vi "MASTER_-_Copy.vi"() -> ()   [LabVIEW 2019]
doc: "This is the interface, the one VI which loads all the others. Run this one first.\n\n(the line below ensures settings are saved)\n[Red Tweezers Save Settings]"
uses:
  subvis/line_trapping.ctl
  subvis/spot.ctl
  <vilib>/userdefined/High Color/IMAQdx.ctl
  subvis/selection_element.ctl
  <vilib>/Analysis/Matrix/Datatypes/RealMatrix.ctl
  subvis/mouse_info.ctl
  subvis/red_tweezers_globals_INTERNAL_VOLATILE.vi
  subvis/red_tweezers_globals.vi
  <vilib>/Analysis/Matrix/Numeric/Multiply/Multiply - RM,R.vi
  <vilib>/Analysis/baseanly.llb/Real A x B.vi
  <vilib>/Analysis/NI_AALBase.lvlib
  <vilib>/vision/driver/NI_Vision_Acquisition_Software.lvlib
  <vilib>/Analysis/Matrix/NI_Matrix.lvlib
  <vilib>/vision/NI_Vision_Development_Module.lvlib
panel:
  out "Objects":T1(array[cluster]) {"Aspect Ratio" format="%.2f"; "Orientation" format="%.2f"; "Area" format="%.2f"; "Object Center"."Y" format="%.2f"; "Object Center"."X" format="%.2f"}
  out "Specific Point 2":cluster{i32, i32}
  out "Specific Point":cluster{i32, i32}
  out "bottomrx 3":dbl
  out "toply 3":dbl
  out "bottomry 3":dbl
  out "toplx 3":dbl
  out "Circles 2":T2(array[cluster]) {"Position"."Y" format="%.2f"; "Position"."X" format="%.2f"}
  out "Spot Storage":T3[](array[typedef]) {"Amplitude Correction" step=0.1; "Line Trapping"."Phase Gradient" step=0.05; "Line Trapping"."Vector"."x" step=1e-06 format="%#_6p"; "Line Trapping"."Vector"."y" step=1e-06 format="%#_6p"; "Line Trapping"."Vector"."z" step=1e-06 format="%#_6p"; "NA Position"."r" step=1e-06; "NA Position"."y" step=1e-06; "NA Position"."x" step=1e-06; "Position"."z" step=1e-06; "Position"."y" step=1e-06; "Position"."x" step=1e-06; "Phase" step=0.7753; "Intensity" step=0.1}
  out "# selected":i16
  out "Last Pattern":T3[](array[typedef]) {"Amplitude Correction" step=0.1; "Line Trapping"."Phase Gradient" step=0.05; "Line Trapping"."Vector"."x" step=1e-06 format="%#_6p"; "Line Trapping"."Vector"."y" step=1e-06 format="%#_6p"; "Line Trapping"."Vector"."z" step=1e-06 format="%#_6p"; "NA Position"."r" step=1e-06; "NA Position"."y" step=1e-06; "NA Position"."x" step=1e-06; "Position"."z" step=1e-06; "Position"."y" step=1e-06; "Position"."x" step=1e-06; "Phase" step=0.7753; "Intensity" step=0.1}
  out "Plugins":T5(array[cluster])=[{"Name"="ASI Stage", "Folder"=path "C:/Users/Richard Bowman/Dropbox/red_tweezers_1_4_rc4/plugins/ASI Stage.llb", "vi reference"=refnum, "Needs to be run"=TRUE, "Error"={"status"=FALSE, "code"=0, "source"=""}}, {"Name"="iTweezers", "Folder"=path "C:/Users/Richard Bowman/Dropbox/red_tweezers_1_4_rc4/plugins/iTweezers.llb", "vi reference"=refnum, "Needs to be run"=TRUE, "Error"={"status"=FALSE, "code"=0, "source"=""}}, {"Name"="MightexLED", "Folder"=path "C:/Users/Richard Bowman/Dropbox/red_tweezers_1_4_rc4/plugins/MightexLED.llb", "vi reference"=refnum, "Needs to be run"=TRUE, "Error"={"status"=FALSE, "code"=0, "source"=""}}]
  in  "Tab":T6(tab)
  out "Possible Collision":bool
  out "Play Pressed":bool
  out "Y":dbl
  out "X":dbl
  in  "O Button":bool
  in  "OK Button":bool
  in  "Bubble Size":dbl=50.0002
  out "Hit Indicator":bool
  in  "On":bool
  out "Induce check":bool
  out "Area+ Buffer":dbl
  in  "Area to check":dbl=0.00025
  out "Prev Current Spot":dbl
  out "spots selected 2":i32=4
  out "Spot # Check":dbl
  out "Orig Y SC":dbl
  out "Orig X SC":dbl
  out "ID num check":dbl
  out "Value Check":dbl
  out "ID":dbl[](array[numeric])
  out "Null array":dbl[](array[numeric])
  out "Potential Collisions":dbl
  out "What to Check":dbl[](array[numeric])
  out "Num":dbl
  out "Old Y":dbl
  out "Old X":dbl
  out "init":dbl
  out "Looper":bool
  in  "Output to SLM":bool
  out "Maximum":dbl
  out "Projected Distance":dbl
  out "Previous Distance":dbl
  out "Group ID #":dbl
  in  "Buffer Zone":dbl=7e-05
  out "# of Spots":dbl
  out "Distance":dbl
  out "Hit":bool
  out "Y Displacement":dbl
  out "X Displacement":dbl
  out "Current Spot #":dbl
  out "spots selected":i32=4
  in  "lock aspect ratio":bool=TRUE
  in  "Size":cluster{"x":dbl, "y":dbl, "z":dbl} {"z" step=1e-06 format="%#_4p"; "y" step=1e-06 format="%#_4p"; "x" step=1e-06 format="%#_4p"}
  in  "Position":cluster{"x":dbl, "y":dbl, "z":dbl}={"x"=1e-06, "y"=-6.3e-06, "z"=0.0} {"z" step=1e-06 format="%#_4p"; "y" step=1e-06 format="%#_4p"; "x" step=1e-06 format="%#_4p"}
  in  "phase":dbl step=0.7753
  in  "Vortex Charge":i8
  in  "Intensity":dbl=1.0 step=0.1
  in  "add to selection":bool
  in  "random position":bool
  in  "new spot":bool
  in  "delete":bool
  in  "rotate":bool
  in  "Rotation Axis":u16(ring)=2 items=["Z", "X", "Y", "Custom"]
  in  "Angle (degrees)":dbl=2.0
  in  "Custom Axis":cluster{dbl, dbl, dbl}
  in  "Spot Shape":enum32{"Normal", "Line", "NA", "Mixed"}(tab)=enum."Mixed"
  in  "Line Trapping":T4 {"Phase Gradient" step=0.05; "Vector"."x" step=1e-06 format="%#_4p"; "Vector"."y" step=1e-06 format="%#_4p"; "Vector"."z" step=1e-06 format="%#_4p"}
  in  "Scale back aperture":dbl=1.1 step=0.1
  in  "Scale BA":bool
  in  "Position on back aperture":cluster{"x":dbl, "y":dbl}={"x"=-5.84327907697451e-18, "y"=0.0} {"y" step=0.1 format="%#_4p"; "x" step=0.1 format="%#_4p"}
  in  "Radius on back aperture":dbl=1.1 step=0.1
  in  "Generate":bool
  in  "Pattern":T7(tab)
  in  "Spots across centre":i32=5
  in  "Reference Array?":bool
  in  "Fraction of SLM":dbl=1.0
  in  "Spots across centre":i32=5
  in  "N":cluster{i32, i32}
  in  "spacing/m":dbl=2.0
  in  "Iterations":i32=10
  out "non-uniformity":dbl(slide)=0.031119223416512406 scale=0.0..0.2
  out "efficiency":dbl(slide)=0.8985936267644501 scale=0.0..1.0
  in  "Optimise":bool
  in  "Reset Phase/Amplitude":bool
  in  "Fall-off/m":dbl=0.00025 min=0.0 step=1e-06 format="%#_4p"
  in  "Abort Plugin":bool
  in  "Plugin:":u16(ring)=1
  in  "Save Video":bool
  in  "Global ROI (requires restart)":i32[](array[numeric])=[0, 0, 1280, 512]
  in  "Zoom":bool
  in  "Draw ROI":bool
  in  "Zoom to Fit":bool
  out "Image Information":string="640x480 1.93X 8-bit image 255    (0,0)"
  in  "Camera":T8
  in  "Time per Frame (ms)":dbl
  in  "Edit Sequence Mode":bool
  in  "Manual Edit":bool
  in  "Bubble ID to Empty":dbl
  in  "Clearance Button":bool
  in  "Manual Sequence":bool
  in  "Play Sequence":bool
  in  "Reset":bool
  out "Sequence Instances":dbl
  out "Counter":dbl
  in  "Save State":bool
  out "Sequence On?":bool
  in  "Sequence Order":dbl
  out "Selection/Group":T9[](array[typedef])
  in  "Sequence Storer":T3[][](array[typedef]) {"Amplitude Correction" step=0.1; "Line Trapping"."Phase Gradient" step=0.05; "Line Trapping"."Vector"."x" step=1e-06 format="%#_6p"; "Line Trapping"."Vector"."y" step=1e-06 format="%#_6p"; "Line Trapping"."Vector"."z" step=1e-06 format="%#_6p"; "NA Position"."r" step=1e-06; "NA Position"."y" step=1e-06; "NA Position"."x" step=1e-06; "Position"."z" step=1e-06; "Position"."y" step=1e-06; "Position"."x" step=1e-06; "Phase" step=0.7753; "Intensity" step=0.1}
  in  "New location\n ROI":bool
  out "Radius ROI x6":dbl
  out "Radius ROI y6":dbl
  out "Radius ROI y5":dbl
  out "Radius ROI x5":dbl
  out "Radius ROI y4":dbl
  out "Radius ROI x4":dbl
  out "Radius ROI y3":dbl
  out "Radius ROI x3":dbl
  out "Radius ROI x2":dbl
  out "Radius ROI y2":dbl
  out "Radius ROI y1":dbl
  out "Radius ROI x1":dbl
  out "Caging Radius \nToo Big":bool
  in  "Caging Radius":dbl
  out "ROI Point 1":T10
  out "ROI Point 0":T10
  out "ROI Point 2":T10
  in  "New Center Y":dbl
  in  "New Center X":dbl
  out "Delta x":dbl[](array[numeric])
  out "Delta y":dbl[](array[numeric])
  in  "Input New \nObject Location":bool
  out "Time Elapsed(ms)":i32
  out "Start":i32
  out "Stop":i32
  out "Insert End":bool
  out "NewXYRates":dbl[][](array[numeric])
  out "NewXYArraySize":dbl
  out "NewXYArray":dbl[][](array[numeric])
  in  "Rates":dbl
  out "LCS Y":dbl
  out "LCS X":dbl
  in  "LCS":dbl
  in  "Play":bool
  out "Initiate Creation":dbl
  in  "Max Number \nof Bubbles":dbl
  in  "Number of Planned\nSequence Frames":dbl
  in  "Add Additional Frames":bool
  in  "Frame Location":dbl
  in  "Additional Frames Wanted":dbl
  in  "Tab Control":enum32{"Line", "Arc"}(tab)
  out "X Rate":dbl
  out "Y Rate":dbl
  out "Original D-Y":dbl
  out "Original D-X":dbl
  out "Original Radius":dbl
  out "Center Location":dbl[][](array[numeric])
  out "Center X":dbl
  out "Center Y":dbl
  out "ROI Y":dbl
  out "ROI X":dbl
  out "Original Theta":dbl
  out "Degree Rate":dbl
  in  "Lock Current Spot":bool
  out "Locked Current Spot":dbl
  out "Numeric":dbl
  out "probe":dbl
  in  "Insert":bool
  in  "Start at Which Frame?":dbl
  out "Original Y":dbl
  out "Original X":dbl
  in  "Mark Original Position":bool
  in  "How Many Frames?":dbl
  out "New Y":dbl
  out "New X":dbl
  out "Spot Storage 2":T3[](array[typedef]) {"Amplitude Correction" step=0.1; "Line Trapping"."Phase Gradient" step=0.05; "Line Trapping"."Vector"."x" step=1e-06 format="%#_6p"; "Line Trapping"."Vector"."y" step=1e-06 format="%#_6p"; "Line Trapping"."Vector"."z" step=1e-06 format="%#_6p"; "NA Position"."r" step=1e-06; "NA Position"."y" step=1e-06; "NA Position"."x" step=1e-06; "Position"."z" step=1e-06; "Position"."y" step=1e-06; "Position"."x" step=1e-06; "Phase" step=0.7753; "Intensity" step=0.1}
  in  "Save":bool
  in  "Load":bool
  out "Current Y":dbl
  out "Current X":dbl
  out "Object MP Y":dbl
  out "Object MP X":dbl
  out "ROI Point 3":T10
  out "Numeric 3":dbl
  out "Numeric 2":dbl
  in  "ROI points":dbl
  out "ROI Y":dbl
  out "ROI X":dbl
  out "Center Y":dbl
  out "Center X":dbl
  in  "Camera Capture 2":bool
  out "Bubble y 2":dbl
  out "Bubble x 2":dbl
  out "Number of Matches Returned":dbl
  out "bottomry 2":dbl
  out "toply 2":dbl
  out "bottomrx 2":dbl
  out "toplx 2":dbl
  in  "Send Data":bool
  out "Camera 3":T11(plugin-control)
  in  "Circle Descriptor 2":cluster{"Min Radius":dbl, "Max Radius":dbl}={"Min Radius"=3.0, "Max Radius"=500.0}
  out "Radius":dbl
  in  "Settings":T12={"Objects"=0, "Threshold"=128, "Reject Border"=FALSE, "Fill Holes"=FALSE, "Min Object Size"=FALSE, "Min Size"=3, "Max Object Size"=FALSE, "Max Size"=100, "Show Search Area"=FALSE, "Show Center"=TRUE, "Show Bounding Box"=TRUE} {"Objects" items=["Bright Objects", "Dark Objects"]; "Threshold" min=1 max=999999999 step=1; "Max Size" min=1 max=999999999 step=1; "Min Size" min=1 max=999999999 step=1}
  out "Number of Objects":i32
  in  "ROI switch":bool
  out "# of pairs":dbl
  out "Video Frame Rate":dbl(knob)=50.00000000000003 scale=0.0..100.0 scale format="%.1f"
  out "Interface Frame Rate":dbl(knob)=97.23240312927678 scale=0.0..100.0 scale format="%.1f"
  in  "stop":bool=TRUE
  out "Step Calculation Y2":dbl
  out "Step Calculation Y1":dbl
  out "Step Calculation X2":dbl
  out "Step Calculation X1":dbl
  out "NewY2":dbl
  out "NewX2":dbl
  out "NewY1":dbl
  out "NewX1":dbl
  out "3spot Y":dbl
  out "3spot X":dbl
  out "2spot Y":dbl
  out "2spot X":dbl
  out "1spot Y":dbl
  out "1spot X":dbl
  in  "Spots":dbl
  out "ROI new Mpy":dbl
  out "ROI new MPx":dbl
  out "ROI y6":dbl
  out "ROI x6":dbl
  out "ROI y5":dbl
  out "ROI x5":dbl
  out "ROI y4":dbl
  out "ROI x4":dbl
  out "ROI y3":dbl
  out "ROI x3":dbl
  out "ROI y2":dbl
  out "ROI x2":dbl
  out "ROI y1":dbl
  out "ROI x1":dbl
  out "ROI Point 6":T10
  out "ROI point 5":T10
  out "ROI Point 4":T10
  out "MOP pressed":bool
  out "MOP pressed After":bool
  out "X Pos every 10 sec":dbl
  out "Elapsed Time":dbl
  out "Position Indicator":string
  out "Spot Checker":T3[](array[typedef]) {"Amplitude Correction" step=0.1; "Line Trapping"."Phase Gradient" step=0.05; "Line Trapping"."Vector"."x" step=1e-06 format="%#_6p"; "Line Trapping"."Vector"."y" step=1e-06 format="%#_6p"; "Line Trapping"."Vector"."z" step=1e-06 format="%#_6p"; "NA Position"."r" step=1e-06; "NA Position"."y" step=1e-06; "NA Position"."x" step=1e-06; "Position"."z" step=1e-06; "Position"."y" step=1e-06; "Position"."x" step=1e-06; "Phase" step=0.7753; "Intensity" step=0.1}
  out "Image":T11(plugin-control)
  # "Notes:\n\nIf you are doing non-sequence controls,\nthe delete function can be used as intended.\nHowever, do not use the delete function after\nrunning a sequence! Using it will prevent\nthe bubbles from appearing as the\nnumber of spots will change, which is\nessential for the sequence to work (it would\nbe displaying the maximum number of\nbubbles). \n\nIf you happen to delete a bubble, it can be \nrestored by inserting a new spot. Once enough\nspots have been restored, click on manual edit\nto correct the # of spots tracker. It should \nbe restored to where it originally was."
  # "The SLM can be used to shape spots; here you can restrict the NA of a spot (so it comes only from part of the back aperture), or create a line-trap"
  # "The traps do not have any spot-shaping applied (so they should just be diffraction-limited focal spots)."
  # "This shapes the amplitude (and phase) of the beam to create extended line traps.  The \"Phase Gradient\" control allows the Poynting vector to push things along the line.  Unfortunately, some work is needed on the scaling factors so the phase gradient control will need tweaking if the line trap has a nonzero z component."
  # "By default,each spot comes from the whole back aperture.  Here, you can limit a spot to come from a specific part of the back aperture."
  # "The control below allows you to scale the whole back aperture (i.e. the position and size of all the apertures).  It's a one-time operation, i.e. only changes things when you push \"ok\"."
  # "A Combination of line-trapping and NA restriction has been applied to these traps.  You can get at the line trap or NA parameters on the other tabs, switching to the NA tab does not delete the line-trap settings."
  # "This tab generates Shack-Hartmann type holograms, which are often useful when aligning the system, and arrays of spots."
  # "The controls above only work when using the \"IMAQdx with ROI Buttons\" case in the bottom loop.  You can save video regardless of camera code though."
  # "Manual Edit allows a user to\ngo to a specific sequence frame."
  # "To clear the sequence, you must\nclear the array. Right click on sequence\nstorer to do this."
  # "Use this to \"clear\" a \nspecific bubble. If\nworking on a sequence,\nuse this as your delete\nbutton! You can update\nthe view by using manual edit."
  # "Use the reset button\nto clear counter.\nIt becomes necessary\nwhen you clear the array,\nespecially in manual mode."
  # "Use the sequence creator tab to specify the\nnumber of bubbles you want along with\nthe number of frames.\n\nTo save at a specific interval, the sequence\norder can be used to place the state. If used\nto correct something, it will replace the\nentire sequence frame.\n\n\"Sequence On?\" is only used in auto mode."
  # "Multiple bubbles can  be done with the\nline function. One bubble at a time for the arc\nfunction."
  # "Using the Load/Save function:\n\nRed Tweezers itself is unable to save long \nsequences, but a separate program is able to\naccomplish this. To do this, follow these\nsteps:\n\n1. After creating your sequence, press the save\nbutton below.\n\n2. Then, go to the subvi folder and find\nSequenceSaver.vi.\n\n3. At the control \"Sequence Storer,\" right-click\nthe dimensions part of the array and go to\ndata operations.\n\n4. Press \"Make Current Values Default\" and save\nthe sequence.\n\n5. The next time you load the program, simply\npress load to re-acquire the sequence. You\nwill need to insert the bubbles again, but after\nthe first frame can be recovered by using\nSequenceControl.vi."
types:
  T1 = cluster{"Object Center":cluster{"X":sgl, "Y":sgl}, "Bounding Box":cluster{"X Left":i32, "Y Top":i32, "X Right":i32, "Y Bottom":i32}, "Area":sgl, "Orientation":sgl, "Aspect Ratio":sgl, "Nb Holes":i32}[]
  T2 = cluster{"Position":cluster{"X":sgl, "Y":sgl}, "Radius":dbl, "Score":dbl}[]
  T3 = typedef "spot.ctl" = cluster{"Position":cluster{"x":dbl, "y":dbl, "z":dbl}, "Intensity":dbl, "Vortex Charge":i8, "Phase":dbl, "NA Position":cluster{"x":dbl, "y":dbl, "r":dbl}, "Line Trapping":T4, "Amplitude Correction":dbl}
  T4 = typedef "line_trapping.ctl" = cluster{"Vector":cluster{"x":dbl, "y":dbl, "z":dbl}, "Phase Gradient":dbl}
  T5 = cluster{"Name":string, "Folder":path, "vi reference":refnum<vi>, "Needs to be run":bool, "Error":errorcluster}[]
  T6 = enum32{"Current Spot", "Rotate", "Spot Shape", "Patterns", "Plugins", "Video", "Sequence", "Sequence Creator", "Spot Control", "Load/Save", "Image Process"}
  T7 = enum32{"HCP Shack-Hartmann", "Square Shack-Hartmann", "Rectangular Grid"}
  T8 = typedef "IMAQdx.ctl" = refnum<k21>
  T9 = typedef "selection_element.ctl" = cluster{"Group ID":i32, "Selected":bool}
  T10 = typedef "NI_Matrix.lvlib/RealMatrix.ctl" = dbl[][]
  T11 = typedef "IMAQ Image.ctl" = refnum<image>
  T12 = cluster{"Objects":u16, "Threshold":i32, "Reject Border":bool, "Fill Holes":bool, "Min Object Size":bool, "Min Size":i32, "Max Object Size":bool, "Max Size":i32, "Show Search Area":bool, "Show Center":bool, "Show Bounding Box":bool}
  T13 = typedef "mouse_info.ctl" = cluster{"Button Down":bool, "Dragging":bool, "Position (Image Pixels)":cluster{"X":dbl, "Y":dbl}, "Previous Position (Image Pixels)":cluster{"X":dbl, "Y":dbl}, "Button":u16, "Mods":cluster{"Double Click":bool, "Menu Key":bool}, "PlatMods":cluster{"Shift":bool, "Ctrl":bool, "Alt":bool, "Cmd":bool, "Opt":bool}}
  T14 = cluster{"Desired Font (Application)":enum16{"User-specified Font", "Application Font", "System Font", "Dialog Font"}, "[User-specified Font]":cluster{"Font Name":string, "Size":i16, "Strikeout?":bool, "Italic?":bool, "Underline?":bool, "Outline?":bool, "Shadow?":bool, "Bold?":bool, "Rotation Angle":dbl}, "Horizontal Alignment":i16, "Vertical Alignment":i16}
  T15 = cluster{"Position":cluster{"x":dbl, "y":dbl, "z":dbl}, "Intensity":dbl, "Vortex Charge":i8, "Phase":dbl, "NA Position":cluster{"x":dbl, "y":dbl, "r":dbl}, "Line Trapping":T4, "Amplitude Correction":dbl}
  T16 = enum16{"Set guide visibility", "Set grid visibility", "Show front panel", "Render on image"}
  T17 = enum32{"Current Spot", "Rotate", "Spot Shape", "Patterns", "Plugins", "Video"}
  T18 = enum16{"Left Button", "Center Button", "Right Button", "Window Close"}
  T19 = typedef "Image Type" = u32
  T20 = cluster{"number: 0 to 1":dbl, "number: 0 to 1":dbl}
  T21 = typedef "overlay_element.ctl" = cluster{"Tool":enum16{"Lines", "Oval", "Rectangle", "Text"}, "Points":cluster{"X":dbl, "Y":dbl}[], "Drawing Mode":u32, "Color":u32, "String":string}
  T22 = enum32{"Current Spot", "Rotate", "Spot Shape", "Patterns", "Plugins", "Video", "Particle Tracking", "Clamping", "Blank"}[]
  T23 = typedef "LVMenuShortCut.ctl" = cluster{"include Shift key?":bool, "include Ctrl key?":bool, "shortcut key":string}
  T24 = typedef "LVPoint32TypeDef.ctl" = cluster{"Horizontal":i32, "Vertical":i32}
  T25 = cluster{"Shift":bool, "Ctrl":bool, "Alt":bool, "Cmd":bool, "Opt":bool}
  T26 = cluster{"Button Down":bool, "Dragging":bool, "Mouse Coords (image pixels)":cluster{dbl, dbl}, "Mouse Coords (image pixels)":cluster{dbl, dbl}, "Button":u16, "Mods":cluster{"Double Click":bool, "Menu Key":bool}, "PlatMods":cluster{"Shift":bool, "Ctrl":bool, "Alt":bool, "Cmd":bool, "Opt":bool}}
  T27 = cluster{"Position":cluster{"X":sgl, "Y":sgl}, "Radius":dbl, "Score":dbl}
  T28 = cluster{"Global Rectangle":i32[], "Contours":cluster{"Contour Type":u32, "ROI Type":u32, "Points":i32[]}[]}
  T29 = cluster{"Contour Type":u32, "ROI Type":u32, "Points":i32[]}[]
  T30 = cluster{"Contour Type":u32, "ROI Type":u32, "Points":i32[]}
  T31 = cluster{"[0]":dbl, "[1]":dbl, "[2]":dbl, "[3]":dbl}
  T32 = cluster{"Object Center":cluster{"X":sgl, "Y":sgl}, "Bounding Box":cluster{"X Left":i32, "Y Top":i32, "X Right":i32, "Y Bottom":i32}, "Area":sgl, "Orientation":sgl, "Aspect Ratio":sgl, "Nb Holes":i32}
  T33 = cluster{"Position":cluster{"x":dbl, "y":dbl, "z":dbl}, "Intensity":dbl, "Vortex Charge":i8, "Phase":dbl, "NA Position":cluster{"x":dbl, "y":dbl, "r":dbl}, "Line Trapping":T4, "Amplitude Correction":dbl}[]
  T34 = cluster{"NewXYArray[0]":dbl, "NewXYArray[1]":dbl, "NewXYArray[2]":dbl, "NewXYArray[3]":dbl, "NewXYArray[4]":dbl, "NewXYArray[5]":dbl, "NewXYArray[6]":dbl, "NewXYArray[7]":dbl, "NewXYArray[8]":dbl}
  T35 = cluster{"Average Frame Time":dbl, "millisecond timer value":u32}
  T36 = enum32{"Bad", "Idle", "Run top level", "Running"}
  T37 = typedef "AviRefnum.ctl" = refnum<k1>
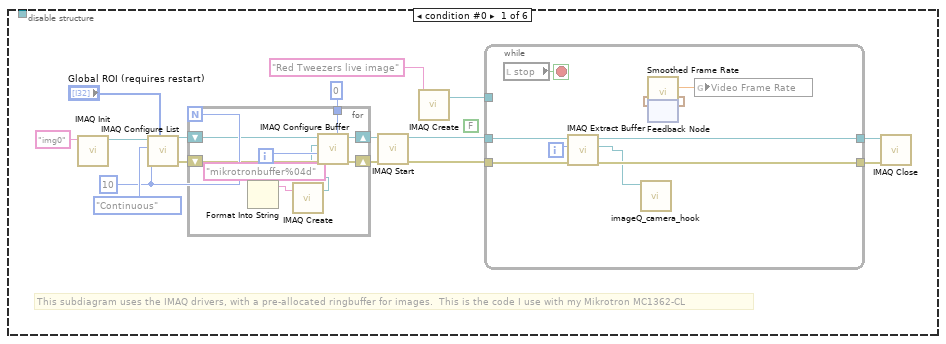
[diagram p3: hidden frame]
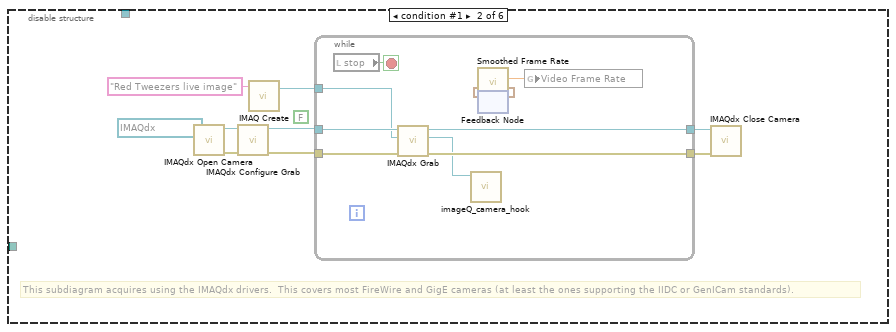
[diagram p4: hidden frame]
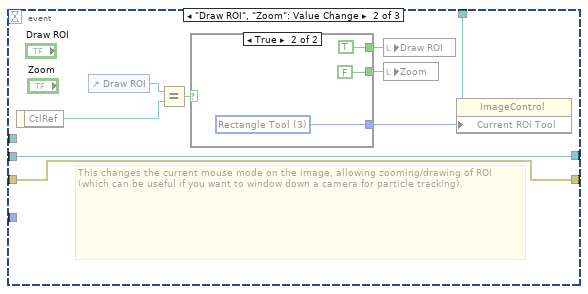
[diagram p5: hidden frame]
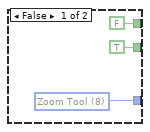
[diagram p6: hidden frame]
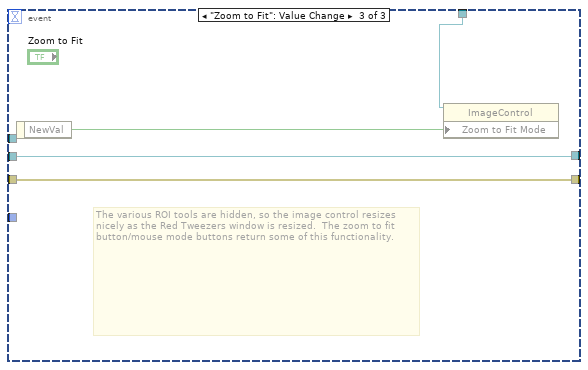
[diagram p7: hidden frame]
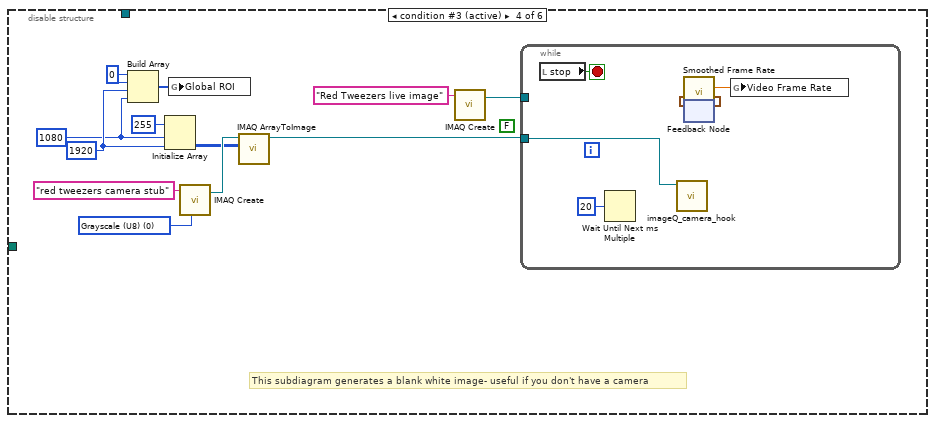
[diagram p8: hidden frame]
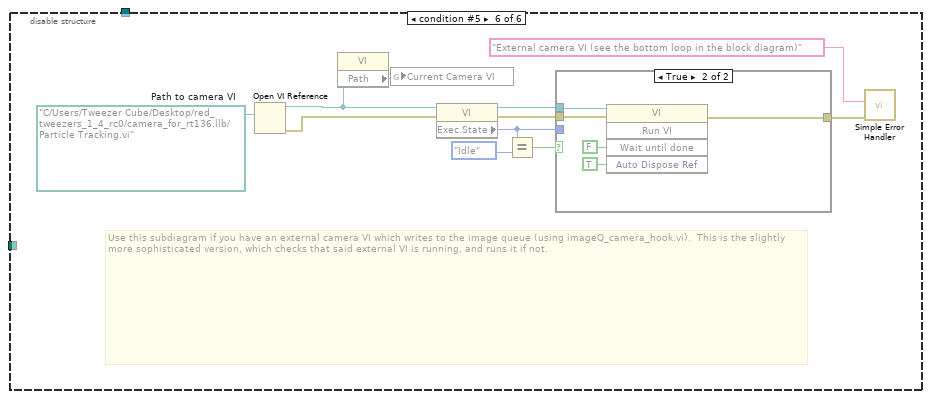
[diagram p10: hidden frame]
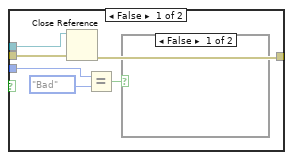
[diagram p11: hidden frame]
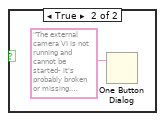
[diagram p12: hidden frame]
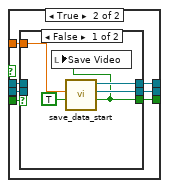
[diagram p14: hidden frame]
diagram:
  w11 = "red_tweezers_display_imageQ" ("Queue Name")
  w23 = T13 {"Button Down"=FALSE, "Dragging"=FALSE, "Position (Image Pixels)"={"X"=0.0, "Y"=0.0}, "Previous Position (Image Pixels)"={"X"=0.0, "Y"=0.0}, "Button"=0, "Mods"={"Double Click"=FALSE, "Menu Key"=FALSE}, "PlatMods"={"Shift"=FALSE, "Ctrl"=FALSE, "Alt"=FALSE, "Cmd"=FALSE, "Opt"=FALSE}}  # Mouse Information
  w24 = refnum<vi> refnum  # Image
  # "The funny looking feedback-node structure is deliberate (if odd).  We want to reload settings from the last used file (stored in the registry) only if this program has not been run since it was last loaded from file/recompiled.  That's why I use an uninitialised shift register: every time the program runs, it increments.  So, if it is zero, this is our first run (or we've been recently recompiled)."
  # "This loop handles the video that is displayed on-screen and saved to file."
  # "Initially, we only register to be told when the user clicks the image"
  # "This is the actual image control"
  # "This is a generic reference.\nIt is just a placeholder, so we can register for events later."
  # "This version of red tweezers uses two coordinate systems: \n1. Real Coordinates - corresponding to physical distances in 3D in microns\n2. Image Coordinates - position on the camera image, relative to the top left of the CURRENT ROI, measured in pixels. If the ROI changes, the relationship between \"real units\" and \"image pixels\" may change, so all values should be stored and presented to the user in REAL units unless there is a good reason to do otherwise."
  n1 = control-ref of="Plugin Pnl"() -> (w20:refnum<vi>)
  n2 = flat-sequence {
    tunnel: [w27] -> w6
    tunnel: w4 -> [_]
    frame #0 {
      n3 = vi-ref "red_tweezers_globals_INTERNAL.vi"() -> (w28:refnum<vi>)
      n4 = property class="VI"(reference=w28) -> ("Path"=w27:path)  [unwired: 1 in, 2 out]
      n5 = global write "red_tweezers_globals_INTERNAL_VOLATILE.vi" "Current Camera VI"(w27) -> ()
    }
  }
  n6 = control-ref of="Plugin:"() -> (w21:refnum<vi>)
  n7 = feedback #1() -> (w14:dbl)  [unwired: 1 in]
  n8 = Equal To 0?(x=w14) -> (x = 0?=w13:bool)
  n9 = Increment(x=w14) -> (x+1=w12:dbl)
  n10 = feedback-in #1(w12) -> ()
  n11 = call "plugins_load.vi"("Sub Panel"=w20, "Plugin Chooser"=w21) -> ("error out"=w15:errorcluster, "Plugins"=w17:T5)  [unwired: 2 in, 2 out]
  "Plugins" <- w17
  n12 = control-ref of="Image"() -> (w5:refnum<vi>)
  n13 = case shown="True" w13 {
    tunnel: w15 -> [_ w29]
    tunnel: [_ w29] -> w4
    frame False {
    }
    frame True {
      n14 = call "settings_load_default_file.vi"("error out"=w29) -> ()
    }
  }
  n15 = flat-sequence {
    tunnel: w4 -> [_]
    tunnel: w2 -> [w31]
    frame #0 {
      # "ensure we don't accidentally start saving video, and run UDP Sender to set up the hologram window."
      n16 = local write "Save Video"(FALSE ("background subtraction")) -> ()
      n17 = call "UDP Sender generic_2.vi"("Spots"=w31) -> ()  [unwired: 2 in, 1 out]
    }
  }
  n18 = global read "red_tweezers_globals.vi" "Selection/Group"() -> (w22:T9[])
  n19 = register-events(w5, w24, w24, w24) -> (reference out=w25:refnum<event-registration>)  [unwired: 2 in, 1 out]
  n20 = global read "red_tweezers_globals.vi" "Spots"() -> (w2:T3[])
  n21 = local write "stop"(FALSE ("STOP")) -> ()
  n22 = call "ensure_selection_matches_spots.vi"("Selection and Groups in"=w22, "Spots"=w2) -> ("Selection and Groups out"=w26:T9[], "Spots (duplicate)"=w1:T3[])  [unwired: 4 in]
  n23 = call "IMAQ Create"("Image Name"=w11) -> ("New Image"=w9:T11)  [unwired: 4 in, 1 out]
  n24 = call "imageQ_create_return_queue.vi"("Queue Name"=w11) -> ("queue out"=w10:refnum<queue>)
  n25 = while {
    shift-right: [w153] -> _
    shift-left: w1 -> [w173]
    shift-right: [w172] -> _
    shift-left: w26 -> [w171]
    shift-right: [w175] -> _
    shift-left: _ -> [w166]
    shift-right: [w174] -> _
    shift-left: _ -> [w165]
    tunnel: w5 -> [w170]
    shift-right: [w164] -> _
    shift-left: w23 -> [w163]
    shift-right: [w167] -> _
    shift-left: w25 -> [w168]
    border: errorcluster {"status"=FALSE, "code"=0, "source"=""} ("error out") -> [_]
    tunnel: [errorcluster {"status"=FALSE, "code"=0, "source"=""} ("error in (no error)")] -> w18
    border: w17 -> [_]
    tunnel: w1 -> [w154]
    stop <- w155 stop-if-true
    (unwired) 1 ("index")
    w72 = 7 items=["Red", "Green", "Blue", "Hue", "Saturation", "Luminance", "Value", "Intensity"] ("Color Plane")
    w74 = T19 0 items=["Grayscale (U8)", "Grayscale (I16)", "Grayscale (SGL)", "Complex (CSG)", "RGB (U32)", "HSL (U32)", "RGB (U64)", "Grayscale (U16)"] ("Image Type")
    # "Old play function that goes into case structure when\nInput New Object Location is False, using this case structure\nto prevent code from being actiivated for now"
    # "Pressing play is supposed to cause the program to\nsendcoordinates to Sequence Storer, which is\nused by SequenceControl to move the bubble, \nhowever this does not work at the moment"
    # "When done obtatining points\nKEEP it at 7!"
    # "Cycle through to obtain points"
    # "This is the calculation for the center of the detected circle, not sure where to put for now"
    # "This Play Function inserts bubbles from a given .mat file into the sequence storer"
    # "The function inserts the newly generated sequence for the automatic sequence generator. It also contains the code\nthe code necessary to check whether the bubbles will intersect with each other in the sequence."
    # "This calculates the size of the area including the buffer zone length.\nThe bubble diameter will also be included in the near future."
    # "The statement to the right controls the area that are being chcecked and checks\nwhich bubbles need to be checked.  There are two instances where this activates\nin this case:\n\nWhen a new bubble is selected\nWhen a bubble is deselected, reverting to the last current spot #\n\nThe other case, when the bubble moves out of the area specified, is located\ninside the while loop controlling the bubble movement with a mouse."
    # "Timer function example"
    # "These functions help with the calculations for the sequence generator."
    # "This loads the sequence from the \"saver\" VI. The save function below \"saves\" the sequence into the saver VI."
    # "The VI above is SequenceSaver.vi which contains the\ncode necessary to create a sequence."
    # "This case structure is the Save State structure. This stores\nthe current state of the bubbles (ie position)."
    # "Reset sets the counter back to zero. This is particularly useful \nwhen using the manual sequence."
    # "This case structure helps to continue the sequence.\nThis takes the true case of the Sequence On? function\nor the true case for the Manual Sequence function\nin order to go to the next sequence frame."
    # "This case structure allows for the playing of the sequence.\nThe amount of time it takes to go through the sequence\ncan be edited on the current spot menu."
    # "We only write to the image overlay when we are in one of the tabs, to prevent it disappearing when we are (for example) using the mouse."
    # "These wires control saving undo info. See the VI below's tip strips for details."
    # "Setting these wires to false means:\n(1) dragging moves the selection\n(2) clicking spots changes selection\nset them to true to stop the default mouse behaviour, don't wire them straight through!"
    n26 = event shown="[6] <Image>: Mouse Move" {
      selector: w168 -> [w901 w1582 w1587 w1809 w1837 w1854 w1951 _]
      dyn-events: [w901 w1581 w1587 w1807 w1834 w1855 w1951 _] -> w167
      timeout: 0 -> [_ _ _ _ _ _ _ _]
      tunnel: [w909 _ w1589 w1804 w1839 w1846 w1938 _] -> w175
      tunnel: [w908 _ w1588 w1803 w1838 w1845 w1942 _] -> w174
      tunnel: [w907 _ _ _ _ _ _ _] -> w126
      tunnel: w173 -> [w906 w1577 w1594 w1799 w1832 w1851 w1946 w2269]
      tunnel: [w905 w1577 w1592 w1799 w1832 w1842 w1944 w2269] -> w161
      tunnel: [w904 w1576 w1591 w1788 w1831 w1852 w1934 w2268] -> w160
      tunnel: w171 -> [w903 w1576 w1593 w1788 w1831 w1850 w1945 w2268]
      tunnel: w170 -> [w902 w1578 w1584 w1798 w1835 w1853 w1947 _]
      tunnel: [w900 _ w1586 w1808 T13 {"Button Down"=FALSE, "Dragging"=FALSE, "Position (Image Pixels)"={"X"=0.0, "Y"=0.0}, "Previous Position (Image Pixels)"={"X"=0.0, "Y"=0.0}, "Button"=0, "Mods"={"Double Click"=FALSE, "Menu Key"=FALSE}, "PlatMods"={"Shift"=FALSE, "Ctrl"=FALSE, "Alt"=FALSE, "Cmd"=FALSE, "Opt"=FALSE}} T13 {"Button Down"=FALSE, "Dragging"=FALSE, "Position (Image Pixels)"={"X"=0.0, "Y"=0.0}, "Previous Position (Image Pixels)"={"X"=0.0, "Y"=0.0}, "Button"=0, "Mods"={"Double Click"=FALSE, "Menu Key"=FALSE}, "PlatMods"={"Shift"=FALSE, "Ctrl"=FALSE, "Alt"=FALSE, "Cmd"=FALSE, "Opt"=FALSE}} w1950 _] -> w164
      tunnel: w163 -> [w900 _ w1586 _ _ w1849 w1941 _]
      tunnel: w166 -> [_ _ w1589 w1804 w1839 w1846 w1938 _]
      tunnel: w165 -> [_ _ w1588 w1803 w1838 w1845 w1942 _]
      tunnel: [w899 _ _ _ _ _ _ _] -> w162
      tunnel: [_ _ w1585 _ _ _ TRUE _] -> w159
      tunnel: [_ _ _ TRUE TRUE TRUE FALSE _] -> w158
      tunnel: [TRUE _ _ _ _ _ _ _] -> w156
      tunnel: [_ _ _ _ _ _ _ "stop"] -> w155
      tunnel: w154 -> [_ _ _ _ _ _ w1935 _]
      event Timeout {
        n27 = event-data() -> ()  [unwired: 1 in, 1 out]
        n28 = case shown="\"Image Process\"" "Tab" {
          tunnel: [w924 w1192 w1339 w1441 w1522 w1560 w1562 w1564 w1566 w1568 w1570] -> w905
          tunnel: w906 -> [w921 w1194 w1340 w1443 w1522 w1560 w1562 w1564 w1566 w1568 w1570]
          tunnel: w903 -> [w910 w1193 w1337 w1442 w1521 w1559 w1561 w1563 w1565 w1567 w1569]
          tunnel: [w923 w1191 w1338 w1440 w1521 w1559 w1561 w1563 w1565 w1567 w1569] -> w904
          tunnel: [w911 _ TRUE _ _ _ _ _ _ _ _] -> w909
          tunnel: [w911 _ _ _ _ _ _ _ _ _ _] -> w908
          tunnel: [_ _ _ FALSE _ _ _ _ _ _ _] -> w907
          tunnel: w902 -> [_ _ _ _ _ w1556 _ _ _ _ _]
          tunnel: w900 -> [_ _ w1319 _ _ _ _ _ _ _ _]
          tunnel: [_ _ w1321 _ _ _ _ _ _ _ _] -> w899
          frame "Current Spot", Default {
            w911 = FALSE
            # "The function below contains the code necessary to use the automatic sequence generator to create specific movements. It also helps translate cases where the point is entered in not dragged.\nThis prevents bubbles from intersecting if the bubble is told not to intersect."
            # "If it's out of date, update front panel"
            n29 = call "find_centroid.vi"("Selection and Groups"=w910, "Spots"=w921) -> ("Mean Values"=w919:T3, "size"=w913:cluster{"x":dbl, "y":dbl, "z":dbl}, "centroid"=w914:cluster{"x":dbl, "y":dbl, "z":dbl}, "# selected"=w912:i16)  [unwired: 2 in, 1 out]
            n30 = stacked-sequence {
              tunnel: w912 -> [_ w926]
              frame #0 {
                n31 = local read "spots selected"() -> (→"spots selected 2":i32)
              }
              frame #1 {
                "spots selected" <- w926
              }
            }
            n32 = feedback-in #2(w919) -> ()
            n33 = feedback #2() -> (w920:T3)  [unwired: 1 in]
            n34 = feedback #3() -> (w918:cluster{"x":dbl, "y":dbl, "z":dbl})  [unwired: 1 in]
            n35 = feedback-in #3(w913) -> ()
            n36 = Not Equal?(x=w920, y=w919) -> (x != y?=w917:bool)
            n37 = Not Equal?(x=w918, y=w913) -> (x != y?=w916:bool)
            n38 = Or(x=w917, y=w916) -> (x .or. y?=w915:bool)
            n39 = case shown="True" w915 {
              tunnel: w919 -> [_ w932]
              tunnel: w913 -> [_ w928]
              frame False {
              }
              frame True {
                n40 = Unbundle By Name(w932) -> ("Position"=w927:cluster{"x":dbl, "y":dbl, "z":dbl}, "Intensity"=w930:dbl, "Vortex Charge"=w929:i8, "Phase"=w931:dbl)
                n41 = local write "Size"(w928) -> ()
                n42 = local write "Vortex Charge"(w929) -> ()
                n43 = local write "Intensity"(w930) -> ()
                n44 = local write "Position"(w927) -> ()
                n45 = local write "phase"(w931) -> ()
                n46 = Unbundle By Name(w927) -> ()  [unwired: 2 out]
              }
            }
            n47 = local write "Selection/Group"(w910) -> ()
            n48 = event shown="[5] \"Intensity\": Value Change" {
              selector: _ -> [_ _ _ _ _ _ _ _]
              dyn-events: _ -> [_ _ _ _ _ _ _ _]
              timeout: 10 -> [_ _ _ _ _ _ _ _]
              tunnel: w921 -> [w934 w938 w952 w975 w1079 w1124 w1150 w1173]
              tunnel: w910 -> [w933 w937 w955 w982 w1066 w1121 w1147 w1171]
              tunnel: [w934 w936 w953 w974 w1067 w1122 w1148 w1172] -> w924
              tunnel: [w933 w935 w954 w982 w1066 w1121 w1147 w1171] -> w923
              tunnel: w914 -> [_ _ _ _ w1078 _ _ _]
              event Timeout {
                n49 = event-data() -> ()  [unwired: 3 out]
              }
              event "delete": Value Change {
                n50 = event-data() -> ()  [unwired: 7 out]
                n51 = call "delete_selected_spots.vi"("Selection/Group 3"=w937, "Spots 3"=w938) -> ("Selection/Group 2"=w935:T9[], "Spots 2"=w936:T3[])  [unwired: 4 in]
              }
              event "new spot": Value Change {
                # "If we're not adding it to the selection, de-select all the other spots"
                n52 = event-data() -> ()  [unwired: 7 out]
                n53 = call "coords_ROI_currentimage.vi"() -> ("Mono ROI"=w939:i32[])
                n54 = case shown="False" "add to selection" {
                  tunnel: w955 -> [w968 w973]
                  tunnel: [w967 w973] -> w950
                  frame False {
                    n55 = for {
                      tunnel: w968 -> [w971] mode=indexing
                      tunnel: [w972] -> w967 mode=indexing
                      n56 = Unbundle(w971) -> ("Group ID"=w970:i32)  [unwired: 1 out]
                      n57 = Bundle(cluster=w971, "Group ID"=w970, "Selected"=FALSE ("Label.Visible")) -> (w972:T9)
                    }
                  }
                  frame True {
                  }
                }
                n58 = Index Array(array=w939) -> (element #1=w945:i32, element #2=w946:i32, element #3=w944:i32, element #4=w943:i32)  [unwired: 4 in]
                n59 = Bundle("Numeric"=w945, "Numeric"=w946) -> (w940:cluster{"Numeric":i32, "Numeric":i32})  [unwired: 1 in]
                n60 = Bundle("Numeric"=w944, "Numeric"=w943) -> (w942:cluster{"Numeric":i32, "Numeric":i32})  [unwired: 1 in]
                n61 = Subtract(x=w942, y=w940) -> (x-y=w941:cluster{"Numeric":i32, "Numeric":i32})
                n62 = case shown="True" "random position" {
                  tunnel: [w957 w963] -> w948
                  tunnel: w941 -> [_ w959]
                  tunnel: w940 -> [_ w958]
                  frame False {
                    n63 = call "replace_position.vi"("Position"=cluster{"x":dbl, "y":dbl, "z":dbl} {"x"=0.0, "y"=0.0, "z"=0.0}) -> ("Spot"=w957:T3)  [unwired: 1 in, 2 out]
                  }
                  frame True {
                    n64 = Random Number (0-1)() -> (number: 0 to 1=w965:dbl)
                    n65 = Random Number (0-1)() -> (number: 0 to 1=w966:dbl)
                    n66 = Bundle("number: 0 to 1"=w966, "number: 0 to 1"=w965) -> (w964:T20)  [unwired: 1 out]
                    n67 = Multiply(x=w964, y=w959) -> (x*y=w961:cluster{dbl, dbl})
                    n68 = Add(x=w961, y=w958) -> (x+y=w960:cluster{dbl, dbl})
                    n69 = call "coords_image_to_real_currentimage.vi"("Position (pixels on image)"=w960) -> ("Position (real coords)"=w962:cluster{dbl, dbl, "Z":dbl})  [unwired: 9 in]
                    n70 = call "replace_position.vi"("Position"=w962) -> ("Spot"=w963:T3)  [unwired: 1 in, 2 out]
                  }
                }
                n71 = Build Array (concatenate)(w952, w948) -> (w953:T3[])
                n72 = Build Array (concatenate)(w950, cluster{i32, "Label.Visible":bool} {0, "Label.Visible"=TRUE}) -> (w954:T9[])
              }
              event "Position": Value Change {
                # "If the position has changed, translate the spots"
                n73 = event-data() -> ("OldVal"=w980:cluster{"x":dbl, "y":dbl, "z":dbl}, "NewVal"=w981:cluster{"x":dbl, "y":dbl, "z":dbl})  [unwired: 5 out]
                n74 = flat-sequence {
                  tunnel: w982 -> [w986]
                  tunnel: w979 -> [w985]
                  tunnel: w975 -> [w984]
                  tunnel: [w983] -> w976
                  frame #0 {
                    n75 = for {
                      tunnel: w984 -> [w991] mode=indexing
                      tunnel: w986 -> [w988] mode=indexing
                      tunnel: [w990] -> w983 mode=indexing
                      tunnel: w985 -> [w989]
                      n76 = Unbundle(w988) -> ("Selected"=w987:bool)  [unwired: 1 out]
                      n77 = case shown="True" w987 {
                        tunnel: w991 -> [w992 w997]
                        tunnel: [w992 w996] -> w990
                        tunnel: w989 -> [_ w993]
                        frame False {
                        }
                        frame True {
                          n78 = call "extract_position.vi"("Spot"=w997) -> ("Position"=w994:cluster{"x":dbl, "y":dbl, "z":dbl})
                          n79 = Add(x=w994, y=w993) -> (x+y=w995:cluster{"x":dbl, "y":dbl, "z":dbl})
                          n80 = call "replace_position.vi"("Position"=w995, "Spot in"=w997) -> ("Spot"=w996:T3)  [unwired: 2 out]
                        }
                      }
                    }
                  }
                }
                n81 = Subtract(x=w981, y=w980) -> (x-y=w979:cluster{"x":dbl, "y":dbl, "z":dbl})
                n82 = local read "# of Spots"() -> (w978:dbl)
                n83 = stacked-sequence {
                  tunnel: w975 -> [_ w1002 _]
                  tunnel: w976 -> [_ w1001 _]
                  tunnel: w978 -> [_ w1000 _]
                  tunnel: [_ _ w1049] -> w977
                  tunnel: w976 -> [_ _ w1048]
                  tunnel: w975 -> [_ _ w1047]
                  tunnel: [_ _ w1046] -> w974
                  frame #0 {
                    n84 = local write "Looper"(FALSE) -> ()
                    "init" <- 0
                  }
                  frame #1 {
                    n85 = for {
                      N: w1000 -> [_]
                      tunnel: w1002 -> [w1007]
                      tunnel: w1001 -> [w1012]
                      stop <- w1013 stop-if-true
                      n86 = local read "init"() -> (w1006:dbl)
                      n87 = Index Array(array=w1012, index=w1006) -> (element=w1011:T3)
                      n88 = Index Array(array=w1007, index=w1006) -> (element=w1005:T3)
                      n89 = Unbundle By Name(w1011) -> ("Position.x"=w1010:dbl, "Position.y"=w1009:dbl)
                      n90 = local read "# of Spots"() -> (w1008:dbl)
                      n91 = Unbundle By Name(w1005) -> ("Position.x"=→"Old X":dbl, "Position.y"=→"Old Y":dbl)
                      n92 = local write "New X"(w1010) -> ()
                      n93 = local write "New Y"(w1009) -> ()
                      n94 = stacked-sequence {
                        tunnel: w1007 -> [w1018 _]
                        tunnel: w1010 -> [w1017 _]
                        tunnel: w1009 -> [w1016 _]
                        tunnel: w1008 -> [w1015 _]
                        tunnel: w1006 -> [w1014 _]
                        frame #0 {
                          n95 = for {
                            N: w1015 -> [_]
                            tunnel: w1018 -> [w1040]
                            tunnel: w1017 -> [w1039]
                            tunnel: w1016 -> [w1037]
                            tunnel: w1014 -> [w1022]
                            i -> [w1024]
                            stop <- w1023 stop-if-true
                            n96 = Index Array(array=w1040, index=w1024) -> (element=w1041:T3)
                            n97 = Unbundle By Name(w1041) -> ("Position.x"=w1038:dbl, "Position.y"=w1036:dbl)
                            n98 = Subtract(x=w1039, y=w1038) -> (x-y=w1035:dbl)
                            n99 = Subtract(x=w1037, y=w1036) -> (x-y=w1034:dbl)
                            n100 = Square(x=w1035) -> (x^2=w1033:dbl)
                            n101 = Square(x=w1034) -> (x^2=w1032:dbl)
                            n102 = local read "# of Spots"() -> (w1026:dbl)
                            n103 = Add(x=w1033, y=w1032) -> (x+y=w1031:dbl)
                            n104 = local read "Buffer Zone"() -> (w1021:dbl)
                            n105 = Square Root(x=w1031) -> (sqrt(x)=w1030:dbl)
                            n106 = Multiply(x=2, y=w1021) -> (x*y=w1019:dbl)
                            n107 = Less?(x=w1030, y=w1019) -> (x < y?=w1028:bool)
                            n108 = Not Equal?(x=w1022, y=w1024) -> (x != y?=w1027:bool)
                            n109 = Equal?(x=w1026, y=w1024) -> (x = y?=w1029:bool)
                            n110 = And(x=w1027, y=w1028) -> (x .and. y?=w1025:bool)
                            "Looper" <- w1025
                            n111 = Or(x=w1025, y=w1029) -> (x .or. y?=w1023:bool)
                          }
                        }
                        frame #1 {
                          n112 = local read "Looper"() -> (w1042:bool)
                          n113 = case shown="False" w1042 {
                            frame False {
                              n114 = local read "init"() -> (w1043:dbl)
                              n115 = Add(x=w1043, y=1) -> (x+y=w1045:dbl)
                              n116 = local write "init"(w1045) -> ()
                            }
                            frame True {
                            }
                          }
                        }
                      }
                      n117 = local read "Looper"() -> (w1013:bool)
                    }
                  }
                  frame #2 {
                    n118 = local read "Looper"() -> (w1050:bool)
                    n119 = case shown="True" w1050 {
                      tunnel: w1048 -> [w1054 _]
                      tunnel: w1047 -> [_ w1062]
                      tunnel: ["This is an acceptable entry." "ERROR: A bubble will intersect the buffer zone."] -> w1049
                      tunnel: [w1054 w1062] -> w1046
                      frame False {
                        n120 = local write "Looper"(FALSE) -> ()
                        n121 = local read "Current Spot #"() -> (w1055:dbl)
                        n122 = Index Array(array=w1054, index=w1055) -> (element=w1053:T3)
                        n123 = Unbundle By Name(w1053) -> ("Position.x"=w1052:dbl, "Position.y"=w1051:dbl)
                        n124 = local write "New Y"(w1051) -> ()
                        n125 = local write "New X"(w1052) -> ()
                      }
                      frame True {
                        # "Restore original position"
                        n126 = local write "Looper"(FALSE) -> ()
                        n127 = local read "Old Y"() -> (w1059:dbl)
                        n128 = local read "Old X"() -> (w1060:dbl)
                        n129 = local read "Position"() -> (w1058:cluster{"x":dbl, "y":dbl, "z":dbl})
                        n130 = Bundle By Name(cluster=w1058, "x"=w1060, "y"=w1059) -> (w1061:cluster{"x":dbl, "y":dbl, "z":dbl})
                        n131 = local write "Position"(w1061) -> ()
                      }
                    }
                  }
                }
                "Position Indicator" <- w977
              }
              event "Size": Value Change {
                # "If we were constraining the aspect ratio, or preventing a divide by zero, the size control on the FP may be incorrect.  We refresh it in here to stop it displaying a wrong value."
                # "If the size has changed, scale the spots"
                n132 = event-data() -> ("OldVal"=w1071:cluster{"x":dbl, "y":dbl, "z":dbl}, "NewVal"=w1077:cluster{"x":dbl, "y":dbl, "z":dbl})  [unwired: 5 out]
                n133 = Not Equal?(x=w1071, y=w1077) -> (x != y?=w1070:cluster{"x":bool, "y":bool, "z":bool})
                n134 = Divide(x=w1077, y=w1071) -> (x/y=w1076:cluster{"x":dbl, "y":dbl, "z":dbl})
                n135 = Not Equal To 0?(x=w1071) -> (x != 0?=w1069:cluster{"x":bool, "y":bool, "z":bool})
                n136 = And(x=w1070, y=w1069) -> (x .and. y?=w1068:cluster{"x":bool, "y":bool, "z":bool})
                n137 = Cluster To Array(cluster=w1068) -> (array=w1075:bool[])
                n138 = Cluster To Array(cluster=w1076) -> (array=w1074:dbl[])
                n139 = case shown="True" "lock aspect ratio" {
                  tunnel: w1075 -> [w1083 w1100]
                  tunnel: w1074 -> [w1082 w1098]
                  tunnel: [w1080 w1090] -> w1073
                  frame False {
                    # "We are not constraining the aspect ratio here, so just check we're not introducing NAs"
                    n140 = for {
                      tunnel: w1083 -> [w1089] mode=indexing
                      tunnel: w1082 -> [w1085] mode=indexing
                      tunnel: [w1087] -> w1081 mode=indexing
                      n141 = Not A Number/Path/Refnum?(number/path/refnum=w1085) -> (NaN/Path/Refnum?=w1086:bool)
                      n142 = Compound Arithmetic op=AND(w1089, invert w1086) -> (w1088:bool)
                      n143 = Select(t=w1085, s=w1088, f=1.0) -> (s? t:f=w1087:dbl)
                    }
                    n144 = Array To Cluster(array=w1081) -> (cluster=w1080:cluster{"[0]":dbl, "[1]":dbl, "[2]":dbl})
                  }
                  frame True {
                    # "Pick the first element that changed and use it.  Also need to make sure (1) an element did change and (2) everything's valid (no divide by zeros)"
                    n145 = Search 1D Array(1D array=w1100, element=TRUE) -> (index of element=w1097:i32)  [unwired: 1 in]
                    n146 = Index Array(array=w1098, index=w1097) -> (element=w1093:dbl)
                    n147 = Not A Number/Path/Refnum?(number/path/refnum=w1093) -> (NaN/Path/Refnum?=w1096:bool)
                    n148 = Less Than 0?(x=w1097) -> (x < 0?=w1095:bool)
                    n149 = Or(x=w1096, y=w1095) -> (x .or. y?=w1094:bool)
                    n150 = Select(t=1.0, s=w1094, f=w1093) -> (s? t:f=w1091:dbl)
                    n151 = Bundle("x"=w1091, "x"=w1091, "x"=w1091) -> (w1090:cluster{"x":dbl, "x":dbl, "x":dbl})  [unwired: 1 in]
                  }
                }
                n152 = for {
                  tunnel: w1079 -> [w1106] mode=indexing
                  tunnel: w1066 -> [w1103] mode=indexing
                  tunnel: [w1105] -> w1067 mode=indexing
                  tunnel: w1073 -> [w1104]
                  tunnel: w1078 -> [w1101]
                  n153 = Unbundle(w1103) -> ("Selected"=w1102:bool)  [unwired: 1 out]
                  n154 = case shown="True" w1102 {
                    tunnel: w1106 -> [w1107 w1115]
                    tunnel: [w1107 w1114] -> w1105
                    tunnel: w1104 -> [_ w1113]
                    tunnel: w1101 -> [_ w1109]
                    frame False {
                    }
                    frame True {
                      n155 = call "extract_position.vi"("Spot"=w1115) -> ("Position"=w1111:cluster{"x":dbl, "y":dbl, "z":dbl})
                      n156 = Subtract(x=w1111, y=w1109) -> (x-y=w1112:cluster{"x":dbl, "y":dbl, "z":dbl})
                      n157 = Multiply(x=w1112, y=w1113) -> (x*y=w1110:cluster{"x":dbl, dbl, dbl})
                      n158 = Add(x=w1109, y=w1110) -> (x+y=w1108:cluster{"x":dbl, dbl, dbl})
                      n159 = call "replace_position.vi"("Position"=w1108, "Spot in"=w1115) -> ("Spot"=w1114:T3)  [unwired: 2 out]
                    }
                  }
                }
                n160 = call "find_centroid.vi"("Selection and Groups"=w1066, "Spots"=w1067) -> ("size"=w1065:cluster{"x":dbl, "y":dbl, "z":dbl})  [unwired: 2 in, 4 out]
                n161 = local write "Size"(w1065) -> ()
              }
              event "Intensity": Value Change {
                # "When  the user changes intensity, scale all the spots selected so the new mean is correct but keep the ratio between the selected spots.\n\nThe exception to this is when the mean intensity is zero, in which case multiplying makes no sense- in that case we just replace with the new value."
                n162 = event-data() -> ("NewVal"=w1116:dbl, "OldVal"=w1123:dbl)  [unwired: 5 out]
                n163 = Equal To 0?(x=w1123) -> (x = 0?=w1119:bool)
                n164 = Not A Number/Path/Refnum?(number/path/refnum=w1123) -> (NaN/Path/Refnum?=w1118:bool)
                n165 = Or(x=w1119, y=w1118) -> (x .or. y?=w1117:bool)
                n166 = Divide(x=w1116, y=w1123) -> (x/y=w1120:dbl)
                n167 = for {
                  tunnel: w1124 -> [w1129] mode=indexing
                  tunnel: w1121 -> [w1131] mode=indexing
                  tunnel: [w1128] -> w1122 mode=indexing
                  tunnel: w1120 -> [w1127]
                  tunnel: w1117 -> [w1126]
                  tunnel: w1116 -> [w1125]
                  n168 = Unbundle(w1131) -> ("Selected"=w1130:bool)  [unwired: 1 out]
                  n169 = case shown="True" w1130 {
                    tunnel: w1129 -> [w1132 w1139]
                    tunnel: [w1132 w1136] -> w1128
                    tunnel: w1127 -> [_ w1135]
                    tunnel: w1126 -> [_ w1134]
                    tunnel: w1125 -> [_ w1133]
                    frame False {
                    }
                    frame True {
                      n170 = Unbundle By Name(w1139) -> ("Intensity"=w1137:dbl)
                      n171 = case shown="True" w1134 {
                        tunnel: [w1142 w1143] -> w1138
                        tunnel: w1137 -> [w1141 _]
                        tunnel: w1135 -> [w1140 _]
                        tunnel: w1133 -> [_ w1143]
                        frame False {
                          n172 = Multiply(x=w1141, y=w1140) -> (x*y=w1142:dbl)
                        }
                        frame True {
                        }
                      }
                      n173 = Bundle By Name(cluster=w1139, "Intensity"=w1138) -> (w1136:T3)
                    }
                  }
                }
              }
              event "phase": Value Change {
                # "When  the user changes phase, translate the phase of all spots selectedd"
                n174 = event-data() -> ("NewVal"=w1145:dbl, "OldVal"=w1149:dbl)  [unwired: 5 out]
                n175 = Not A Number/Path/Refnum?(number/path/refnum=w1149) -> (NaN/Path/Refnum?=w1144:bool)
                n176 = Subtract(x=w1145, y=w1149) -> (x-y=w1146:dbl)
                n177 = for {
                  tunnel: w1150 -> [w1155] mode=indexing
                  tunnel: w1147 -> [w1157] mode=indexing
                  tunnel: [w1154] -> w1148 mode=indexing
                  tunnel: w1146 -> [w1153]
                  tunnel: w1144 -> [w1152]
                  tunnel: w1145 -> [w1151]
                  n178 = Unbundle(w1157) -> ("Selected"=w1156:bool)  [unwired: 1 out]
                  n179 = case shown="False" w1156 {
                    tunnel: w1155 -> [w1158 w1165]
                    tunnel: [w1158 w1162] -> w1154
                    tunnel: w1153 -> [_ w1161]
                    tunnel: w1152 -> [_ w1160]
                    tunnel: w1151 -> [_ w1159]
                    frame False {
                    }
                    frame True {
                      n180 = Unbundle By Name(w1165) -> ("Phase"=w1163:dbl)
                      n181 = case shown="False" w1160 {
                        tunnel: [w1168 w1169] -> w1164
                        tunnel: w1163 -> [w1167 _]
                        tunnel: w1161 -> [w1166 _]
                        tunnel: w1159 -> [_ w1169]
                        frame False {
                          n182 = Add(x=w1167, y=w1166) -> (x+y=w1168:dbl)
                        }
                        frame True {
                        }
                      }
                      n183 = Bundle By Name(cluster=w1165, "Phase"=w1164) -> (w1162:T3)
                    }
                  }
                }
              }
              event "Vortex Charge": Value Change {
                # "When  the user changes l, just set all selected spots to have that value of l."
                n184 = event-data() -> ("NewVal"=w1170:i8)  [unwired: 6 out]
                n185 = for {
                  tunnel: w1173 -> [w1176] mode=indexing
                  tunnel: w1171 -> [w1178] mode=indexing
                  tunnel: [w1175] -> w1172 mode=indexing
                  tunnel: w1170 -> [w1174]
                  n186 = Unbundle(w1178) -> ("Selected"=w1177:bool)  [unwired: 1 out]
                  n187 = case shown="True" w1177 {
                    tunnel: w1176 -> [w1179 w1182]
                    tunnel: [w1179 w1181] -> w1175
                    tunnel: w1174 -> [_ w1180]
                    frame False {
                    }
                    frame True {
                      n188 = Bundle By Name(cluster=w1182, "Vortex Charge"=w1180) -> (w1181:T3)
                    }
                  }
                }
              }
            }
          }
          frame "Spot Shape" {
            # "We update the spot shape tab only when spots have changed OUTSIDE this tab.  This avoids unnecessary jumping about of the tab control."
            n189 = call "find_centroid.vi"("Selection and Groups"=w1193, "Spots"=w1194) -> ("Mean Values"=w1189:T3)  [unwired: 2 in, 4 out]
            n190 = Wait (ms)(milliseconds to wait=u32 10) -> ()  [unwired: 1 out]
            n191 = call "spots_shape.vi"("Selection and Groups"=w1193, "Spots"=w1194) -> ("Spot Shape"=w1196:enum32{"Normal", "Line", "NA", "Mixed"})  [unwired: 7 in]
            n192 = feedback-in #4(w1189) -> ()
            n193 = feedback #4() -> (w1190:T3)  [unwired: 1 in]
            n194 = Not Equal?(x=w1190, y=w1189) -> (x != y?=w1195:bool)
            n195 = feedback #5() -> (w1185:enum32{"Normal", "Line", "NA", "Mixed"})  [unwired: 1 in]
            n196 = feedback #6() -> (w1187:T3)  [unwired: 1 in]
            n197 = Not Equal?(x=w1187, y=w1189) -> (x != y?=w1186:bool)
            n198 = case shown="False" w1186 {
              tunnel: w1196 -> [_ w1315]
              tunnel: ["Spot Shape" w1315] -> w1184
              frame False {
              }
              frame True {
                n199 = local write "Spot Shape"(w1315) -> ()
              }
            }
            n200 = feedback-in #5(w1184) -> ()
            n201 = Not Equal?(x=w1184, y=w1185) -> (x != y?=w1183:bool)
            n202 = case shown="\"Normal\", Default" w1184 {
              tunnel: w1194 -> [w1200 w1217 w1243 w1313]
              tunnel: w1193 -> [w1199 w1216 w1242 w1312]
              tunnel: [w1199 w1215 w1240 w1312] -> w1191
              tunnel: [w1198 w1214 w1241 w1313] -> w1192
              tunnel: w1189 -> [_ w1213 w1239 _]
              tunnel: w1195 -> [_ w1212 w1238 _]
              tunnel: w1183 -> [_ w1210 w1236 _]
              frame "Normal", Default {
                # "If \"normal\" is selected, don't allow any NA or line-trapping stuff"
                n203 = for {
                  tunnel: w1200 -> [w1203] mode=indexing
                  tunnel: w1199 -> [w1202] mode=indexing
                  tunnel: [w1204] -> w1198 mode=indexing
                  n204 = Unbundle(w1202) -> ("Selected"=w1201:bool)  [unwired: 1 out]
                  n205 = case shown="True" w1201 {
                    tunnel: [w1205 w1209] -> w1204
                    tunnel: w1203 -> [w1205 w1208]
                    frame False {
                    }
                    frame True {
                      n206 = Bundle By Name(cluster=w1208, "NA Position"=cluster{"x":dbl, "y":dbl, "r":dbl} {"x"=0.0, "y"=0.0, "r"=1.0} ("x"), "Line Trapping"=T4 {"Vector"={"x"=0.0, "y"=0.0, "z"=0.0}, "Phase Gradient"=0.0}) -> (w1209:T3)
                    }
                  }
                }
              }
              frame "Line" {
                # "If it's out of date, update front panel"
                n207 = Or(x=w1212, y=w1210) -> (x .or. y?=w1211:bool)
                n208 = case shown="True" w1211 {
                  tunnel: w1213 -> [_ w1220]
                  frame False {
                  }
                  frame True {
                    n209 = Unbundle By Name(w1220) -> ("Line Trapping"=w1219:T4)
                    n210 = local write "Line Trapping"(w1219) -> ()
                  }
                }
                n211 = event shown="[1] \"Line Trapping\": Value Change" {
                  selector: _ -> [_ _]
                  dyn-events: _ -> [_ _]
                  timeout: 10 -> [_ _]
                  tunnel: w1217 -> [w1222 w1226]
                  tunnel: w1216 -> [w1221 w1224]
                  tunnel: [w1222 w1225] -> w1214
                  tunnel: [w1221 w1224] -> w1215
                  event Timeout {
                    n212 = event-data() -> ()  [unwired: 3 out]
                  }
                  event Value Change {
                    # "If the line vector has changed, update it"
                    n213 = event-data() -> ("NewVal"=w1223:T4)  [unwired: 6 out]
                    n214 = for {
                      tunnel: w1226 -> [w1231] mode=indexing
                      tunnel: w1224 -> [w1228] mode=indexing
                      tunnel: [w1230] -> w1225 mode=indexing
                      tunnel: w1223 -> [w1229]
                      n215 = Unbundle(w1228) -> ("Selected"=w1227:bool)  [unwired: 1 out]
                      n216 = case shown="True" w1227 {
                        tunnel: w1231 -> [w1232 w1234]
                        tunnel: [w1232 w1235] -> w1230
                        tunnel: w1229 -> [_ w1233]
                        frame False {
                        }
                        frame True {
                          n217 = Bundle By Name(cluster=w1234, "Line Trapping"=w1233) -> (w1235:T3)
                        }
                      }
                    }
                  }
                }
              }
              frame "NA" {
                n218 = Or(x=w1236, y=w1238) -> (x .or. y?=w1237:bool)
                n219 = case shown="True" w1237 {
                  tunnel: w1239 -> [_ w1248]
                  frame False {
                  }
                  frame True {
                    n220 = Unbundle By Name(w1248) -> ("NA Position"=w1247:cluster{"x":dbl, "y":dbl, "r":dbl})
                    n221 = call "xyz_to_xy.vi"("Position"=w1247) -> ("Position (2D)"=w1246:cluster{"x":dbl, "y":dbl}, "z"=w1245:dbl)  [unwired: 6 out]
                    n222 = local write "Position on back aperture"(w1246) -> ()
                    n223 = local write "Radius on back aperture"(w1245) -> ()
                  }
                }
                n224 = event shown="[3] \"Scale BA\": Value Change" {
                  selector: _ -> [_ _ _ _]
                  dyn-events: _ -> [_ _ _ _]
                  timeout: 10 -> [_ _ _ _]
                  tunnel: w1243 -> [w1250 w1256 w1277 w1299]
                  tunnel: w1242 -> [w1249 w1254 w1274 w1300]
                  tunnel: [w1250 w1255 w1275 w1297] -> w1241
                  tunnel: [w1249 w1254 w1274 w1300] -> w1240
                  event Timeout {
                    n225 = event-data() -> ()  [unwired: 3 out]
                  }
                  event "Position on back aperture": Value Change {
                    # "If the position has changed, translate the spots"
                    n226 = event-data() -> ("OldVal"=w1252:cluster{"x":dbl, "y":dbl}, "NewVal"=w1253:cluster{"x":dbl, "y":dbl})  [unwired: 5 out]
                    n227 = Subtract(x=w1253, y=w1252) -> (x-y=w1251:cluster{"x":dbl, "y":dbl})
                    n228 = for {
                      tunnel: w1256 -> [w1261] mode=indexing
                      tunnel: w1254 -> [w1258] mode=indexing
                      tunnel: [w1260] -> w1255 mode=indexing
                      tunnel: w1251 -> [w1259]
                      n229 = Unbundle(w1258) -> ("Selected"=w1257:bool)  [unwired: 1 out]
                      n230 = case shown="True" w1257 {
                        tunnel: w1261 -> [w1262 w1264]
                        tunnel: [w1262 w1265] -> w1260
                        tunnel: w1259 -> [_ w1266]
                        frame False {
                        }
                        frame True {
                          n231 = Unbundle By Name(w1264) -> ("NA Position"=w1268:cluster{"x":dbl, "y":dbl, "r":dbl})
                          n232 = call "xy_to_xyz.vi"("Position (2D)"=w1266) -> ("Position (3D)"=w1267:cluster{dbl, dbl, dbl})  [unwired: 1 in, 2 out]
                          n233 = Add(x=w1268, y=w1267) -> (x+y=w1263:cluster{dbl, dbl, dbl})
                          n234 = Bundle By Name(cluster=w1264, "NA Position"=w1263) -> (w1265:T3)
                        }
                      }
                    }
                  }
                  event "Radius on back aperture": Value Change {
                    # "When  the user changes intensity, scale all the spots selected so the new mean is correct but keep the ratio between the selected spots.\n\nThe exception to this is when the mean intensity is zero, in which case multiplying makes no sense- in that case we just replace with the new value."
                    n235 = event-data() -> ("NewVal"=w1269:dbl, "OldVal"=w1276:dbl)  [unwired: 5 out]
                    n236 = Equal To 0?(x=w1276) -> (x = 0?=w1272:bool)
                    n237 = Not A Number/Path/Refnum?(number/path/refnum=w1276) -> (NaN/Path/Refnum?=w1271:bool)
                    n238 = Or(x=w1272, y=w1271) -> (x .or. y?=w1270:bool)
                    n239 = Divide(x=w1269, y=w1276) -> (x/y=w1273:dbl)
                    n240 = for {
                      tunnel: w1277 -> [w1282] mode=indexing
                      tunnel: w1274 -> [w1284] mode=indexing
                      tunnel: [w1281] -> w1275 mode=indexing
                      tunnel: w1273 -> [w1280]
                      tunnel: w1270 -> [w1279]
                      tunnel: w1269 -> [w1278]
                      n241 = Unbundle(w1284) -> ("Selected"=w1283:bool)  [unwired: 1 out]
                      n242 = case shown="True" w1283 {
                        tunnel: w1282 -> [w1285 w1292]
                        tunnel: [w1285 w1289] -> w1281
                        tunnel: w1280 -> [_ w1288]
                        tunnel: w1279 -> [_ w1287]
                        tunnel: w1278 -> [_ w1286]
                        frame False {
                        }
                        frame True {
                          n243 = Unbundle By Name(w1292) -> ("NA Position.r"=w1290:dbl)
                          n244 = case shown="False" w1287 {
                            tunnel: [w1295 w1296] -> w1291
                            tunnel: w1290 -> [w1294 _]
                            tunnel: w1288 -> [w1293 _]
                            tunnel: w1286 -> [_ w1296]
                            frame False {
                              n245 = Multiply(x=w1294, y=w1293) -> (x*y=w1295:dbl)
                            }
                            frame True {
                            }
                          }
                          n246 = Bundle By Name(cluster=w1292, "NA Position.r"=w1291) -> (w1289:T3)
                        }
                      }
                    }
                  }
                  event "Scale BA": Value Change {
                    n247 = event-data() -> ()  [unwired: 7 out]
                    n248 = for {
                      tunnel: w1300 -> [w1305] mode=indexing
                      tunnel: w1299 -> [w1303] mode=indexing
                      tunnel: "Scale back aperture" -> [w1302]
                      tunnel: [w1301] -> w1297 mode=indexing
                      n249 = Unbundle(w1305) -> ("Selected"=w1304:bool)  [unwired: 1 out]
                      n250 = case shown="True" w1304 {
                        tunnel: w1303 -> [w1306 w1307]
                        tunnel: w1302 -> [_ w1310]
                        tunnel: [w1306 w1308] -> w1301
                        frame False {
                        }
                        frame True {
                          n251 = Unbundle By Name(w1307) -> ("NA Position"=w1311:cluster{"x":dbl, "y":dbl, "r":dbl})
                          n252 = Multiply(x=w1310, y=w1311) -> (x*y=w1309:cluster{"x":dbl, "y":dbl, "r":dbl})
                          n253 = Bundle By Name(cluster=w1307, "NA Position"=w1309) -> (w1308:T3)
                        }
                      }
                    }
                  }
                }
              }
              frame "Mixed" {
              }
            }
            n254 = call "find_centroid.vi"("Selection and Groups"=w1191, "Spots"=w1192) -> ("Mean Values"=w1188:T3)  [unwired: 2 in, 4 out]
            n255 = feedback-in #6(w1188) -> ()
          }
          frame "Rotate" {
            w1326 = u32 0 items=["Frame", "Fill", "Highlight"] ("Drawing Mode")
            w1325 = u32 0 ("Color")
            w1322 = i16 100 ("radius")
            # "It's necessary to check this has changed to stop us unintentionally \"spinning\" the spots..."
            # "Draw the centroid as a spot, then a large circle+cross"
            # "It's important that this loop doesn't go too fast- it hogs the CPU.  However, each tab can have a different loop speed."
            n256 = Unbundle By Name(w1319) -> ("Position (Image Pixels)"=w1335:cluster{"X":dbl, "Y":dbl}, "Previous Position (Image Pixels)"=w1334:cluster{"X":dbl, "Y":dbl}, "Dragging"=w1336:bool)
            n257 = feedback-in #7(w1319) -> ()
            n258 = feedback #7() -> (w1320:T13)  [unwired: 1 in]
            n259 = call "find_centroid.vi"("Selection and Groups"=w1337, "Spots"=w1340) -> ("centroid"=w1333:cluster{"x":dbl, "y":dbl, "z":dbl})  [unwired: 2 in, 4 out]
            n260 = Not Equal?(x=w1319, y=w1320) -> (x != y?=w1317:bool)
            n261 = Wait (ms)(milliseconds to wait=u32 10) -> ()  [unwired: 1 out]
            n262 = And(x=w1317, y=w1336) -> (x .and. y?=w1318:bool)
            n263 = call "coords_real_to_image_currentview.vi"("Position (real coords)"=w1333) -> ("Position (pixels, relative to the top left of the image)"=w1316:cluster{dbl, dbl})  [unwired: 7 in, 1 out]
            n264 = case shown="True" w1318 {
              tunnel: w1340 -> [w1349 w1393]
              tunnel: [w1351 w1392] -> w1339
              tunnel: w1337 -> [w1350 w1394]
              tunnel: [w1350 w1394] -> w1338
              tunnel: w1333 -> [w1348 w1385]
              tunnel: w1335 -> [_ w1384]
              tunnel: w1334 -> [_ w1383]
              tunnel: w1316 -> [_ w1382]
              frame False {
                n265 = event shown="[1] Timeout" {
                  selector: _ -> [_ _]
                  dyn-events: _ -> [_ _]
                  timeout: 10 -> [_ _]
                  tunnel: [w1364 w1381] -> w1351
                  tunnel: w1350 -> [w1363 _]
                  tunnel: w1349 -> [w1362 w1381]
                  tunnel: w1348 -> [w1358 _]
                  event "rotate": Value Change {
                    n266 = event-data() -> ()  [unwired: 6 out]
                    n267 = case shown="3" "Rotation Axis" {
                      tunnel: [cluster{dbl, dbl, dbl} {0.0, 0.0, 1.0} ("Custom Axis") cluster{dbl, dbl, dbl} {1.0, 0.0, 0.0} ("Custom Axis") cluster{dbl, dbl, dbl} {0.0, 1.0, 0.0} ("Custom Axis") "Custom Axis"] -> w1359
                      frame 0, Default {
                        # "Z"
                      }
                      frame 1 {
                        # "X"
                      }
                      frame 2 {
                        # "Y"
                      }
                      frame 3 {
                      }
                    }
                    n268 = call "normalise_3d_vector.vi"("Vector"=w1359) -> ("Unit Vector"=w1361:cluster{dbl, dbl, dbl})  [unwired: 3 out]
                    n269 = Divide(x=6.283185307179586, y=360.0) -> (x/y=w1356:dbl)
                    n270 = Multiply(x="Angle (degrees)", y=w1356) -> (x*y=w1353:dbl)
                    n271 = call "arb_rotation_matrix.vi"("Unit Vector"=w1361, "theta"=w1353) -> ("Real Matrix"=w1365:T10)
                    n272 = for {
                      tunnel: w1363 -> [w1375] mode=indexing
                      tunnel: w1362 -> [w1370] mode=indexing
                      tunnel: [w1371] -> w1364 mode=indexing
                      tunnel: w1358 -> [w1373]
                      tunnel: w1365 -> [w1372]
                      n273 = Unbundle(w1375) -> ("Selected"=w1374:bool)  [unwired: 1 out]
                      n274 = case shown="True" w1374 {
                        tunnel: w1373 -> [_ w1380]
                        tunnel: [w1376 w1379] -> w1371
                        tunnel: w1370 -> [w1376 w1378]
                        tunnel: w1372 -> [_ w1377]
                        frame False {
                        }
                        frame True {
                          n275 = call "apply_matrix_transformation_to_spots.vi"("Transform centre (i.e. transform about this point)"=w1380, "Transformation Matrix (3x3)"=w1377, "Spot In"=w1378) -> ("Spot Out"=w1379:T3)  [unwired: 5 out]
                        }
                      }
                    }
                  }
                  event Timeout {
                    n276 = event-data() -> ()  [unwired: 4 out]
                  }
                }
              }
              frame True {
                # "if the mouse has not moved, stuff will be NaN, so let's make like a leopard and not change our spots"
                # "the magnitude of the change in our direction vector gives the rotation angle in radians"
                # "If it's within 100px of the centroid, pretend the mouse is on the surface of a sphere, and synthesize Z accordingly (z^2=100^2-x^2-y^2).  This allows rotation in 3d :)  The output should always be a unit vector."
                n277 = Build Array(w1384, w1383) -> (w1399:cluster{"X":dbl, "Y":dbl}[])
                n278 = for {
                  tunnel: w1382 -> [w1432]
                  tunnel: w1399 -> [w1428] mode=indexing
                  tunnel: [w1418] -> w1398 mode=indexing
                  n279 = Subtract(x=w1428, y=w1432) -> (x-y=w1423:cluster{dbl, dbl})
                  n280 = Divide(x=w1423, y=100.0 ("x")) -> (x/y=w1424:cluster{dbl, dbl})
                  n281 = Square(x=w1424) -> (x^2=w1431:cluster{dbl, dbl})
                  n282 = Unbundle(w1431) -> (w1429:dbl, w1430:dbl)
                  n283 = Add(x=w1429, y=w1430) -> (x+y=w1420:dbl)
                  n284 = Subtract(x=1.0, y=w1420) -> (x-y=w1426:dbl)
                  n285 = Square Root(x=w1420) -> (sqrt(x)=w1421:dbl)
                  n286 = Greater Than 0?(x=w1426) -> (x > 0?=w1427:bool)
                  n287 = case shown="False" w1427 {
                    tunnel: w1426 -> [_ w1439]
                    tunnel: [0.0 w1438] -> w1417
                    tunnel: w1424 -> [w1436 w1437]
                    tunnel: w1421 -> [w1435 _]
                    tunnel: [w1434 w1437] -> w1419
                    frame False {
                      n288 = Divide(x=w1436, y=w1435) -> (x/y=w1434:cluster{dbl, dbl})
                    }
                    frame True {
                      n289 = Square Root(x=w1439) -> (sqrt(x)=w1438:dbl)
                    }
                  }
                  n290 = call "xy_to_xyz.vi"("z"=w1417, "Position (2D)"=w1419) -> ("Position (3D)"=w1418:cluster{dbl, dbl, dbl})  [unwired: 2 out]
                }
                n291 = Index Array(array=w1398) -> (element #1=w1397:cluster{dbl, dbl, dbl}, element #2=w1388:cluster{dbl, dbl, dbl})  [unwired: 2 in]
                n292 = Add(x=w1397, y=w1388) -> (x+y=w1387:cluster{dbl, dbl, dbl})
                n293 = Subtract(x=w1397, y=w1388) -> (x-y=w1386:cluster{dbl, dbl, dbl})
                n294 = call "cross_product.vi"("b"=w1387, "a"=w1386) -> ("a cross b"=w1396:cluster{dbl, dbl, dbl})
                n295 = call "normalise_3d_vector.vi"("Vector"=w1396) -> ("Unit Vector"=w1395:cluster{dbl, dbl, dbl})  [unwired: 3 out]
                n296 = call "normalise_3d_vector.vi"("Vector"=w1386) -> ("magnitude"=w1390:dbl)  [unwired: 3 out]
                n297 = Not Equal To 0?(x=w1390) -> (x != 0?=w1389:bool)
                n298 = call "arb_rotation_matrix.vi"("Unit Vector"=w1395, "theta"=w1390) -> ("Real Matrix"=w1391:T10)
                n299 = case shown="True" w1389 {
                  tunnel: w1394 -> [_ w1405]
                  tunnel: w1393 -> [w1400 w1404]
                  tunnel: [w1400 w1403] -> w1392
                  tunnel: w1391 -> [_ w1402]
                  tunnel: w1385 -> [_ w1401]
                  frame False {
                  }
                  frame True {
                    n300 = for {
                      tunnel: w1405 -> [w1411] mode=indexing
                      tunnel: w1404 -> [w1408] mode=indexing
                      tunnel: [w1407] -> w1403 mode=indexing
                      tunnel: w1402 -> [w1409]
                      tunnel: w1401 -> [w1406]
                      n301 = Unbundle(w1411) -> ("Selected"=w1410:bool)  [unwired: 1 out]
                      n302 = case shown="True" w1410 {
                        tunnel: [w1412 w1415] -> w1407
                        tunnel: w1408 -> [w1412 w1416]
                        tunnel: w1409 -> [_ w1413]
                        tunnel: w1406 -> [_ w1414]
                        frame False {
                        }
                        frame True {
                          n303 = call "apply_matrix_transformation_to_spots.vi"("Transform centre (i.e. transform about this point)"=w1414, "Transformation Matrix (3x3)"=w1413, "Spot In"=w1416) -> ("Spot Out"=w1415:T3)  [unwired: 5 out]
                        }
                      }
                    }
                  }
                }
              }
            }
            n304 = call "coords_real_to_image_currentview.vi"("Position (real coords)"=w1333) -> ("Position (pixels, relative to the top left of the image)"=w1328:cluster{dbl, dbl}, "z (real coords)"=w1332:dbl)  [unwired: 7 in]
            n305 = expression code="z*1e7+20"(w1332) -> (w1344:dbl)
            n306 = In Range and Coerce(upper limit=100.0, x=w1344, lower limit=2.0) -> (coerced(x)=w1331:dbl)  [unwired: 1 out]
            n307 = Bundle("upper limit"=w1331, "upper limit"=w1331) -> (w1324:cluster{"upper limit":dbl, "upper limit":dbl})  [unwired: 1 in]
            n308 = call "myoverlay_oval.vi"("Color"=w1325, "Drawing Mode"=w1326, "Size"=w1324, "Centre Position (pixels on image)"=w1328) -> ("Overlay Elements Out"=w1330:T21[])  [unwired: 5 in]
            n309 = Bundle("radius"=w1322, "radius"=w1322) -> (w1323:cluster{"radius":i16, "radius":i16})  [unwired: 1 in]
            n310 = call "myoverlay_oval.vi"("Color"=w1325, "Drawing Mode"=w1326, "Size"=w1323, "Centre Position (pixels on image)"=w1328, "Overlay Elements In"=w1330) -> ("Overlay Elements Out"=w1329:T21[])  [unwired: 4 in]
            n311 = Multiply(x=w1322, y=cluster{dbl, dbl}[] [{0.0, 0.0}, {1.0, 0.0}, {0.0, 0.0}, {0.0, 1.0}, {0.0, 0.0}, {-1.0, 0.0}, {0.0, 0.0}, {0.0, -1.0}, {0.0, 0.0}]) -> (x*y=w1341:cluster{dbl, dbl}[])
            n312 = Add(x=w1328, y=w1341) -> (x+y=w1327:cluster{dbl, dbl}[])
            n313 = call "myoverlay_lines.vi"("Color"=w1325, "Drawing Mode"=w1326, "Line Endpoints"=w1327, "Overlay Elements In"=w1329) -> ("Overlay Elements Out"=w1321:T21[])  [unwired: 5 in]
          }
          frame "Patterns" {
            n314 = event shown="[3] \"Optimise\": Value Change" {
              selector: _ -> [_ _ _ _ _]
              dyn-events: _ -> [_ _ _ _ _]
              timeout: u32 10 ("milliseconds to wait") -> [_ _ _ _ _]
              tunnel: [w1458 w1488 w1492 w1495 w1506] -> w1441
              tunnel: [w1457 w1489 w1491 w1498 w1507] -> w1440
              tunnel: w1443 -> [w1456 w1488 w1492 w1496 w1505]
              tunnel: w1442 -> [w1455 w1489 w1491 w1498 w1507]
              event "Generate": Value Change {
                # "If there were previous spots, centre the pattern on the spots"
                n315 = event-data() -> ()  [unwired: 1 in, 1 out]
                n316 = call "find_centroid.vi"("Selection and Groups"=w1455, "Spots"=w1456) -> ("size"=w1451:cluster{"x":dbl, "y":dbl, "z":dbl}, "centroid"=w1447:cluster{"x":dbl, "y":dbl, "z":dbl}, "# selected"=w1453:i16)  [unwired: 2 in, 2 out]
                n317 = Greater?(x=w1453, y=i16 1) -> (0:w1448:bool)
                n318 = case shown="False" w1448 {
                  tunnel: w1451 -> [_ w1474]
                  tunnel: [cluster{"x":dbl, "y":dbl, "z":dbl} {"x"=2e-05, "y"=2e-05, "z"=2e-05} ("size") w1474] -> w1450
                  frame False {
                  }
                  frame True {
                  }
                }
                n319 = case shown="\"HCP Shack-Hartmann\"" "Pattern" {
                  tunnel: [w1476 w1479 w1485] -> w1449
                  tunnel: w1450 -> [_ w1478 _]
                  frame "Square Shack-Hartmann" {
                    n320 = call "patterns_square_shack_hartmann.vi"("N"="Spots across centre") -> ("Spots"=w1476:T3[])
                  }
                  frame "HCP Shack-Hartmann" {
                    n321 = Unbundle By Name(w1478) -> ("x"=w1477:dbl)
                    n322 = call "pattern_hcp_shack_hartmann.vi"("Width"=w1477, "Reference Array?"="Reference Array?", "Fraction of SLM"="Fraction of SLM", "N"="Spots across centre") -> ("Shack-Hartmann Spots"=w1479:T3[])  [unwired: 7 in]
                  }
                  frame "Rectangular Grid" {
                    n323 = call "patterns_rectangular_grid.vi"("spacing/m"="spacing/m", "N"="N") -> ("Spots"=w1485:T3[])
                  }
                }
                n324 = local write "Generate"(FALSE ("Generate")) -> ()
                n325 = case shown="True" w1448 {
                  tunnel: w1449 -> [w1461 w1465]
                  tunnel: w1447 -> [_ w1467]
                  tunnel: [w1461 w1463] -> w1459
                  frame False {
                  }
                  frame True {
                    n326 = call "find_centroid.vi"("Spots"=w1465) -> ("centroid"=w1466:cluster{"x":dbl, "y":dbl, "z":dbl}, "# selected"=→"# selected":i16)  [unwired: 3 in, 3 out]
                    n327 = Subtract(x=w1467, y=w1466) -> (x-y=w1464:cluster{"x":dbl, "y":dbl, "z":dbl})
                    n328 = for {
                      tunnel: w1465 -> [w1470] mode=indexing
                      tunnel: w1464 -> [w1469]
                      tunnel: [w1468] -> w1463 mode=indexing
                      n329 = call "extract_position.vi"("Spot"=w1470) -> ("Position"=w1471:cluster{"x":dbl, "y":dbl, "z":dbl})
                      n330 = Add(x=w1471, y=w1469) -> (x+y=w1472:cluster{"x":dbl, "y":dbl, "z":dbl})
                      n331 = call "replace_position.vi"("Position"=w1472, "Spot in"=w1470) -> ("Spot"=w1468:T3)  [unwired: 2 out]
                    }
                  }
                }
                "Last Pattern" <- w1459
                n332 = call "ensure_selection_matches_spots.vi"("Select All (default: no)"=TRUE ("Select All (default: true)"), "Spots"=w1459) -> ("Selection and Groups out"=w1457:T9[], "Spots (duplicate)"=w1458:T3[])  [unwired: 4 in]
              }
              event "Spots across centre", "Fraction of SLM", "Reference Array?", "N", "spacing/m", "Spots across centre": Value Change {
                n333 = event-data() -> ()  [unwired: 1 in, 1 out]
                n334 = local read "Last Pattern"() -> (w1487:T3[])
                n335 = Equal?(x=w1488, y=w1487) -> (x = y?=w1486:bool)
                n336 = case shown="True" w1486 {
                  selector: w1486 -> [_ w1490]
                  frame False {
                  }
                  frame True {
                    n337 = property on="Generate" class="Bool (strict)"("Val(Sgnl)"=w1490) -> ()  [unwired: 2 in, 2 out]
                  }
                }
              }
              event Timeout {
                n338 = event-data() -> ()  [unwired: 1 in, 1 out]
              }
              event "Optimise": Value Change {
                n339 = event-data() -> ()  [unwired: 1 in, 1 out]
                n340 = for {
                  N: "Iterations" -> [_]
                  tunnel: 203 ("Optimisation Resolution") -> [w1502]
                  shift-right: [w1503] -> w1495
                  shift-left: w1496 -> [w1504]
                  tunnel: "Fall-off/m" -> [w1499]
                  n341 = call "do_gsw_step.vi"("Optimisation Resolution"=w1502, "Sinc Zero"=w1499, "Spots In"=w1504) -> ("non-uniformity"=→"non-uniformity":dbl, "efficiency"=→"efficiency":dbl, "Spots Out"=w1503:T3[])  [unwired: 6 in]
                }
              }
              event "Reset Phase/Amplitude": Value Change {
                n342 = event-data() -> ()  [unwired: 1 in, 1 out]
                n343 = for {
                  tunnel: [w1510] -> w1506 mode=indexing
                  tunnel: w1505 -> [w1511] mode=indexing
                  n344 = Bundle By Name(cluster=w1511, "Phase"=0.0, "Amplitude Correction"=0.0) -> (w1510:T3)
                }
              }
            }
          }
          frame "Plugins" {
            # "The local variable ensures the references are  correct when they make it through to the \"close plugins\" block."
            # "This is the error from loading/unloading VIs on the front panel"
            n345 = control-ref of="Plugin Pnl"() -> (w1515:refnum<vi>)
            n346 = Wait (ms)(milliseconds to wait=u32 10) -> ()  [unwired: 1 out]
            n347 = feedback #8() -> (w1514:T5)
            n348 = feedback #9() -> (w1516:errorcluster)
            n349 = event shown="[1] \"Plugin:\": Value Change" {
              selector: _ -> [_ _ _]
              dyn-events: _ -> [_ _ _]
              timeout: 10 -> [_ _ _]
              tunnel: "Abort Plugin" -> [w1523 _ _]
              tunnel: "Plugin:" -> [w1528 _ w1544]
              tunnel: w1516 -> [w1527 w1542 w1546]
              tunnel: [w1526 w1537 w1545] -> w1517
              tunnel: [w1525 w1538 w1548] -> w1513
              tunnel: w1514 -> [w1529 w1539 w1547]
              tunnel: w1515 -> [_ w1540 _]
              event Timeout {
                n350 = event-data() -> ()  [unwired: 1 in, 2 out]
                n351 = Not(x=w1523) -> (.not. x?=w1524:bool)
                n352 = case shown="True" w1524 {
                  tunnel: w1529 -> [w1531 w1536]
                  tunnel: w1528 -> [_ w1535]
                  tunnel: w1527 -> [w1530 w1534]
                  tunnel: [w1530 w1533] -> w1526
                  tunnel: [w1531 w1532] -> w1525
                  frame False {
                  }
                  frame True {
                    n353 = call "plugins_run.vi"("Error In"=w1534, "Plugin Index"=w1535, "Plugins In"=w1536) -> ("Error Out"=w1533:errorcluster, "Plugins"=w1532:T5)  [unwired: 7 in]
                  }
                }
              }
              event "Plugin:": Value Change {
                n354 = event-data() -> ("NewVal"=w1541:u16)  [unwired: 1 in]
                n355 = call "plugins_switch.vi"("error in"=w1542, "Plugin Pnl"=w1540, "Plugin Index"=w1541, "Plugins In"=w1539) -> ("error out"=w1537:errorcluster, "Plugins Out"=w1538:T5)  [unwired: 4 in]
              }
              event "Abort Plugin": Value Change {
                n356 = event-data() -> ("NewVal"=w1543:bool)  [unwired: 1 in]
                n357 = case shown="True" w1543 {
                  tunnel: [w1550 w1555] -> w1548
                  tunnel: w1547 -> [w1550 w1554]
                  tunnel: w1546 -> [w1549 w1553]
                  tunnel: [w1549 w1552] -> w1545
                  tunnel: w1544 -> [_ w1551]
                  frame False {
                  }
                  frame True {
                    n358 = call "plugins_abort.vi"("Error In"=w1553, "Plugin Index"=w1551, "Plugins In"=w1554) -> ("Error Out"=w1552:errorcluster, "Plugins Out"=w1555:T5)  [unwired: 7 in]
                  }
                }
              }
            }
            n359 = feedback-in #8(w1513) -> ()
            n360 = feedback-in #9(w1517) -> ()
            n361 = local write "Plugins"(w1513) -> ()
          }
          frame "Video" {
            # "All the controls on this tab are in the bottom (camera) loop."
            n362 = Wait (ms)(milliseconds to wait=u32 10) -> ()  [unwired: 1 out]
            n363 = property on="Property Node" class="ImageControl"(reference=w1556) -> ("Image Information String"=→"Image Information":string)  [unwired: 1 in, 2 out]
          }
          frame "Sequence" {
          }
          frame "Sequence Creator" {
          }
          frame "Spot Control" {
          }
          frame "Load/Save" {
          }
          frame "Image Process" {
          }
        }
      }
      event "Tab": Value Change {
        w1574 = T22 [enum."Video", enum."Particle Tracking"] items=["Current Spot", "Rotate", "Spot Shape", "Patterns", "Plugins", "Video", "Particle Tracking", "Clamping", "Blank"]
        w1579 = refnum<vi> refnum  # Image
        # "This allows us to disable custom mouse-handling for certain tabs.  It can also be done from within the \"mouse down\" event case."
        n364 = event-data() -> ("NewVal"=w1575:T6)  [unwired: 1 in, 3 out]
        n365 = Equal?(x=w1574, y=w1575) -> (x = y?=w1573:bool[])
        n366 = Or Array Elements(Boolean array=w1573) -> (logical OR=w1572:bool)
        n367 = Not(x=w1572) -> (.not. x?=w1571:bool)
        n368 = Select(t=w1578, s=w1571, f=w1579) -> (s? t:f=w1580:refnum<vi>)
        n369 = register-events(reference=w1582, w1580, w1579, w1579, w1579) -> (reference out=w1581:refnum<event-registration>)  [unwired: 1 in, 1 out]
      }
      event Menu Selection (User) {
        n370 = event-data() -> ("ItemTag"=w1590:string, "MenuRef"=w1583:refnum<k9>)  [unwired: 1 in]
        n371 = case shown="\"ToggleSavingData\"" w1590 {
          tunnel: w1594 -> [w1598 w1608 w1617 w1631 w1650 w1654 w1657 w1664 w1671 w1673 w1676 w1705 w1731 w1752 w1763 w1774 w1777 w1779 w1784 w1787]
          tunnel: w1593 -> [w1597 w1607 w1616 w1640 w1649 w1653 w1655 w1662 w1670 w1672 w1675 w1704 w1730 w1751 w1762 w1773 w1776 w1780 w1785 w1786]
          tunnel: [w1598 w1608 w1617 w1631 w1648 w1651 w1657 w1664 w1671 w1673 w1676 w1705 w1731 w1752 w1763 w1774 w1777 w1779 w1784 w1787] -> w1592
          tunnel: [w1597 w1607 w1616 w1640 w1647 w1652 w1656 w1663 w1669 w1674 w1677 w1704 w1730 w1751 w1762 w1773 w1776 w1780 w1785 w1786] -> w1591
          tunnel: [_ _ _ _ TRUE _ _ _ _ _ _ _ _ _ _ _ _ _ _ _] -> w1585
          tunnel: w1584 -> [_ _ _ _ _ _ _ _ _ _ _ w1703 w1729 w1743 _ _ _ _ _ _]
          tunnel: w1583 -> [_ _ _ _ _ _ _ _ _ _ _ w1694 w1723 w1746 w1757 w1768 _ _ _ _]
          frame "ToggleSavingData" {
            # "Data is saved from the middle loop: look there for an explanation."
            n372 = local read "Save Video"() -> (w1596:bool)
            n373 = Not(x=w1596) -> (.not. x?=w1595:bool)
            n374 = local write "Save Video"(w1595) -> ()
          }
          frame "SaveStateToFile" {
            # "Save the current settings (i.e. the values of all the controls in VIs that have [Red Tweezers Save Settings] in their documentation string) to a file."
            n375 = call "File Dialog"("prompt"="Please select a location to save the settings", "button label"="Save", "default name"="red_tweezers_settings.xml", "pattern (all files)"="*.xml" ("pattern label"), "pattern label"="XML Settings Files") -> ("selected path"=w1606:path, "cancelled"=w1599:bool)  [unwired: 7 in, 2 out]
            n376 = Not(x=w1599) -> (.not. x?=w1600:bool)
            n377 = case shown="True" w1600 {
              tunnel: w1606 -> [_ w1610]
              frame False {
              }
              frame True {
                n378 = Path To String(path=w1610) -> (string=w1609:string)
                n379 = call "settings_save_to_file.vi"("XML File Path"=w1610) -> ()  [unwired: 11 in]
                n380 = call "settings_filename_to_registry.vi"("Last Used Settings File"=w1609) -> ()  [unwired: 11 in]
              }
            }
          }
          frame "SaveStateToCurrentFile" {
            # "As SaveStateToFile, but using the current file (i.e. Save not Save As...)."
            n381 = global read "red_tweezers_globals_INTERNAL_VOLATILE.vi" "Current Settings File"() -> (w1615:path)
            n382 = call <vilib>:"Check if File or Folder Exists.vi"("path"=w1615) -> ("file or folder exists?"=w1614:bool, "dup path"=w1613:path)  [unwired: 8 in, 1 out]
            n383 = case shown="True" w1614 {
              selector: w1614 -> [_ w1628]
              tunnel: w1613 -> [_ w1629]
              tunnel: [w1620 w1629] -> w1612
              tunnel: [w1621 w1628] -> w1611
              frame False {
                n384 = call "File Dialog3"("prompt"="Please select a location to save the settings", "button label"="Save", "default name"="red_tweezers_settings.xml", "pattern (all files)"="*.xml" ("pattern label"), "pattern label"="XML Settings Files") -> ("selected path"=w1620:path, "cancelled"=w1627:bool)  [unwired: 7 in, 2 out]
                n385 = Not(x=w1627) -> (.not. x?=w1621:bool)
              }
              frame True {
              }
            }
            n386 = case shown="True" w1611 {
              tunnel: w1612 -> [_ w1619]
              frame False {
              }
              frame True {
                n387 = Path To String(path=w1619) -> (string=w1618:string)
                n388 = call "settings_save_to_file.vi"("XML File Path"=w1619) -> ()  [unwired: 11 in]
                n389 = call "settings_filename_to_registry.vi"("Last Used Settings File"=w1618) -> ()  [unwired: 11 in]
              }
            }
          }
          frame "LoadStateFromFile" {
            # "Load a file, and use it to reset the values of all the front panel controls."
            # "We need to re-run the initialisation stuff in UDP sender after changing settings\n(for example, this synchronises the settings like camera pixel size with the\nrelevant global variable)"
            n390 = call "File Dialog2"("prompt"="Please select a settings file", "button label"="Open", "default name"="red_tweezers_settings.xml", "pattern (all files)"="*.xml" ("pattern label"), "pattern label"="XML Settings Files") -> ("selected path"=w1632:path, "cancelled"=w1639:bool)  [unwired: 7 in, 2 out]
            n391 = Not(x=w1639) -> (.not. x?=w1638:bool)
            n392 = case shown="False" w1638 {
              selector: w1638 -> [w1641 w1642]
              tunnel: w1632 -> [_ w1643]
              tunnel: [w1641 w1642] -> w1630
              frame False {
              }
              frame True {
                n393 = call "settings_load_from_file.vi"("XML File Path"=w1643) -> ()  [unwired: 9 in, 2 out]
                n394 = Path To String(path=w1643) -> (string=w1644:string)
                n395 = call "settings_filename_to_registry.vi"("Last Used Settings File"=w1644) -> ()  [unwired: 11 in]
              }
            }
            n396 = call "UDP Sender generic_2.vi"("re-initialise"=w1630, "Spots"=w1631) -> ()  [unwired: 1 in, 1 out]
          }
          frame "Undo" {
            # "This should get the last undo vector and replace the spots with it :)"
            n397 = call "red_tweezers_UNDO.vi"("Selection/Group"=w1649, "Undo/Store (store, False)"=TRUE, "Spots"=w1650) -> ("Selection/Group Out (Undo only)"=w1647:T9[], "Spots Out (Undo only)"=w1648:T3[])  [unwired: 7 in]
          }
          frame "Delete" {
            n398 = call "delete_selected_spots.vi"("Selection/Group 3"=w1653, "Spots 3"=w1654) -> ("Selection/Group 2"=w1652:T9[], "Spots 2"=w1651:T3[])  [unwired: 4 in]
          }
          frame "SelectAllSpots" {
            n399 = for {
              tunnel: w1655 -> [w1660] mode=indexing
              tunnel: [w1661] -> w1656 mode=indexing
              n400 = Unbundle(w1660) -> ("Group ID"=w1659:i32)  [unwired: 1 out]
              n401 = Bundle(cluster=w1660, "Group ID"=w1659, "Selected"=TRUE ("Label.Visible")) -> (w1661:T9)
            }
          }
          frame "SelectNoSpots" {
            n402 = for {
              tunnel: w1662 -> [w1667] mode=indexing
              tunnel: [w1668] -> w1663 mode=indexing
              n403 = Unbundle(w1667) -> ("Group ID"=w1666:i32)  [unwired: 1 out]
              n404 = Bundle(cluster=w1667, "Group ID"=w1666, "Selected"=FALSE ("Label.Visible")) -> (w1668:T9)
            }
          }
          frame "SelectSpecificSpots" {
            n405 = call "select_by_id.vi"("Selection/Group"=w1670, "Spots"=w1671) -> ("Selection/Group Out"=w1669:T9[])  [unwired: 9 in]
          }
          frame "Group" {
            # "Group the currently selected spots"
            n406 = call "group_selected_spots.vi"("Selection/Group 2"=w1672) -> ("Array"=w1674:T9[])
          }
          frame "Ungroup" {
            # "Ungroup the currently selected spots"
            n407 = for {
              tunnel: [w1681] -> w1677 mode=indexing
              tunnel: w1675 -> [w1680] mode=indexing
              tunnel: 0 -> [w1679]
              n408 = Unbundle(w1680) -> ("Selected"=w1682:bool)  [unwired: 1 out]
              n409 = case shown="False" w1682 {
                tunnel: [w1683 w1686] -> w1681
                tunnel: w1680 -> [w1683 w1685]
                tunnel: w1679 -> [_ w1684]
                frame False {
                }
                frame True {
                  n410 = Unbundle(w1685) -> ("Selected"=w1687:bool)  [unwired: 1 out]
                  n411 = Bundle(cluster=w1685, "Group ID"=w1684, "Selected"=w1687) -> (w1686:T9)
                }
              }
            }
          }
          frame "ZoomIn" {
            w1688 = "ZoomToFit" ("item tag")
            # "turn off \"zoom to fit\""
            n412 = property class="ImageControl"(reference=w1703) -> (reference out=w1697:refnum<vi>, "ZoomSingle"=w1702:cluster{"X":sgl, "Y":sgl}, "Image Center Position"=w1695:cluster{"X":u32, "Y":u32})  [unwired: 1 in, 1 out]
            n413 = Unbundle(w1702) -> ("X"=w1700:sgl)  [unwired: 1 out]
            n414 = Round To Nearest(number=w1700) -> (nearest integer value=w1696:sgl)
            n415 = Greater Than 0?(x=w1696) -> (x > 0?=w1701:bool)
            n416 = case shown="True" w1701 {
              tunnel: w1700 -> [w1710 w1713]
              tunnel: [w1709 w1711] -> w1699
              frame False {
                n417 = Reciprocal(x=w1710) -> (1/x=w1707:sgl)
                n418 = Round Toward +Infinity(x=w1707) -> (ceil(x): smallest int >= x=w1708:sgl)
                n419 = Decrement(x=w1708) -> (x-1=w1706:sgl)
                n420 = Reciprocal(x=w1706) -> (1/x=w1709:sgl)
              }
              frame True {
                n421 = Round Toward -Infinity(1:w1713) -> (0:w1712:sgl)
                n422 = Increment(x=w1712) -> (x+1=w1711:sgl)
              }
            }
            n423 = Bundle(w1699, w1699) -> (w1698:cluster{sgl, sgl})  [unwired: 1 in]
            n424 = property class="ImageControl"(reference=w1697, "ZoomSingle"=w1698, "Image Center Position"=w1695) -> ()  [unwired: 1 in, 2 out]
            n425 = Get Menu Item Info(7:w1688, 11:w1694) -> (1:w1691:bool, 2:w1692:string, 3:w1693:refnum<k9>, 6:w1690:T23)  [unwired: 1 in, 3 out]
            n426 = Set Menu Item Info(4:w1690, 6:FALSE ("checked"), 7:w1688, 9:w1691, 10:w1692, 11:w1693) -> ()  [unwired: 1 in, 2 out]
          }
          frame "ZoomOut" {
            w1717 = "ZoomToFit" ("item tag")
            # "turn off \"zoom to fit\""
            n427 = property class="ImageControl"(reference=w1729) -> (reference out=w1725:refnum<vi>, "ZoomSingle"=w1728:cluster{"X":sgl, "Y":sgl}, "Image Center Position"=w1724:cluster{"X":u32, "Y":u32})  [unwired: 1 in, 1 out]
            n428 = Unbundle(w1728) -> ("X"=w1714:sgl)  [unwired: 1 out]
            n429 = Greater?(x=w1714, y=1.0) -> (0:w1716:bool)
            n430 = case shown="False" w1716 {
              tunnel: w1714 -> [w1738 w1741]
              tunnel: [w1737 w1739] -> w1727
              frame False {
                n431 = Reciprocal(x=w1738) -> (1/x=w1735:sgl)
                n432 = Add(x=w1735, y=sgl 0.01 ("x")) -> (x+y=w1733:sgl)
                n433 = Round Toward -Infinity(1:w1733) -> (0:w1736:sgl)
                n434 = Increment(x=w1736) -> (x+1=w1734:sgl)
                n435 = Reciprocal(x=w1734) -> (1/x=w1737:sgl)
              }
              frame True {
                n436 = Round Toward +Infinity(x=w1741) -> (ceil(x): smallest int >= x=w1740:sgl)
                n437 = Decrement(x=w1740) -> (x-1=w1739:sgl)
              }
            }
            n438 = Bundle(w1727, w1727) -> (w1726:cluster{sgl, sgl})  [unwired: 1 in]
            n439 = property class="ImageControl"(reference=w1725, "ZoomSingle"=w1726, "Image Center Position"=w1724) -> ()  [unwired: 1 in, 2 out]
            n440 = Get Menu Item Info(7:w1717, 11:w1723) -> (1:w1720:bool, 2:w1721:string, 3:w1722:refnum<k9>, 6:w1719:T23)  [unwired: 1 in, 3 out]
            n441 = Set Menu Item Info(4:w1719, 6:FALSE ("checked"), 7:w1717, 9:w1720, 10:w1721, 11:w1722) -> ()  [unwired: 1 in, 2 out]
          }
          frame "ZoomToFit" {
            w1747 = "ZoomToFit" ("item tag")
            # "and make sure the image obeys the result"
            # "Toggle menu checkmark"
            n442 = Get Menu Item Info(7:w1747, 11:w1746) -> (1:w1745:bool, 2:w1749:string, 3:w1750:refnum<k9>, 4:w1744:bool, 6:w1748:T23)  [unwired: 1 in, 2 out]
            n443 = Not(x=w1744) -> (.not. x?=w1742:bool)
            n444 = Set Menu Item Info(4:w1748, 6:w1742, 7:w1747, 9:w1745, 10:w1749, 11:w1750) -> ()  [unwired: 1 in, 2 out]
            n445 = property class="ImageControl"(reference=w1743, "Zoom to Fit Mode"=w1742) -> ()  [unwired: 1 in, 2 out]
          }
          frame "ShowGrid" {
            w1758 = "ShowGrid" ("item tag")
            # "Toggle menu checkmark"
            n446 = Get Menu Item Info(7:w1758, 11:w1757) -> (1:w1756:bool, 2:w1760:string, 3:w1761:refnum<k9>, 4:w1755:bool, 6:w1759:T23)  [unwired: 1 in, 2 out]
            n447 = Not(x=w1755) -> (.not. x?=w1754:bool)
            n448 = Set Menu Item Info(4:w1759, 6:w1754, 7:w1758, 9:w1756, 10:w1760, 11:w1761) -> ()  [unwired: 1 in, 2 out]
            n449 = call "grid_and_guides.vi"("Boolean"=w1754, "Operation"=T16."Set grid visibility") -> ()  [unwired: 9 in, 1 out]
          }
          frame "ShowGuides" {
            w1769 = "ShowGuides" ("item tag")
            # "Toggle menu checkmark"
            n450 = Get Menu Item Info(7:w1769, 11:w1768) -> (1:w1767:bool, 2:w1771:string, 3:w1772:refnum<k9>, 4:w1766:bool, 6:w1770:T23)  [unwired: 1 in, 2 out]
            n451 = Not(x=w1766) -> (.not. x?=w1765:bool)
            n452 = Set Menu Item Info(4:w1770, 6:w1765, 7:w1769, 9:w1767, 10:w1771, 11:w1772) -> ()  [unwired: 1 in, 2 out]
            n453 = call "grid_and_guides.vi"("Boolean"=w1765, "Operation"=T16."Set guide visibility") -> ()  [unwired: 9 in, 1 out]
          }
          frame "ConfigureGridAndGuides" {
            n454 = call "grid_and_guides.vi"("Operation"=T16."Show front panel") -> ()  [unwired: 10 in, 1 out]
          }
          frame "ShowSettings" {
            n455 = call "UDP Sender generic_2.vi"("Show panel"=TRUE, "Spots"=w1779) -> ()  [unwired: 1 in, 1 out]
          }
          frame "CameraSettings" {
            n456 = global read "red_tweezers_globals_INTERNAL_VOLATILE.vi" "Current Camera VI"() -> (w1782:path)
            n457 = Open VI Reference(vi path=w1782) -> (vi reference=w1781:refnum<vi>)  [unwired: 5 in, 1 out]
            n458 = property class="VI"(reference=w1781, "Front Panel.Open"=TRUE ("Front Panel Window:Open")) -> ()  [unwired: 1 in, 2 out]
          }
          frame Default {
          }
        }
      }
      event Mouse Down? {
        # "We don't process clicks when the user is on the video tab, so that we can set ROIs."
        # "When the mouse button goes down over the image, we save where it went down, etc. and wait to see what happens next.  We also register to be told when the mouse leaves the control, goes up, or moves.  \"click\" or \"drag\" are only detected once the mouse moves or goes up."
        n459 = event-data() -> ("Coords"=w1802:T24, "Button"=w1797:u16, "Mods"=w1806:cluster{"Double Click":bool, "Menu Key":bool}, "PlatMods"=w1805:T25)  [unwired: 1 in]
        n460 = call "mouse_to_image_coords.vi"("Mouse Coords (screen/pane units)"=w1802, "Image Control"=w1798) -> ("Cursor is on Display Area"=w1796:bool, "Mouse Coords (image pixels)"=w1801:cluster{dbl, dbl})  [unwired: 4 in]
        n461 = disable-structure shown="Enabled" {
          disable-tunnel: w1797 -> [w1814 _]
          disable-tunnel: w1796 -> [w1812 w1815]
          disable-tunnel: [w1811 w1815] -> w1792
          frame Enabled {
            n462 = Equal?(x=u16 1, y=w1814) -> (x = y?=w1813:bool)
            n463 = And(x=w1812, y=w1813) -> (x .and. y?=w1811:bool)
          }
          frame Disabled {
            # "use other pane to allow right-clicking on image"
          }
        }
        n464 = local read "Tab"() -> (w1793:T6)
        n465 = Not Equal?(x=w1793, y=T17."Video" ("Tab")) -> (x != y?=w1791:bool)
        n466 = And(x=w1792, y=w1791) -> (x .and. y?=w1790:bool)
        n467 = case shown="False" w1790 {
          tunnel: w1809 -> [w1818 w1829]
          tunnel: [T13 {"Button Down"=FALSE, "Dragging"=FALSE, "Position (Image Pixels)"={"X"=0.0, "Y"=0.0}, "Previous Position (Image Pixels)"={"X"=0.0, "Y"=0.0}, "Button"=0, "Mods"={"Double Click"=FALSE, "Menu Key"=FALSE}, "PlatMods"={"Shift"=FALSE, "Ctrl"=FALSE, "Alt"=FALSE, "Cmd"=FALSE, "Opt"=FALSE}} w1828] -> w1808
          tunnel: [w1818 w1825] -> w1807
          tunnel: w1797 -> [_ w1824]
          tunnel: w1806 -> [_ w1823]
          tunnel: w1805 -> [_ w1822]
          tunnel: w1801 -> [_ w1821]
          tunnel: [FALSE TRUE] -> w1800
          tunnel: w1798 -> [_ w1819]
          frame False {
            # "If the user clicked on a scrollbar, ignore it and let LabVIEW handle it. (this keeps the scrollbars working)"
          }
          frame True {
            w1827 = FALSE  # Dragging
            w1826 = TRUE  # Button Down
            n468 = register-events(reference=w1829, w1819, w1819, w1819, w1819) -> (reference out=w1825:refnum<event-registration>)  [unwired: 1 in, 1 out]
            n469 = Bundle("Button Down"=w1826, "Dragging"=w1827, "Mouse Coords (image pixels)"=w1821, "Mouse Coords (image pixels)"=w1821, "Button"=w1824, "Mods"=w1823, "PlatMods"=w1822) -> (w1828:T26)  [unwired: 1 in]
          }
        }
        n470 = Array Size(array=w1788) -> (size(s)=w1789:i32)
        n471 = local write "Selection/Group"(w1788) -> ()
        n472 = local write "# of Spots"(w1789) -> ()
        n473 = event-data("Discard?"=w1800) -> ()  [unwired: 4 in, 1 out]
      }
      event Mouse Leave {
        w1836 = refnum<vi> refnum  # Dummy
        # "When the mouse leaves, we reset things."
        n474 = event-data() -> ()  [unwired: 1 in, 2 out]
        n475 = register-events(reference=w1837, w1835, w1836, w1836, w1836) -> (reference out=w1834:refnum<event-registration>)  [unwired: 1 in, 1 out]
      }
      event Mouse Up {
        w1856 = refnum<vi> refnum  # Dummy
        # "Double clicking adds a spot at the mouse position."
        # "deregister"
        # "If we get here the mouse has gone down and up again.  If we've not moved in between, we have a Click.\nEither way we're no longer interested in mouse leave/move/up events."
        n476 = event-data() -> ("Mods"=w1843:cluster{"Double Click":bool, "Menu Key":bool})  [unwired: 1 in, 5 out]
        n477 = Unbundle By Name(w1849) -> ("Dragging"=w1858:bool)
        n478 = Unbundle By Name(w1843) -> ("Double Click"=w1840:bool)
        n479 = Not(x=w1858) -> (.not. x?=w1857:bool)
        n480 = Not(x=w1845) -> (.not. x?=w1847:bool)
        n481 = And(x=w1857, y=w1847) -> (x .and. y?=w1841:bool)
        n482 = case shown="True" w1841 {
          tunnel: w1849 -> [_ w1864]
          tunnel: w1851 -> [w1859 w1863]
          tunnel: w1850 -> [w1860 w1866]
          tunnel: [w1860 w1865] -> w1852
          tunnel: w1840 -> [_ w1861]
          tunnel: [w1859 w1862] -> w1842
          frame False {
          }
          frame True {
            n483 = case shown="True" w1861 {
              tunnel: w1866 -> [w1873 w1923]
              tunnel: [w1871 w1929] -> w1865
              tunnel: w1863 -> [w1867 w1930]
              tunnel: w1864 -> [w1870 w1925]
              tunnel: [w1867 w1921] -> w1862
              frame False {
                w1877 = 400.0  # 20^2 px
                # "If the user clicked, determine which spots should be selected: if we've clicked a spot/group then select it.  Shift-clicking toggles selection for that spot, and leaves the rest of the selection unchanged."
                # "check we're close enough"
                # "find closest"
                n484 = Unbundle By Name(w1870) -> ("Position (Image Pixels)"=w1869:cluster{"X":dbl, "Y":dbl}, "PlatMods.Shift"=w1868:bool)
                n485 = for {
                  tunnel: [w1913] -> w1875 mode=indexing
                  tunnel: w1869 -> [w1912]
                  tunnel: w1867 -> [w1911] mode=indexing
                  # "calculate distances between mouse position and spot positions"
                  n486 = call "extract_position.vi"("Spot"=w1911) -> ("Position"=w1910:cluster{"x":dbl, "y":dbl, "z":dbl})
                  n487 = call "coords_real_to_image_currentview.vi"("Position (real coords)"=w1910) -> ("Position (pixels, relative to the top left of the image)"=w1909:cluster{dbl, dbl})  [unwired: 7 in, 1 out]
                  n488 = Subtract(x=w1909, y=w1912) -> (x-y=w1916:cluster{dbl, dbl})
                  n489 = Multiply(x=w1916, y=w1916) -> (x*y=w1915:cluster{dbl, dbl})
                  n490 = Cluster To Array(cluster=w1915) -> (array=w1914:dbl[])
                  n491 = Add Array Elements(numeric array=w1914) -> (sum=w1913:dbl)
                }
                n492 = Array Max & Min(array=w1875) -> (min value=w1876:dbl, min index (indices)=w1872:i32)  [unwired: 2 out]
                n493 = Less Or Equal?(x=w1876, y=w1877) -> (x <= y?=w1874:bool)
                n494 = case shown="True" w1874 {
                  tunnel: w1873 -> [w1878 w1885]
                  tunnel: w1872 -> [_ w1879]
                  tunnel: w1868 -> [_ w1881]
                  tunnel: [w1878 w1880] -> w1871
                  frame False {
                    # "If we didn't click a spot, do nothing."
                  }
                  frame True {
                    # "If the spot is in a group, act on all spots in that group, not just the spot we clicked."
                    # "This case statement toggles the selection of the spot/group we clicked, and leaves other spots unchanged if we're holding shift.  Otherwise, we select the spot/group that was clicked and deselect everything else."
                    n495 = stacked-sequence {
                      tunnel: w1879 -> [_ w1887]
                      frame #0 {
                        n496 = local read "Current Spot #"() -> (→"Prev Current Spot":dbl)
                      }
                      frame #1 {
                        "Current Spot #" <- w1887
                      }
                    }
                    n497 = Index Array(array=w1885, index=w1879) -> (element=w1884:T9)
                    n498 = Unbundle(w1884) -> ("Group ID"=w1882:i32)  [unwired: 1 out]
                    n499 = Greater Than 0?(x=w1882) -> (x > 0?=w1883:bool)
                    n500 = for {
                      tunnel: w1885 -> [w1898] mode=indexing
                      tunnel: w1883 -> [w1895]
                      tunnel: w1882 -> [w1894]
                      tunnel: w1879 -> [w1893]
                      tunnel: w1881 -> [w1891]
                      tunnel: [w1889] -> w1880 mode=indexing
                      i -> [w1892]
                      n501 = Unbundle(w1898) -> ("Group ID"=w1888:i32, "Selected"=w1896:bool)
                      n502 = case shown="True" w1895 {
                        tunnel: w1888 -> [_ w1902]
                        tunnel: [w1900 w1904] -> w1890
                        tunnel: w1894 -> [_ w1903]
                        tunnel: w1893 -> [w1901 _]
                        tunnel: w1892 -> [w1899 _]
                        frame False {
                          n503 = Equal?(x=w1899, y=w1901) -> (x = y?=w1900:bool)
                        }
                        frame True {
                          n504 = Equal?(x=w1902, y=w1903) -> (x = y?=w1904:bool)
                        }
                      }
                      n505 = case shown="True" w1891 {
                        tunnel: [w1905 w1906] -> w1897
                        tunnel: w1896 -> [_ w1907]
                        tunnel: w1890 -> [w1905 w1908]
                        frame False {
                        }
                        frame True {
                          n506 = Exclusive Or(1:w1908, 2:w1907) -> (0:w1906:bool)
                        }
                      }
                      n507 = Bundle("Group ID"=w1888, w1897) -> (w1889:cluster{"Group ID":i32, bool})  [unwired: 1 out]
                    }
                  }
                }
              }
              frame True {
                # "convert mouse position to real coords, and add a spot there."
                # "Double-click detected"
                n508 = Unbundle By Name(w1925) -> ("Position (Image Pixels)"=w1924:cluster{"X":dbl, "Y":dbl})
                n509 = for {
                  tunnel: w1923 -> [w1933] mode=indexing
                  tunnel: [w1932] -> w1922 mode=indexing
                  n510 = Bundle(cluster=w1933, "Selected"=FALSE) -> (w1932:T9)  [unwired: 1 in]
                }
                n511 = call "coords_image_to_real_currentimage.vi"("Position (pixels on image)"=w1924) -> ("Position (real coords)"=w1926:cluster{dbl, dbl, "Z":dbl})  [unwired: 9 in]
                n512 = call "replace_position.vi"("Position"=w1926) -> ("Spot"=w1928:T3)  [unwired: 3 in]
                n513 = Build Array (concatenate)(w1930, w1928) -> (w1921:T3[])
                n514 = Build Array (concatenate)(w1922, T9 {"Group ID"=0, "Selected"=TRUE} ("selection_element")) -> (w1929:T9[])
                n515 = Array Size(array=w1921) -> (size(s)=w1920:i32)
                n516 = local write "Induce check"(TRUE) -> ()
                n517 = Subtract(x=w1920, y=1) -> (x-y=w1919:i32)
                n518 = local write "Current Spot #"(w1919) -> ()
              }
            }
          }
        }
        n519 = register-events(reference=w1854, w1853, w1856, w1856, w1856) -> (reference out=w1855:refnum<event-registration>)  [unwired: 1 in, 1 out]
      }
      event Mouse Move {
        n520 = event-data() -> ("Coords"=w1948:T24)  [unwired: 1 in, 2 out]
        n521 = call "mouse_to_image_coords.vi"("Mouse Coords (screen/pane units)"=w1948, "Image Control"=w1947) -> ("Mouse Coords (image pixels)"=w1939:cluster{dbl, dbl})  [unwired: 4 in, 1 out]
        n522 = Not(x=w1938) -> (.not. x?=w1943:bool)
        n523 = case shown="True" w1943 {
          tunnel: w1941 -> [_ w1961]
          tunnel: w1946 -> [w1953 w1963]
          tunnel: w1945 -> [w1952 w1962]
          tunnel: [w1952 w1962] -> w1934
          tunnel: [w1953 w1964] -> w1944
          tunnel: w1939 -> [_ w1955]
          tunnel: w1935 -> [_ w1954]
          frame False {
          }
          frame True {
            # "this is the displacement of the mouse, since the last iteration, in \"real\" coordinates (NB the conversions go before subtracting, as it may involve adding a constant as well as multiplying, which would confuse things as we're only interested in displacements here."
            # "The \"position\" local variable is there just in case we're on the \"current spot\" tab, so that the position updates nicely"
            # "If the user is dragging, translate the spots.\nHolding down shift causes the mouse's motion to be transformed into scaling about the centroid of the spots and rotation about the same point"
            n524 = Unbundle By Name(w1961) -> ("Position (Image Pixels)"=w1956:cluster{"X":dbl, "Y":dbl})
            n525 = call "find_centroid.vi"("Selection and Groups"=w1962, "Spots"=w1963) -> ("centroid"=w1957:cluster{"x":dbl, "y":dbl, "z":dbl})  [unwired: 2 in, 4 out]
            n526 = Unbundle By Name(w1961) -> ("PlatMods.Shift"=w1960:bool)
            n527 = disable-structure shown="Disabled" {
              disable-tunnel: w1957 -> [w1965 _]
              frame Disabled {
                n528 = local write "Position"(w1965) -> ()
              }
              frame Enabled {
              }
            }
            n529 = call "coords_image_to_real_currentimage.vi"("Position (pixels on image)"=w1955) -> ("Position (real coords)"=w1958:cluster{dbl, dbl, "Z":dbl})  [unwired: 9 in]
            n530 = call "coords_image_to_real_currentimage.vi"("Position (pixels on image)"=w1956) -> ("Position (real coords)"=w1959:cluster{dbl, dbl, "Z":dbl})  [unwired: 9 in]
            n531 = case shown="False" w1960 {
              tunnel: [w1970 w2244] -> w1964
              tunnel: w1963 -> [w1976 w2245]
              tunnel: w1962 -> [w1975 w2243]
              tunnel: w1959 -> [w1974 w2230]
              tunnel: w1957 -> [_ w2240]
              tunnel: w1958 -> [w1971 w2231]
              tunnel: w1954 -> [_ _]
              frame False {
                # "Spot Checker passes on information for the bubble collision,system so proper calculations can be made."
                n532 = while {
                  tunnel: w1974 -> [w2015]
                  tunnel: [w2005] -> w1972
                  tunnel: w1971 -> [w2004]
                  i -> [w1998]
                  stop <- w2000 stop-if-true
                  w1990 = 0
                  # "This while loop statement makes sure\nthat every spot gets checked before \nallowing any spot to move."
                  # "Buffer zone controls the amount of space between the\ncenter of a spot compared to the center of another spot.\nThis is used to prevent bubbles from colliding with each other."
                  # "Projected distance calculates the distance between two spots- this is used for when a \"hit\" occurs. If the projected distance becomes larger than the previous distance, the program will assume that the spot is being pulled from the buffer zone and as a result will allow the bubble to exit."
                  # "This subVI leads to the distance function, which outputs the distance between a spot being checked compared to the current spot number."
                  n533 = control-ref of="Value Check"() -> (w1995:refnum<vi>)
                  n534 = control-ref of="ID num check"() -> (w1994:refnum<vi>)
                  n535 = control-ref of="Spot Checker"() -> (w2011:refnum<vi>)
                  n536 = Subtract(x=w2004, y=w2015) -> (x-y=w2005:cluster{dbl, dbl, "Z":dbl})
                  n537 = call "DistanceFunction.vi"("Condition Driver"=FALSE, "Position (real coords)"=w2015, "Current Spot Number"=w1994, "Spot Checker"=w2011, "Spot Number Being Checked"=w1995) -> ("Distance"=w1977:dbl)  [unwired: 6 in]
                  n538 = stacked-sequence {
                    tunnel: w1977 -> [_ w2020]
                    frame #0 {
                      n539 = local read "Distance"() -> (→"Previous Distance":dbl)
                    }
                    frame #1 {
                      "Distance" <- w2020
                    }
                  }
                  n540 = Unbundle(w2005) -> (→"X Displacement":dbl, →"Y Displacement":dbl)  [unwired: 1 out]
                  n541 = control-ref of="ID num check"() -> (w1996:refnum<vi>)
                  n542 = control-ref of="Spot Checker"() -> (w2009:refnum<vi>)
                  n543 = control-ref of="Y Displacement"() -> (w2007:refnum<vi>)
                  n544 = control-ref of="Value Check"() -> (w1997:refnum<vi>)
                  n545 = control-ref of="X Displacement"() -> (w2008:refnum<vi>)
                  n546 = call "ProjectedDistance.vi"("X Displacement"=w2008, "Spot Number Check"=w1997, "Current Spot #"=w1996, "Spot Checker"=w2009, "Y Displacement"=w2007) -> ("Numeric"=→"Projected Distance":dbl)  [unwired: 6 in]
                  n547 = local read "Projected Distance"() -> (w1983:dbl)
                  n548 = Multiply(x="Buffer Zone", y=2) -> (x*y=w2014:dbl)
                  n549 = Less Or Equal?(x=w1977, y=w2014) -> (x <= y?=w1984:bool)
                  n550 = Not Equal?(x=w1983, y=0) -> (x != y?=w1981:bool)
                  n551 = And(x=w1984, y=w1981) -> (x .and. y?=w1978:bool)
                  "Hit" <- w1978
                  n552 = local read "ID num check"() -> (w1991:dbl)
                  n553 = local read "Value Check"() -> (w1992:dbl)
                  n554 = Equal?(x=w1977, y=0) -> (x = y?=w1980:bool)
                  n555 = case shown="False" w1980 {
                    frame False {
                      n556 = local read "Hit"() -> (w2017:bool)
                      n557 = local write "Hit Indicator"(w2017) -> ()
                    }
                    frame True {
                      "Hit Indicator" <- FALSE
                    }
                  }
                  n558 = Equal?(x=w1991, y=w1990) -> (x = y?=w1989:bool)
                  n559 = Equal?(x=w1990, y=w1992) -> (x = y?=w1988:bool)
                  n560 = Not(x=w1978) -> ()  [unwired: 1 out]
                  n561 = And(x=w1989, y=w1988) -> (x .and. y?=w1987:bool)
                  n562 = Or(x=w1978, y=w1987) -> (x .or. y?=w1993:bool)
                  n563 = case shown="True" w1993 {
                    frame False {
                      n564 = stacked-sequence {
                        frame #0 {
                          n565 = local read "Potential Collisions"() -> (w2023:dbl)
                          n566 = local read "Spot # Check"() -> (w2025:dbl)
                          n567 = Subtract(x=w2023, y=1) -> (x-y=w2021:dbl)
                          n568 = Less Or Equal?(x=w2025, y=w2021) -> (x <= y?=w2024:bool)
                          n569 = case shown="True" w2024 {
                            frame False {
                              # "Spot # Check resets if the the number of potential collisons is more than Spot # Check."
                              n570 = local write "Spot # Check"(0) -> ()
                            }
                            frame True {
                              n571 = stacked-sequence {
                                frame #0 {
                                # "Spot # Check increments by 1 every time it is greater than the # of potential collisions."
                                n572 = local read "Spot # Check"() -> (w2029:dbl)
                                n573 = Add(x=w2029, y=1) -> (x+y=→"Spot # Check":dbl)
                                }
                                frame #1 {
                                # "Spot # Check resets if the Spot # Check is eqaul to the # of potential collisions."
                                n574 = local read "Potential Collisions"() -> (w2030:dbl)
                                n575 = local read "Spot # Check"() -> (w2031:dbl)
                                n576 = Equal?(x=w2031, y=w2030) -> (x = y?=w2032:bool)
                                n577 = case shown="True" w2032 {
                                frame False {
                                }
                                frame True {
                                n578 = local write "Spot # Check"(0) -> ()
                                }
                                }
                                }
                                frame #2 {
                                n579 = local read "Spot Checker"() -> (w2047:T3[])
                                n580 = local read "Current Spot #"() -> (w2048:dbl)
                                n581 = local read "Area to check"() -> (w2034:dbl)
                                n582 = Index Array(array=w2047, index=w2048) -> (element=w2046:T3)
                                n583 = local read "Orig Y SC"() -> (w2043:dbl)
                                n584 = Unbundle By Name(w2046) -> ("Position.x"=w2044:dbl, "Position.y"=w2042:dbl)
                                n585 = local read "Orig X SC"() -> (w2045:dbl)
                                n586 = Subtract(x=w2042, y=w2043) -> (x-y=w2035:dbl)
                                n587 = Absolute Value(x=w2035) -> (abs(x)=w2036:dbl)
                                n588 = Subtract(x=w2044, y=w2045) -> (x-y=w2038:dbl)
                                n589 = Greater?(x=w2036, y=w2034) -> (0:w2040:bool)
                                n590 = Absolute Value(x=w2038) -> (abs(x)=w2037:dbl)
                                n591 = Greater?(x=w2037, y=w2034) -> (0:w2039:bool)
                                n592 = Or(x=w2039, y=w2040) -> (x .or. y?=w2041:bool)
                                n593 = case shown="True" w2041 {
                                frame False {
                                }
                                frame True {
                                n594 = stacked-sequence {
                                frame #0 {
                                n595 = local read "Null array"() -> (w2053:dbl[])
                                n596 = local write "What to Check"(w2053) -> ()
                                n597 = local write "ID"(w2053) -> ()
                                n598 = local read "Current Spot #"() -> (w2055:dbl)
                                n599 = local write "Potential Collisions"(0) -> ()
                                n600 = local read "Spot Checker"() -> (w2054:T3[])
                                n601 = Index Array(array=w2054, index=w2055) -> (element=w2056:T3)
                                n602 = Wait (ms)(milliseconds to wait=100) -> ()  [unwired: 1 out]
                                n603 = Unbundle By Name(w2056) -> ("Position.x"=w2050:dbl, "Position.y"=w2051:dbl)
                                n604 = local write "Orig Y SC"(w2051) -> ()
                                n605 = local write "Orig X SC"(w2050) -> ()
                                }
                                frame #1 {
                                # "All this is a  statement checking whether the microrobot is within the area being checked using absolute value statements. The number of potential collisions gets added by 1 every time a bubble is detected within the area."
                                n606 = local read "# of Spots"() -> (w2057:dbl)
                                n607 = for {
                                N: w2057 -> [_]
                                tunnel: w2057 -> [w2062]
                                i -> [w2058]
                                n608 = local read "Selection/Group"() -> (w2061:T9[])
                                n609 = Index Array(array=w2061, index=w2058) -> (element=w2060:T9)
                                n610 = Unbundle By Name(w2060) -> ("Selected"=w2059:bool)
                                n611 = case shown="True" w2059 {
                                tunnel: w2062 -> [_ w2064]
                                tunnel: w2058 -> [_ w2063]
                                frame False {
                                }
                                frame True {
                                n612 = for {
                                N: w2064 -> [_]
                                tunnel: w2063 -> [w2065]
                                i -> [w2066]
                                n613 = local read "Selection/Group"() -> (w2070:T9[])
                                n614 = Index Array(array=w2070, index=w2066) -> (element=w2069:T9)
                                n615 = Unbundle By Name(w2069) -> ("Selected"=w2067:bool)
                                n616 = Not(x=w2067) -> (.not. x?=w2068:bool)
                                n617 = case shown="True" w2068 {
                                tunnel: w2066 -> [_ w2074]
                                tunnel: w2065 -> [_ w2073]
                                tunnel: w2065 -> [_ w2072]
                                frame False {
                                }
                                frame True {
                                n618 = local read "Spot Checker"() -> (w2091:T3[])
                                n619 = Index Array(array=w2091, index=w2074) -> (element=w2092:T3)
                                n620 = Index Array(array=w2091, index=w2073) -> (element=w2090:T3)
                                n621 = Unbundle By Name(w2090) -> ("Position.x"=w2087:dbl, "Position.y"=w2083:dbl)
                                n622 = Unbundle By Name(w2092) -> ("Position.x"=w2084:dbl, "Position.y"=w2080:dbl)
                                n623 = local read "Area+ Buffer"() -> (w2071:dbl)
                                n624 = Subtract(x=w2087, y=w2071) -> (x-y=w2088:dbl)
                                n625 = Greater Or Equal?(x=w2084, y=w2088) -> (x >= y?=w2089:bool)
                                n626 = Add(x=w2083, y=w2071) -> (x+y=w2082:dbl)
                                n627 = Subtract(x=w2083, y=w2071) -> (x-y=w2081:dbl)
                                n628 = Add(x=w2087, y=w2071) -> (x+y=w2085:dbl)
                                n629 = Less Or Equal?(x=w2080, y=w2082) -> (x <= y?=w2079:bool)
                                n630 = Greater Or Equal?(x=w2080, y=w2081) -> (x >= y?=w2078:bool)
                                n631 = Less Or Equal?(x=w2084, y=w2085) -> (x <= y?=w2086:bool)
                                n632 = And(x=w2089, y=w2086) -> (x .and. y?=w2076:bool)
                                n633 = And(x=w2079, y=w2078) -> (x .and. y?=w2077:bool)
                                n634 = And(x=w2076, y=w2077) -> (x .and. y?=w2075:bool)
                                n635 = case shown="True" w2075 {
                                tunnel: w2074 -> [_ _]
                                tunnel: w2074 -> [_ w2094]
                                tunnel: w2072 -> [_ w2093]
                                frame False {
                                }
                                frame True {
                                n636 = stacked-sequence {
                                tunnel: w2094 -> [w2095 _]
                                tunnel: w2093 -> [w2096 _]
                                frame #0 {
                                n637 = local read "Potential Collisions"() -> (w2099:dbl)
                                n638 = local read "What to Check"() -> (w2100:dbl[])
                                n639 = Insert Into Array(array=w2100, index=w2099, new element=w2095) -> (w2101:dbl[])
                                n640 = local read "ID"() -> (w2098:dbl[])
                                n641 = local write "What to Check"(w2101) -> ()
                                n642 = Insert Into Array(array=w2098, index=w2099, new element=w2096) -> (w2097:dbl[])
                                n643 = local write "ID"(w2097) -> ()
                                }
                                frame #1 {
                                n644 = local read "Potential Collisions"() -> (w2104:dbl)
                                n645 = Add(x=w2104, y=1) -> (x+y=w2102:dbl)
                                n646 = local write "Potential Collisions"(w2102) -> ()
                                }
                                }
                                }
                                }
                                }
                                }
                                }
                                }
                                }
                                }
                                }
                                frame #2 {
                                n647 = local read "Current Spot #"() -> (w2105:dbl)
                                n648 = local write "Prev Current Spot"(w2105) -> ()
                                }
                                }
                                }
                                }
                                }
                              }
                            }
                          }
                        }
                        frame #1 {
                          # "This updates the ID and Value being checked at the beginning of IDs and values being checked."
                          n649 = local read "Spot # Check"() -> (w2108:dbl)
                          n650 = local read "What to Check"() -> (w2109:dbl[])
                          n651 = local read "ID"() -> (w2110:dbl[])
                          n652 = Index Array(array=w2110, index=w2108) -> (element=w2107:dbl)
                          n653 = Index Array(array=w2109, index=w2108) -> (element=w2106:dbl)
                          n654 = local write "Value Check"(w2106) -> ()
                          n655 = local write "ID num check"(w2107) -> ()
                        }
                      }
                    }
                    frame True {
                      n656 = stacked-sequence {
                        frame #0 {
                          # "This section activate a case statement which allows us to change the area being checked. Orig X/Y SC holds the position of the area to check and changes after the bubble exits the area beig checked."
                          # "This statement controls the areas selected and finds which bubbles needs to be checked. This activates when the bubble\nmoves out of the area specified."
                          n657 = local read "# of Spots"() -> (w2130:dbl)
                          n658 = local read "Current Spot #"() -> (w2129:dbl)
                          n659 = Subtract(x=w2130, y=1) -> (x-y=w2131:dbl)
                          n660 = Equal?(x=w2129, y=w2131) -> (x = y?=w2127:bool)
                          n661 = case shown="True" w2127 {
                            tunnel: [w2190 w2193] -> w2128
                            frame True {
                              n662 = local read "# of Spots"() -> (w2191:dbl)
                              n663 = Subtract(x=w2191, y=2) -> (x-y=w2190:dbl)
                            }
                            frame False {
                              n664 = local read "# of Spots"() -> (w2192:dbl)
                              n665 = Subtract(x=w2192, y=1) -> (x-y=w2193:dbl)
                            }
                          }
                          "Maximum" <- w2128
                          n666 = local read "Spot Checker"() -> (w2126:T3[])
                          n667 = local read "Current Spot #"() -> (w2125:dbl)
                          n668 = Index Array(array=w2126, index=w2125) -> (element=w2124:T3)
                          n669 = Unbundle By Name(w2124) -> ("Position.x"=w2123:dbl, "Position.y"=w2122:dbl)
                          n670 = local read "Orig Y SC"() -> (w2120:dbl)
                          n671 = local read "Orig X SC"() -> (w2121:dbl)
                          n672 = Subtract(x=w2122, y=w2120) -> (x-y=w2117:dbl)
                          n673 = Subtract(x=w2123, y=w2121) -> (x-y=w2119:dbl)
                          n674 = Absolute Value(x=w2117) -> (abs(x)=w2116:dbl)
                          n675 = Absolute Value(x=w2119) -> (abs(x)=w2118:dbl)
                          n676 = local read "Area to check"() -> (w2112:dbl)
                          n677 = local read "Area to check"() -> (w2111:dbl)
                          n678 = Greater?(x=w2118, y=w2112) -> (0:w2115:bool)
                          n679 = Greater?(x=w2116, y=w2111) -> (0:w2114:bool)
                          n680 = Or(x=w2115, y=w2114) -> (x .or. y?=w2113:bool)
                          n681 = case shown="True" w2113 {
                            frame False {
                            }
                            frame True {
                              n682 = stacked-sequence {
                                frame #0 {
                                # "A small time delay of 100 ms is provided to allow the data to pass throguh properly."
                                n683 = Wait (ms)(milliseconds to wait=100) -> ()  [unwired: 1 out]
                                n684 = local read "Null array"() -> (→"What to Check" →"ID":dbl[])
                                n685 = local read "Spot Checker"() -> (w2138:T3[])
                                n686 = local read "Current Spot #"() -> (w2137:dbl)
                                n687 = Index Array(array=w2138, index=w2137) -> (element=w2136:T3)
                                n688 = Unbundle By Name(w2136) -> ("Position.x"=→"Orig X SC":dbl, "Position.y"=→"Orig Y SC":dbl)
                                "Potential Collisions" <- 0
                                }
                                frame #1 {
                                n689 = local read "# of Spots"() -> (w2141:dbl)
                                n690 = for {
                                N: w2141 -> [_]
                                tunnel: w2141 -> [w2146]
                                i -> [w2142]
                                n691 = local read "Selection/Group"() -> (w2145:T9[])
                                n692 = Index Array(array=w2145, index=w2142) -> (element=w2144:T9)
                                n693 = Unbundle By Name(w2144) -> ("Selected"=w2143:bool)
                                n694 = case shown="True" w2143 {
                                tunnel: w2146 -> [_ w2148]
                                tunnel: w2142 -> [_ w2147]
                                frame False {
                                }
                                frame True {
                                n695 = for {
                                N: w2148 -> [_]
                                tunnel: w2147 -> [w2149]
                                i -> [w2150]
                                n696 = local read "Selection/Group"() -> (w2154:T9[])
                                n697 = Index Array(array=w2154, index=w2150) -> (element=w2153:T9)
                                n698 = Unbundle By Name(w2153) -> ("Selected"=w2151:bool)
                                n699 = Not(x=w2151) -> (.not. x?=w2152:bool)
                                n700 = case shown="True" w2152 {
                                tunnel: w2150 -> [_ w2158]
                                tunnel: w2149 -> [_ w2157]
                                tunnel: w2149 -> [_ w2156]
                                frame False {
                                }
                                frame True {
                                n701 = local read "Spot Checker"() -> (w2175:T3[])
                                n702 = Index Array(array=w2175, index=w2158) -> (element=w2176:T3)
                                n703 = Index Array(array=w2175, index=w2157) -> (element=w2174:T3)
                                n704 = Unbundle By Name(w2174) -> ("Position.x"=w2171:dbl, "Position.y"=w2167:dbl)
                                n705 = Unbundle By Name(w2176) -> ("Position.x"=w2168:dbl, "Position.y"=w2164:dbl)
                                n706 = local read "Area+ Buffer"() -> (w2155:dbl)
                                n707 = Subtract(x=w2171, y=w2155) -> (x-y=w2172:dbl)
                                n708 = Greater Or Equal?(x=w2168, y=w2172) -> (x >= y?=w2173:bool)
                                n709 = Add(x=w2167, y=w2155) -> (x+y=w2166:dbl)
                                n710 = Subtract(x=w2167, y=w2155) -> (x-y=w2165:dbl)
                                n711 = Add(x=w2171, y=w2155) -> (x+y=w2169:dbl)
                                n712 = Less Or Equal?(x=w2164, y=w2166) -> (x <= y?=w2163:bool)
                                n713 = Greater Or Equal?(x=w2164, y=w2165) -> (x >= y?=w2162:bool)
                                n714 = Less Or Equal?(x=w2168, y=w2169) -> (x <= y?=w2170:bool)
                                n715 = And(x=w2173, y=w2170) -> (x .and. y?=w2160:bool)
                                n716 = And(x=w2163, y=w2162) -> (x .and. y?=w2161:bool)
                                n717 = And(x=w2160, y=w2161) -> (x .and. y?=w2159:bool)
                                n718 = case shown="True" w2159 {
                                tunnel: w2158 -> [_ _]
                                tunnel: w2158 -> [_ w2178]
                                tunnel: w2156 -> [_ w2177]
                                frame False {
                                }
                                frame True {
                                n719 = stacked-sequence {
                                tunnel: w2178 -> [w2179 _]
                                tunnel: w2177 -> [w2180 _]
                                frame #0 {
                                n720 = local read "Potential Collisions"() -> (w2183:dbl)
                                n721 = local read "What to Check"() -> (w2184:dbl[])
                                n722 = Insert Into Array(array=w2184, index=w2183, new element=w2179) -> (w2185:dbl[])
                                n723 = local read "ID"() -> (w2182:dbl[])
                                n724 = Insert Into Array(array=w2182, index=w2183, new element=w2180) -> (w2181:dbl[])
                                n725 = local write "What to Check"(w2185) -> ()
                                n726 = local write "ID"(w2181) -> ()
                                }
                                frame #1 {
                                n727 = local read "Potential Collisions"() -> (w2188:dbl)
                                n728 = Add(x=w2188, y=1) -> (x+y=w2186:dbl)
                                n729 = local write "Potential Collisions"(w2186) -> ()
                                }
                                }
                                }
                                }
                                }
                                }
                                }
                                }
                                }
                                }
                                }
                              }
                            }
                          }
                        }
                        frame #1 {
                          n730 = local read "# of Spots"() -> (w2197:dbl)
                          n731 = Not Equal?(x=w2197, y=1) -> (x != y?=w2195:bool)
                          n732 = case shown="True" w2195 {
                            frame False {
                            }
                            frame True {
                              n733 = stacked-sequence {
                                frame #0 {
                                n734 = local read "Potential Collisions"() -> (w2200:dbl)
                                n735 = local read "Spot # Check"() -> (w2202:dbl)
                                n736 = Subtract(x=w2200, y=1) -> (x-y=w2198:dbl)
                                n737 = Less Or Equal?(x=w2202, y=w2198) -> (x <= y?=w2201:bool)
                                n738 = case shown="False" w2201 {
                                frame False {
                                n739 = local write "Spot # Check"(0) -> ()
                                }
                                frame True {
                                }
                                }
                                }
                                frame #1 {
                                n740 = local read "What to Check"() -> (w2208:dbl[])
                                n741 = local read "ID"() -> (w2206:dbl[])
                                n742 = local read "Spot # Check"() -> (w2204:dbl)
                                n743 = Index Array(array=w2208, index=w2204) -> (element=→"Value Check":dbl)
                                n744 = Index Array(array=w2206, index=w2204) -> (element=→"ID num check":dbl)
                                }
                              }
                            }
                          }
                        }
                      }
                    }
                  }
                  n745 = local read "Potential Collisions"() -> (w1985:dbl)
                  n746 = Subtract(x=w1985, y=1) -> (x-y=w1986:dbl)
                  n747 = local read "Hit"() -> (w2003:bool)
                  n748 = Equal?(x=w1998, y=w1986) -> (x = y?=w2002:bool)
                  n749 = Or(x=w2003, y=w2002) -> (x .or. y?=w2000:bool)
                }
                n750 = for {
                  tunnel: w1975 -> [w2222] mode=indexing
                  tunnel: w1976 -> [w2219] mode=indexing
                  tunnel: [w2221] -> w1970 mode=indexing
                  tunnel: w1972 -> [w2220]
                  # "If the projected distance is greater than the\nprevious distance, then the selected spots will move. \nThis situation only occurs if the bubble is about to/crossing \nthe buffer zone of another bubble. \n\nThe selected spots will also move if none of the bubbles\nare near/crossing the buffer zone of another bubble."
                  n751 = local read "Hit"() -> (w2212:bool)
                  n752 = Unbundle By Name(w2219) -> ()  [unwired: 1 out]
                  n753 = local read "Projected Distance"() -> (w2211:dbl)
                  n754 = Unbundle(w2222) -> ("Group ID"=→"Group ID #":i32, "Selected"=w2216:bool)
                  n755 = local read "Previous Distance"() -> (w2214:dbl)
                  n756 = Not(x=w2212) -> (.not. x?=w2210:bool)
                  n757 = Greater?(x=w2211, y=w2214) -> (0:w2213:bool)
                  n758 = And(x=w2212, y=w2213) -> (x .and. y?=w2209:bool)
                  n759 = Or(x=w2210, y=w2209) -> (x .or. y?=w2215:bool)
                  n760 = And(x=w2216, y=w2215) -> (x .and. y?=w2217:bool)
                  n761 = case shown="True" w2217 {
                    tunnel: w2219 -> [w2223 w2227]
                    tunnel: [w2223 w2226] -> w2221
                    tunnel: w2220 -> [_ w2228]
                    frame False {
                      # "otherwise, leave it alone!"
                    }
                    frame True {
                      # "If the spot is selected, move it by the same amount as the mouse"
                      n762 = call "extract_position.vi"("Spot"=w2227) -> ("Position"=w2225:cluster{"x":dbl, "y":dbl, "z":dbl})
                      n763 = Add(x=w2225, y=w2228) -> (x+y=w2224:cluster{dbl, dbl, dbl})
                      n764 = call "replace_position.vi"("Position"=w2224, "Spot in"=w2227) -> ("Spot"=w2226:T3)  [unwired: 2 out]
                    }
                  }
                }
                "Spot Checker" <- w1970
                n765 = local read "Locked Current Spot"() -> (w1966:dbl)
                n766 = Index Array(array=w1970, index=w1966) -> (element=w1969:T3)
                n767 = Unbundle By Name(w1969) -> ("Position.x"=→"New X":dbl, "Position.y"=→"New Y":dbl)  [unwired: 1 out]
                n768 = Array Size(array=w1970) -> (size(s)=→"# of Spots":i32)
              }
              frame True {
                # "coordinate conversion to find the rotation and scaling done by the mouse, about the centroid of the spots"
                n769 = Subtract(x=w2230, y=w2240) -> (x-y=w2249:cluster{dbl, dbl, dbl})
                n770 = Subtract(x=w2231, y=w2240) -> (x-y=w2248:cluster{dbl, dbl, dbl})
                n771 = Unbundle(w2248) -> (w2234:dbl, w2235:dbl)  [unwired: 1 out]
                n772 = Unbundle(w2249) -> (w2239:dbl, w2238:dbl)  [unwired: 1 out]
                n773 = Re/Im To Polar(2:w2235, 3:w2234) -> (0:w2232:dbl, 1:w2233:dbl)
                n774 = Re/Im To Polar(2:w2238, 3:w2239) -> (0:w2236:dbl, 1:w2237:dbl)
                n775 = Divide(x=w2233, y=w2237) -> (x/y=w2229:dbl)
                n776 = Subtract(x=w2232, y=w2236) -> (x-y=w2241:dbl)
                n777 = Bundle(w2229, w2229, w2229) -> (w2251:cluster{dbl, dbl, dbl})  [unwired: 1 out]
                n778 = call "scale_matrix.vi"("Scale Factors"=w2251) -> ("Scale Matrix"=w2247:T10)
                n779 = call "arb_rotation_matrix.vi"("Unit Vector"=cluster{dbl, dbl, dbl} {0.0, 0.0, 1.0}, "theta"=w2241) -> ("Real Matrix"=w2246:T10)
                n780 = call-poly <vilib>:"A x B.vi"("B"=w2246, "A"=w2247) -> ("A x B"=w2242:T10)  [unwired: 1 out]
                n781 = for {
                  tunnel: w2245 -> [w2257] mode=indexing
                  tunnel: [w2256] -> w2244 mode=indexing
                  tunnel: w2243 -> [w2255] mode=indexing
                  tunnel: w2240 -> [w2253]
                  tunnel: w2242 -> [w2252]
                  n782 = Unbundle(w2255) -> ("Selected"=w2254:bool)  [unwired: 1 out]
                  n783 = case shown="True" w2254 {
                    tunnel: w2257 -> [w2258 w2262]
                    tunnel: [w2258 w2261] -> w2256
                    tunnel: w2253 -> [_ w2260]
                    tunnel: w2252 -> [_ w2259]
                    frame False {
                    }
                    frame True {
                      n784 = call "apply_matrix_transformation_to_spots.vi"("Transform centre (i.e. transform about this point)"=w2260, "Transformation Matrix (3x3)"=w2259, "Spot In"=w2262) -> ("Spot Out"=w2261:T3)  [unwired: 5 out]
                    }
                  }
                }
              }
            }
          }
        }
        "Selection/Group" <- w1934
        n785 = Unbundle By Name(w1941) -> ("Position (Image Pixels)"=w1940:cluster{"X":dbl, "Y":dbl})
        n786 = Bundle By Name(cluster=w1941, "Dragging"=TRUE, "Previous Position (Image Pixels)"=w1940, "Position (Image Pixels)"=w1939) -> (w1950:T13)
      }
      event "stop": Value Change {
        n787 = event-data() -> ()  [unwired: 1 in, 4 out]
        n788 = global read "red_tweezers_globals_INTERNAL_VOLATILE.vi" "Current Settings File"() -> (w2266:path)
        n789 = call <vilib>:"Check if File or Folder Exists.vi"("path"=w2266) -> ("file or folder exists?"=w2265:bool)  [unwired: 8 in, 2 out]
        n790 = case shown="False" w2265 {
          tunnel: [w2273 w2277] -> w2267
          frame False {
            n791 = Two Button Dialog(message="Save current settings?", 1:"Don't Save" ("F button name (\"Cancel\")"), 2:"Save As..." ("T button name (\"OK\")")) -> (T button?=w2270:bool)
            n792 = Select(t=T18."Center Button" ("Which Button?"), s=w2270, f=T18."Right Button" ("Which Button?")) -> (s? t:f=w2273:T18)
          }
          frame True {
            n793 = call <vilib>:"Three Button Dialog.vi"("Allow user to close window? (TRUE)"=TRUE, "Window Title (\"\")"="Save Settings?" ("Window Title (\"\")"), "Right Button Text (\"Cancel\")"="No" ("Right Button Text (\"Cancel\")"), "Center Button Text (\"No\")"="Save As..." ("Center Button Text (\"No\")"), "Left Button Text (\"Yes\")"="Save" ("Left Button Text (\"Yes\")"), "message"="Would you like to save the current settings? You can choose to use the current settings file or save to a new location.") -> ("Which Button?"=w2277:T18)  [unwired: 5 in]
          }
        }
        n794 = case shown="\"Center Button\"" w2267 {
          tunnel: [TRUE TRUE FALSE FALSE] -> w2264
          frame "Left Button", Default {
          }
          frame "Center Button" {
            n795 = call "File Dialog5"("prompt"="Please select a location to save the settings", "button label"="Save", "default name"="red_tweezers_settings.xml", "pattern (all files)"="*.xml" ("pattern label"), "pattern label"="XML Settings Files") -> ("selected path"=w2285:path)  [unwired: 7 in, 3 out]
            n796 = global write "red_tweezers_globals_INTERNAL_VOLATILE.vi" "Current Settings File"(w2285) -> ()
          }
          frame "Right Button" {
          }
          frame "Window Close" {
          }
        }
        n797 = global write "red_tweezers_globals_INTERNAL_VOLATILE.vi" "Save Settings On Exit"(w2264) -> ()
      }
    }
    n798 = case shown="1" "ROI points" {
      frame 0, Default {
        # "ROI point 0 is not used"
        n799 = local read "ROI Y"() -> (w355:dbl)
        "ROI new Mpy" <- w355
        n800 = local read "ROI X"() -> (w356:dbl)
        "ROI new MPx" <- w356
        n801 = Build Array(w356, w355) -> (→"ROI Point 0":T10)
      }
      frame 1 {
        n802 = local read "Object MP Y"() -> (w362:dbl)
        n803 = local read "Object MP X"() -> (w363:dbl)
        n804 = local read "ROI Y"() -> (w359:dbl)
        "ROI y1" <- w359
        "NewY1" <- w359
        n805 = local read "ROI X"() -> (w358:dbl)
        "ROI x1" <- w358
        "NewX1" <- w358
        n806 = Subtract(x=w359, y=w362) -> (x-y=→"Radius ROI y1":dbl)
        n807 = Subtract(x=w358, y=w363) -> (x-y=→"Radius ROI x1":dbl)
        n808 = Build Array(w358, w359) -> (→"ROI Point 1":T10)
      }
      frame 2 {
        n809 = local read "Object MP Y"() -> (w369:dbl)
        n810 = local read "Object MP X"() -> (w370:dbl)
        n811 = local read "ROI Y"() -> (w366:dbl)
        "ROI y2" <- w366
        "NewY2" <- w366
        n812 = local read "ROI X"() -> (w365:dbl)
        "ROI x2" <- w365
        "NewX2" <- w365
        n813 = Subtract(x=w366, y=w369) -> (x-y=→"Radius ROI y2":dbl)
        n814 = Subtract(x=w365, y=w370) -> (x-y=→"Radius ROI x2":dbl)
        n815 = Build Array(w365, w366) -> (→"ROI Point 2":T10)
      }
      frame 3 {
        n816 = local read "Object MP Y"() -> (w376:dbl)
        n817 = local read "Object MP X"() -> (w377:dbl)
        n818 = local read "ROI Y"() -> (w372:dbl)
        "ROI y3" <- w372
        n819 = local read "ROI X"() -> (w373:dbl)
        "ROI x3" <- w373
        n820 = Subtract(x=w372, y=w376) -> (x-y=→"Radius ROI y3":dbl)
        n821 = Subtract(x=w373, y=w377) -> (x-y=→"Radius ROI x3":dbl)
        n822 = Build Array(w373, w372) -> (→"ROI Point 3":T10)
      }
      frame 4 {
        n823 = local read "Object MP Y"() -> (w384:dbl)
        n824 = local read "Object MP X"() -> (w383:dbl)
        n825 = local read "ROI Y"() -> (w379:dbl)
        "ROI y4" <- w379
        n826 = local read "ROI X"() -> (w380:dbl)
        "ROI x4" <- w380
        n827 = Subtract(x=w379, y=w384) -> (x-y=→"Radius ROI y4":dbl)
        n828 = Subtract(x=w380, y=w383) -> (x-y=→"Radius ROI x4":dbl)
        n829 = Build Array(w380, w379) -> (→"ROI Point 4":T10)
      }
      frame 5 {
        n830 = local read "Object MP Y"() -> (w391:dbl)
        n831 = local read "Object MP X"() -> (w390:dbl)
        n832 = local read "ROI Y"() -> (w387:dbl)
        "ROI y5" <- w387
        n833 = local read "ROI X"() -> (w386:dbl)
        "ROI x5" <- w386
        n834 = Subtract(x=w387, y=w391) -> (x-y=→"Radius ROI y5":dbl)
        n835 = Subtract(x=w386, y=w390) -> (x-y=→"Radius ROI x5":dbl)
        n836 = Build Array(w386, w387) -> (→"ROI point 5":T10)
      }
      frame 6 {
        n837 = local read "Object MP Y"() -> (w398:dbl)
        n838 = local read "Object MP X"() -> (w397:dbl)
        n839 = local read "ROI Y"() -> (w393:dbl)
        "ROI y6" <- w393
        n840 = local read "ROI X"() -> (w394:dbl)
        "ROI x6" <- w394
        n841 = Subtract(x=w393, y=w398) -> (x-y=→"Radius ROI y6":dbl)
        n842 = Subtract(x=w394, y=w397) -> (x-y=→"Radius ROI x6":dbl)
        n843 = Build Array(w394, w393) -> (→"ROI Point 6":T10)
      }
      frame 7 {
      }
    }
    n844 = case shown="True" "Camera Capture 2" {
      frame False {
      }
      frame True {
        n845 = local read "Circles 2"() -> (w473:T2)
        n846 = Index Array(array=w473) -> (element=w474:T27)  [unwired: 1 in]
        n847 = Index Array(array=w473) -> (element=w484:T27)  [unwired: 1 in]
        n848 = Unbundle(w474) -> ("Position"=w482:cluster{"X":sgl, "Y":sgl}, "Radius"=w475:dbl)  [unwired: 1 out]
        n849 = Unbundle(w484) -> ("Position"=w483:cluster{"X":sgl, "Y":sgl})  [unwired: 2 out]
        n850 = Unbundle(w482) -> ("X"=w480:sgl, "Y"=w481:sgl)
        n851 = Unbundle(w483) -> ("X"=→"Bubble x 2":sgl, "Y"=→"Bubble y 2":sgl)
        n852 = Subtract(x=w480, y=w475) -> (x-y=→"toplx 3":dbl)
        n853 = Add(x=w480, y=w475) -> (x+y=→"bottomrx 3":dbl)
        n854 = Add(x=w481, y=w475) -> (x+y=→"bottomry 3":dbl)
        n855 = Subtract(x=w481, y=w475) -> (x-y=→"toply 3":dbl)
      }
    }
    n856 = property on="Image" class="ImageControl"() -> ("ROI"=w48:T28)  [unwired: 2 in, 2 out]
    n857 = Unbundle By Name(w48) -> ("Contours"=w44:T29)
    n858 = Index Array(array=w44) -> (element=w45:T30)  [unwired: 1 in]
    n859 = Unbundle By Name(w45) -> ("Points"=w46:i32[])
    n860 = Index Array(array=w46, index #1=0 ("index")) -> (element #1=→"Numeric 3":i32, element #2=→"Numeric 2":i32)  [unwired: 1 in]
    n861 = call "Vision Acquisition"() -> ("Image Out"=w32:T11)  [unwired: 24 in, 3 out]
    n862 = call-poly "IMAQ Detect Shapes"("Circle Descriptor"="Circle Descriptor 2", "Image"=w32) -> ("Number of Matches Returned"=→"Number of Matches Returned":i32, "Circles"=→"Circles 2":T2)  [unwired: 7 in, 1 out]
    n863 = call "IMAQ Create"("Image Name"="untitled", "Image Type"=w74) -> ("New Image"=w73:T11)  [unwired: 3 in, 1 out]
    n864 = call "IMAQ ExtractSingleColorPlane"("Color Plane"=w72, "Image Dst"=w73, "Image Src"=w32) -> ()  [unwired: 7 in, 2 out]
    n865 = case shown="True" "ROI switch" {
      tunnel: w32 -> [w401 w441]
      frame False {
        n866 = local read "Number of Matches Returned"() -> (w400:dbl)
        n867 = Add(x=w400, y=1.0 ("x+y")) -> (x+y=w402:dbl)
        n868 = for {
          N: w402 -> [_]
          tunnel: w401 -> [w410]
          i -> [w436]
          w408 = 1e-07  # y
          w409 = 1e-07  # y
          n869 = property on="Camera 3" class="ImageControl"() -> ("ROI"=w411:T28)  [unwired: 2 in, 2 out]
          n870 = Unbundle By Name(w411) -> ("Contours"=w420:T29)
          n871 = local read "Circles 2"() -> (w423:T2)
          n872 = Number To Decimal String(number=w436) -> (decimal integer string=w435:string)  [unwired: 1 in]
          n873 = Index Array(array=w423) -> (element=w440:T27)  [unwired: 1 in]
          n874 = Index Array(array=w420) -> (element=w419:T30)  [unwired: 1 in]
          n875 = Unbundle(w440) -> ("Position"=w434:cluster{"X":sgl, "Y":sgl}, "Radius"=w422:dbl)  [unwired: 1 out]
          "Radius" <- w422
          n876 = Unbundle By Name(w419) -> ("Points"=w418:i32[])
          n877 = Unbundle(w434) -> ("X"=w438:sgl, "Y"=w437:sgl)
          n878 = Subtract(x=w438, y=w422) -> (x-y=→"toplx 2":dbl)
          n879 = Add(x=w438, y=w422) -> (x+y=→"bottomrx 2":dbl)
          n880 = Add(x=w437, y=w422) -> (x+y=→"bottomry 2":dbl)
          n881 = Subtract(x=w437, y=w422) -> (x-y=→"toply 2":dbl)
          n882 = Index Array(array=w418, index #1=0 ("index"), index #2=1 ("index")) -> (element #1=w407:i32, element #2=w405:i32)
          n883 = Bundle(w407, w405) -> (w415:cluster{i32, i32})  [unwired: 1 in]
          "Specific Point 2" <- w415
          n884 = call "IMAQ Overlay Text"("Text Color (black)"=u32 1703680, "Font, Size & Style"=T14 {"Desired Font (Application)"=enum."Application Font", "[User-specified Font]"={"Font Name"="", "Size"=40, "Strikeout?"=FALSE, "Italic?"=FALSE, "Underline?"=FALSE, "Outline?"=FALSE, "Shadow?"=FALSE, "Bold?"=FALSE, "Rotation Angle"=0.0}, "Horizontal Alignment"=0, "Vertical Alignment"=0}, "String"="ROI", "Origin"=w415, "Image"=w410) -> ()  [unwired: 5 in, 2 out]
          n885 = Multiply(x=w407, y=w408) -> (x*y=w406:dbl)
          n886 = Multiply(x=w405, y=w409) -> (x*y=w404:dbl)
          n887 = local read "toply 2"() -> (w426:dbl)
          n888 = local read "bottomrx 2"() -> (w425:dbl)
          n889 = local read "toplx 2"() -> (w427:dbl)
          n890 = local read "bottomry 2"() -> (w424:dbl)
          n891 = local write "ROI X"(w406) -> ()
          n892 = local write "ROI Y"(w404) -> ()
          n893 = Build Array(w427, w426, w425, w424) -> (w432:dbl[])
          n894 = Array To Cluster(array=w432) -> (cluster=w439:T31)
          n895 = call "IMAQ Overlay Oval"("Bounding Rectangle"=w439, "Image"=w410) -> ("Image Out"=w433:T11)  [unwired: 8 in, 1 out]
          n896 = call "IMAQ Overlay Text"("String"=w435, "Origin"=w434, "Image"=w433) -> ("Image Out"=→"Camera 3":T11)  [unwired: 7 in, 1 out]
        }
      }
      frame True {
        # "This is the code for ROI and Object detection"
        n897 = local read "Number of Objects"() -> (w443:i32)
        n898 = Add(x=w443, y=1.0 ("x+y")) -> (x+y=w442:dbl)
        n899 = for {
          N: w442 -> [_]
          tunnel: w441 -> [w458]
          w449 = 1e-07  # y
          w450 = 1e-07  # y
          # "This part of the\ncode detects \nobeject"
          # "This is the ROI, a specific point selected"
          # "This part of the code will obtain the Midpoint"
          n900 = property on="Camera 3" class="ImageControl"() -> ("ROI"=w457:T28)  [unwired: 2 in, 2 out]
          n901 = local read "Objects"() -> (w454:T1)
          n902 = Unbundle By Name(w457) -> ("Contours"=w467:T29)
          n903 = Index Array(array=w454) -> (element=w455:T32)  [unwired: 1 in]
          n904 = call "IMAQ Count Objects 2"("Settings"="Settings", "Image"=w458) -> ("Number of Objects"=→"Number of Objects":i32, "Image Out"=w470:T11, "Objects"=→"Objects":T1)  [unwired: 5 in, 2 out]
          n905 = local write "Camera 3"(w470) -> ()
          n906 = Index Array(array=w467) -> (element=w466:T30)  [unwired: 1 in]
          n907 = Unbundle(w455) -> ("Object Center"=w453:cluster{"X":sgl, "Y":sgl})  [unwired: 5 out]
          n908 = Unbundle By Name(w466) -> ("Points"=w465:i32[])
          n909 = Unbundle(w453) -> ("X"=→"Object MP X":sgl, "Y"=→"Object MP Y":sgl)
          n910 = Index Array(array=w465, index #1=0 ("index"), index #2=1 ("index")) -> (element #1=w446:i32, element #2=w448:i32)
          n911 = Multiply(x=w446, y=w450) -> (x*y=→"ROI X":dbl)
          n912 = Multiply(x=w448, y=w449) -> (x*y=→"ROI Y":dbl)
          n913 = Bundle(w446, w448) -> (w462:cluster{i32, i32})  [unwired: 1 in]
          "Specific Point" <- w462
          n914 = call "IMAQ Overlay Text"("Text Color (black)"=u32 1703680, "Font, Size & Style"=T14 {"Desired Font (Application)"=enum."Application Font", "[User-specified Font]"={"Font Name"="", "Size"=40, "Strikeout?"=FALSE, "Italic?"=FALSE, "Underline?"=FALSE, "Outline?"=FALSE, "Shadow?"=FALSE, "Bold?"=FALSE, "Rotation Angle"=0.0}, "Horizontal Alignment"=0, "Vertical Alignment"=0}, "String"="ROI", "Origin"=w462, "Image"=w458) -> ()  [unwired: 5 in, 2 out]
        }
      }
    }
    n915 = case shown="True" "Play" {
      frame False {
      }
      frame True {
        n916 = stacked-sequence {
          frame #0 {
            n917 = Tick Count (ms)() -> (millisecond timer value=→"Start":u32)
          }
          frame #1 {
            n918 = local read "ROI switch"() -> (w645:bool)
            n919 = case shown="False" w645 {
              frame True {
                # "When this is on select a new Midpoint using the ROI tool"
                n920 = case shown="True" "New location\n ROI" {
                  frame False {
                    n921 = local read "ROI Point 2"() -> (w656:T10)
                    n922 = local read "ROI Point 1"() -> (w657:T10)
                    n923 = local read "ROI Point 3"() -> (w655:T10)
                    n924 = local read "ROI Point 4"() -> (w654:T10)
                    n925 = local read "ROI point 5"() -> (w653:T10)
                    n926 = local read "ROI Point 6"() -> (w652:T10)
                    n927 = Build Array (concatenate) ("Build Matrix")(w657, w656, w655, w654, w653, w652) -> (w658:T10)
                    n928 = local write "NewXYArray"(w658) -> ()
                  }
                  frame True {
                    w695 = 1e-07
                    n929 = local read "Radius ROI x1"() -> (w697:dbl)
                    n930 = local read "Radius ROI x3"() -> (w678:dbl)
                    n931 = local read "Radius ROI x4"() -> (w676:dbl)
                    n932 = local read "Radius ROI y1"() -> (w696:dbl)
                    n933 = local read "Radius ROI y2"() -> (w679:dbl)
                    n934 = local read "Radius ROI y3"() -> (w677:dbl)
                    n935 = local read "Radius ROI y4"() -> (w675:dbl)
                    n936 = local read "Radius ROI y5"() -> (w673:dbl)
                    n937 = local read "Radius ROI y6"() -> (w671:dbl)
                    n938 = local read "Radius ROI x2"() -> (w680:dbl)
                    n939 = local read "Radius ROI x5"() -> (w674:dbl)
                    n940 = local read "Radius ROI x6"() -> (w672:dbl)
                    n941 = local read "ROI new MPx"() -> (w682:dbl)
                    n942 = local read "ROI new Mpy"() -> (w681:dbl)
                    n943 = Add(x=w697, y=w682) -> (x+y=w670:dbl)
                    n944 = Add(x=w696, y=w681) -> (x+y=w669:dbl)
                    n945 = Add(x=w682, y=w680) -> (x+y=w668:dbl)
                    n946 = Add(x=w681, y=w679) -> (x+y=w667:dbl)
                    n947 = Add(x=w682, y=w678) -> (x+y=w666:dbl)
                    n948 = Add(x=w681, y=w677) -> (x+y=w665:dbl)
                    n949 = Add(x=w682, y=w676) -> (x+y=w664:dbl)
                    n950 = Add(x=w681, y=w675) -> (x+y=w663:dbl)
                    n951 = Add(x=w682, y=w674) -> (x+y=w662:dbl)
                    n952 = Add(x=w673, y=w681) -> (x+y=w661:dbl)
                    n953 = Add(x=w682, y=w672) -> (x+y=w660:dbl)
                    n954 = Add(x=w671, y=w681) -> (x+y=w659:dbl)
                    n955 = Build Array(w670, w669) -> (w694:T10)
                    n956 = Build Array(w668, w667) -> (w691:T10)
                    n957 = Build Array(w666, w665) -> (w690:T10)
                    n958 = Build Array(w664, w663) -> (w689:T10)
                    n959 = Build Array(w662, w661) -> (w688:T10)
                    n960 = Build Array(w660, w659) -> (w687:T10)
                    n961 = call-poly <vilib>:"Multiply.vi"("Real Scalar c"=w695, "Real Matrix A"=w694) -> ("A * c"=w693:T10)
                    n962 = call-poly <vilib>:"Multiply.vi"("Real Scalar c"=w695, "Real Matrix A"=w691) -> ("A * c"=w692:T10)
                    n963 = call-poly <vilib>:"Multiply.vi"("Real Scalar c"=w695, "Real Matrix A"=w690) -> ("A * c"=w686:T10)
                    n964 = call-poly <vilib>:"Multiply.vi"("Real Scalar c"=w695, "Real Matrix A"=w689) -> ("A * c"=w685:T10)
                    n965 = call-poly <vilib>:"Multiply.vi"("Real Scalar c"=w695, "Real Matrix A"=w688) -> ("A * c"=w684:T10)
                    n966 = call-poly <vilib>:"Multiply.vi"("Real Scalar c"=w695, "Real Matrix A"=w687) -> ("A * c"=w683:T10)
                    n967 = Build Array (concatenate) ("Build Matrix")(w693, w692, w686, w685, w684, w683) -> (w698:T10)
                    n968 = local write "NewXYArray"(w698) -> ()
                  }
                }
              }
              frame False {
                n969 = case shown="True" "Input New \nObject Location" {
                  frame True {
                    n970 = local read "Caging Radius"() -> (w702:dbl)
                    n971 = Multiply(x=w702, y=1e-07) -> (x*y=w700:dbl)
                    n972 = local read "Radius"() -> (w704:dbl)
                    n973 = local read "New Center X"() -> (w716:dbl)
                    n974 = Add(x=w704, y=w700) -> (x+y=w703:dbl)
                    n975 = local read "New Center Y"() -> (w720:dbl)
                    n976 = local read "# of pairs"() -> (w719:dbl)
                    n977 = Add(x=w716, y=w703) -> (x+y=w722:dbl)
                    n978 = Multiply(x=w722, y=1e-07) -> (x*y=w715:dbl)
                    n979 = Multiply(x=w719, y=2.0) -> (x*y=w717:dbl)
                    n980 = Multiply(x=w720, y=1e-07) -> (x*y=w714:dbl)
                    n981 = Initialize Array(w715, w717) -> (w713:dbl[])
                    n982 = local read "Delta y"() -> (w711:dbl[])
                    n983 = local read "Delta x"() -> (w712:dbl[])
                    n984 = Initialize Array(w714, w717) -> (w710:dbl[])
                    n985 = for {
                      tunnel: w711 -> [w731] mode=indexing
                      tunnel: w710 -> [w730] mode=indexing
                      tunnel: [w729] -> w707 mode=indexing
                      n986 = Add(x=w730, y=w731) -> (x+y=w729:dbl)
                    }
                    n987 = for {
                      tunnel: w713 -> [w728] mode=indexing
                      tunnel: w712 -> [w727] mode=indexing
                      tunnel: [w726] -> w709 mode=indexing
                      n988 = Subtract(x=w728, y=w727) -> (x-y=w726:dbl)
                    }
                    n989 = for {
                      tunnel: w710 -> [w734] mode=indexing
                      tunnel: w711 -> [w733] mode=indexing
                      tunnel: [w732] -> w708 mode=indexing
                      n990 = Subtract(x=w734, y=w733) -> (x-y=w732:dbl)
                    }
                    n991 = Build Array(w709, w707) -> (w706:T10)
                    n992 = Build Array(w709, w708) -> (w705:T10)
                    n993 = Build Array(w715, w714) -> (w725:T10)
                    n994 = Build Array (concatenate)(w725, w706, w705) -> (w724:T10)
                    n995 = local write "NewXYArray"(w724) -> ()
                  }
                  frame False {
                    n996 = local read "Center X"() -> (w736:dbl)
                    n997 = Multiply(x=w736, y=1e-07) -> ()  [unwired: 1 out]
                  }
                }
              }
            }
            n998 = local write "Max Number \nof Bubbles"("Max Number \nof Bubbles") -> ()
            n999 = local write "LCS"("LCS") -> ()
            n1000 = local write "Rates"("Rates") -> ()
            n1001 = local write "How Many Frames?"("Number of Planned\nSequence Frames") -> ()
            "Initiate Creation" <- 1.0
          }
          frame #2 {
            n1002 = local read "NewXYArray"() -> (w740:dbl[][])
            n1003 = Array Size(array=w740) -> (size(s)=w739:i32[])
            n1004 = Index Array(array=w739, index=0) -> (element=w737:i32)
            "NewXYArraySize" <- w737
            n1005 = for {
              N: w737 -> [w742]
              i -> [w743]
              stop <- w741 stop-if-true
              n1006 = stacked-sequence {
                tunnel: w743 -> [w745 _]
                tunnel: w742 -> [w744 _]
                tunnel: [_ w748] -> w741
                frame #0 {
                  n1007 = local write "Locked Current Spot"(w745) -> ()
                  n1008 = local write "# of Spots"(w744) -> ()
                  n1009 = local write "Rates"(1) -> ()
                  n1010 = local write "LCS"(0) -> ()
                }
                frame #1 {
                  n1011 = local read "Insert"() -> (w748:bool)
                  n1012 = local write "Insert"(TRUE) -> ()
                }
              }
            }
          }
        }
      }
    }
    n1013 = local read "bottomrx 2"() -> (w64:dbl)
    n1014 = local read "toplx 2"() -> (w63:dbl)
    n1015 = local read "bottomry 2"() -> (w62:dbl)
    n1016 = local read "toply 2"() -> (w61:dbl)
    n1017 = Subtract(x=w62, y=w61) -> (x-y=w60:dbl)
    n1018 = Subtract(x=w63, y=w64) -> (x-y=w66:dbl)
    n1019 = Absolute Value(x=w60) -> (abs(x)=w59:dbl)
    n1020 = local read "toplx 2"() -> (w68:dbl)
    n1021 = local write "Caging Radius"("Caging Radius") -> ()
    n1022 = local read "toply 2"() -> (w57:dbl)
    n1023 = Absolute Value(x=w66) -> (abs(x)=w67:dbl)
    n1024 = Divide(x=w59, y=2.0) -> (x/y=w54:dbl)
    n1025 = Divide(x=w67, y=2.0) -> (x/y=w55:dbl)
    n1026 = Add(x=w54, y=w57) -> (x+y=→"Center Y":dbl)
    n1027 = Add(x=w55, y=w68) -> (x+y=→"Center X":dbl)
    n1028 = local read "Stop"() -> (w77:i32)
    n1029 = local read "Start"() -> (w76:i32)
    n1030 = local write "New Center X"("New Center X") -> ()
    n1031 = local write "New Center Y"("New Center Y") -> ()
    n1032 = Subtract(x=w77, y=w76) -> (x-y=→"Time Elapsed(ms)":i32)
    n1033 = case shown="True" "Lock Current Spot" {
      frame False {
      }
      frame True {
        n1034 = global read "red_tweezers_globals.vi" "Spots"() -> (w827:T3[])
        n1035 = local read "Current Spot #"() -> (w828:dbl)
        "Locked Current Spot" <- w828
        n1036 = Index Array(array=w827, index=w828) -> (element=w829:T3)
        n1037 = Unbundle By Name(w829) -> ("Position.x"=→"LCS X":dbl, "Position.y"=→"LCS Y":dbl)
        n1038 = local write "LCS"(0) -> ()
      }
    }
    n1039 = Not Equal?(x=1, y=1) -> (x != y?=w33:bool)
    n1040 = case shown="True" w33 {
      frame False {
      }
      frame True {
        # "array of bubbles"
        n1041 = local read "Max Number \nof Bubbles"() -> (w190:dbl)
        n1042 = local read "bottomry 2"() -> (w211:dbl)
        n1043 = local read "toply 2"() -> (w212:dbl)
        n1044 = Subtract(x=w212, y=w211) -> (x-y=w213:dbl)
        n1045 = local read "Caging Radius"() -> (w191:dbl)
        n1046 = local read "bottomrx 2"() -> (w206:dbl)
        n1047 = local read "bottomry 2"() -> (w205:dbl)
        n1048 = case shown="Default" w190 {
          tunnel: [1 2 3 4 5 6 0] -> w195
          frame 3 {
          }
          frame 4, 5 {
          }
          frame 6, 7 {
          }
          frame 8, 9 {
          }
          frame 10, 11 {
          }
          frame 12 {
          }
          frame Default {
          }
        }
        "# of pairs" <- w195
        n1049 = local read "Radius"() -> (w198:dbl)
        n1050 = Divide(x=w213, y=2.0) -> (x/y=w204:dbl)
        n1051 = Add(x=w205, y=w204) -> (x+y=w207:dbl)
        n1052 = Multiply(x=w206, y=1e-07) -> (x*y=w193:dbl)
        n1053 = Multiply(x=w198, y=1e-07) -> (x*y=w186:dbl)
        n1054 = Multiply(x=w191, y=1e-07) -> (x*y=w189:dbl)
        n1055 = Multiply(x=w207, y=1e-07) -> (x*y=w203:dbl)
        n1056 = Add(x=w186, y=w189) -> (x+y=w194:dbl)
        n1057 = Add(x=w189, y=w193) -> (x+y=w192:dbl)
        n1058 = for {
          N: w195 -> [_]
          tunnel: w190 -> [w231]
          tunnel: w194 -> [w230]
          tunnel: w203 -> [w229]
          tunnel: [w228] -> w202 mode=indexing
          tunnel: [w227] -> w201 mode=indexing
          tunnel: [w226] -> w200 mode=indexing
          tunnel: [w224] -> w197 mode=indexing
          tunnel: [w223] -> w196 mode=indexing
          tunnel: w192 -> [w222]
          tunnel: [w221] -> w188 mode=indexing
          i -> [w225]
          w240 = 2.0
          n1059 = Divide(x=360, y=w231) -> (x/y=w246:dbl)
          n1060 = Add(x=1, y=w225) -> (x+y=w244:i32)
          n1061 = Multiply(x=w246, y=w244) -> (x*y=w239:dbl)
          n1062 = expression code="(x/180.0)*pi" ("degrees to radians")(w239) -> (w238:dbl)
          n1063 = Subtract(x=180, y=w239) -> (x-y=w247:dbl)
          n1064 = Square(x=w230) -> (x^2=w242:dbl)
          n1065 = Cosine(x=w238) -> (cos(x)=w237:dbl)
          n1066 = Divide(x=w247, y=w240) -> (x/y=w235:dbl)
          n1067 = Multiply(x=w240, y=w242) -> (x*y=w243:dbl)
          n1068 = Compound Arithmetic op=MULTIPLY(w240, w237, w242) -> (w241:dbl)
          n1069 = expression code="(x/180.0)*pi" ("degrees to radians")(w235) -> (w236:dbl)
          n1070 = Subtract(x=w243, y=w241) -> (x-y=w233:dbl)
          n1071 = Sine(x=w236) -> (sin(x)=w232:dbl)
          n1072 = Cosine(x=w236) -> (cos(x)=w234:dbl)
          n1073 = Square Root(x=w233) -> (sqrt(x)=w221:dbl)
          n1074 = Multiply(x=w232, y=w221) -> (x*y=w224:dbl)
          n1075 = Multiply(x=w234, y=w221) -> (x*y=w223:dbl)
          n1076 = Add(x=w229, y=w224) -> (x+y=w227:dbl)
          n1077 = Subtract(x=w229, y=w224) -> (x-y=w228:dbl)
          n1078 = Subtract(x=w222, y=w223) -> (x-y=w226:dbl)
        }
        "Delta y" <- w197
        "Delta x" <- w196
        n1079 = Index Array(array=w188, index=0) -> (element=w187:dbl)
        n1080 = Build Array(w200, w201) -> (w209:T10)
        n1081 = Greater Or Equal?(x=w187, y=w186) -> (x >= y?=→"Caging Radius \nToo Big":bool)
        n1082 = Build Array(w192, w203) -> (w210:T10)
        n1083 = Build Array(w200, w202) -> (w208:T10)
        n1084 = Build Array (concatenate) ("Build Matrix")(w210, w209, w208) -> (→"NewXYArray":T10)
      }
    }
    n1085 = case shown="True" "Mark Original Position" {
      frame False {
      }
      frame True {
        w830 = TRUE
        n1086 = local write "Mark Original Position"(FALSE) -> ()
        n1087 = local read "New X"() -> (→"Original X":dbl)
        n1088 = local read "New Y"() -> (→"Original Y":dbl)
        "MOP pressed After" <- w830
        "MOP pressed" <- w830
      }
    }
    n1089 = case shown="True" "Add Additional Frames" {
      frame False {
      }
      frame True {
        # "This adds additional frames to the sequence."
        n1090 = for {
          N: "Additional Frames Wanted" -> [_]
          i -> [w836]
          n1091 = local read "Max Number \nof Bubbles"() -> (w840:dbl)
          n1092 = Add(x=1, y=w836) -> (x+y=w837:i32)
          n1093 = Add(x="Frame Location", y=w837) -> (x+y=w838:dbl)
          n1094 = Initialize Array(T15 {"Position"={"x"=nan, "y"=nan, "z"=nan}, "Intensity"=1.0, "Vortex Charge"=1, "Phase"=1.0, "NA Position"={"x"=0.0, "y"=0.0, "r"=1.0}, "Line Trapping"={"Vector"={"x"=0.0, "y"=0.0, "z"=0.0}, "Phase Gradient"=0.0}, "Amplitude Correction"=0.0} ("Cluster"), w840) -> (w841:T33)
          n1095 = local read "Sequence Storer"() -> (w842:T3[][])
          n1096 = Insert Into Array(array=w842, index (row)=w838, new element=w841) -> (w843:T3[][])  [unwired: 1 in]
          n1097 = local write "Sequence Storer"(w843) -> ()
        }
      }
    }
    n1098 = local read "Rates"() -> (w81:dbl)
    n1099 = Equal?(x=w81, y=1.0) -> (x = y?=w79:bool)
    n1100 = case shown="True" w79 {
      frame False {
      }
      frame True {
        n1101 = stacked-sequence {
          frame #0 {
            n1102 = local read "Number of Planned\nSequence Frames"() -> (w566:dbl)
            n1103 = local read "Tab Control"() -> (w567:enum32{"Line", "Arc"})
            n1104 = case shown="\"Arc\"" w567 {
              tunnel: w566 -> [w601 w614]
              frame "Arc" {
                w590 = 2
                w595 = 1e-07
                n1105 = local read "Current X"() -> (w584:dbl)
                n1106 = local read "Center X"() -> (w583:dbl)
                n1107 = local read "Center Y"() -> (w581:dbl)
                n1108 = local read "Current Y"() -> (w582:dbl)
                n1109 = expression code="(x/180.0)*pi"(180.0) -> (w599:dbl)
                n1110 = Subtract(x=w601, y=1.0) -> (x-y=w598:dbl)
                n1111 = Subtract(x=w584, y=w583) -> (x-y=w579:dbl)
                "Original D-X" <- w579
                n1112 = Subtract(x=w582, y=w581) -> (x-y=w580:dbl)
                "Original D-Y" <- w580
                n1113 = Divide(x=w599, y=w598) -> (x/y=→"Degree Rate":dbl)
                n1114 = Divide(x=w580, y=w579) -> (x/y=w578:dbl)
                n1115 = Greater Or Equal To 0?(x=w580) -> (x >= 0?=w575:bool)
                n1116 = Greater Or Equal To 0?(x=w579) -> (x >= 0?=w576:bool)
                n1117 = Inverse Tangent(1:w578) -> (0:w577:dbl)
                n1118 = local read "ROI X"() -> (w596:dbl)
                "ROI X" <- w596
                n1119 = local read "ROI Y"() -> (w594:dbl)
                "ROI Y" <- w594
                n1120 = case shown="True" w576 {
                  tunnel: w577 -> [w605 w607]
                  tunnel: w575 -> [_ w608]
                  tunnel: [w603 w606] -> w574
                  frame False {
                    n1121 = Add(x=w605, y=3.141592653589793) -> (x+y=w603:dbl)
                  }
                  frame True {
                    n1122 = case shown="False" w608 {
                      tunnel: w607 -> [w610 w612]
                      tunnel: [w611 w612] -> w606
                      frame False {
                        n1123 = Add(x=w610, y=6.283185307179586) -> (x+y=w611:dbl)
                      }
                      frame True {
                      }
                    }
                  }
                }
                "Original Theta" <- w574
                n1124 = Multiply(x=w596, y=w595) -> (x*y=w592:dbl)
                n1125 = Multiply(x=w595, y=w594) -> (x*y=w591:dbl)
                n1126 = Divide(x=w592, y=w590) -> (x/y=w589:dbl)
                "Center X" <- w589
                n1127 = Divide(x=w591, y=w590) -> (x/y=w588:dbl)
                "Center Y" <- w588
                n1128 = Build Array(w589, w588) -> (→"Center Location":T10)
                n1129 = local read "Position"() -> (w593:cluster{"x":dbl, "y":dbl, "z":dbl})
                n1130 = Unbundle(w593) -> ("x"=→"Current X":dbl, "y"=→"Current Y":dbl)  [unwired: 1 out]
                n1131 = local read "Original D-X"() -> (w572:dbl)
                n1132 = local read "Original D-Y"() -> (w573:dbl)
                n1133 = Square(x=w573) -> (x^2=w570:dbl)
                n1134 = Square(x=w572) -> (x^2=w571:dbl)
                n1135 = Add(x=w571, y=w570) -> (x+y=w568:dbl)
                n1136 = Square Root(x=w568) -> (sqrt(x)=→"Original Radius":dbl)
              }
              frame "Line" {
                n1137 = local read "Max Number \nof Bubbles"() -> (w613:dbl)
                n1138 = for {
                  N: w613 -> [_]
                  tunnel: w614 -> [w616]
                  i -> [w615]
                  n1139 = stacked-sequence {
                    tunnel: w616 -> [_ w634]
                    tunnel: w615 -> [w620 w631]
                    frame #0 {
                      n1140 = local read "NewXYArray"() -> (w626:dbl[][])
                      n1141 = Index Array(array=w626, index (row)=w620) -> (element=w625:dbl[])  [unwired: 1 in]
                      n1142 = Array To Cluster(array=w625) -> (cluster=w624:T34)
                      n1143 = global read "red_tweezers_globals.vi" "Spots"() -> (w621:T3[])
                      n1144 = Unbundle By Name(w624) -> ("NewXYArray[0]"=w623:dbl, "NewXYArray[1]"=w622:dbl)
                      n1145 = Index Array(array=w621, index=w620) -> (element=w619:T3)
                      n1146 = local write "New Y"(w622) -> ()
                      n1147 = local write "New X"(w623) -> ()
                      n1148 = Unbundle By Name(w619) -> ("Position.x"=w618:dbl, "Position.y"=w617:dbl)
                      n1149 = local write "Original X"(w618) -> ()
                      n1150 = local write "Original Y"(w617) -> ()
                    }
                    frame #1 {
                      n1151 = local read "Original X"() -> (w635:dbl)
                      n1152 = local read "Original Y"() -> (w637:dbl)
                      n1153 = Subtract(x=w634, y=1) -> (x-y=w641:dbl)
                      n1154 = local read "New Y"() -> (w638:dbl)
                      n1155 = local read "New X"() -> (w636:dbl)
                      n1156 = Subtract(x=w637, y=w638) -> (x-y=w640:dbl)
                      n1157 = Subtract(x=w635, y=w636) -> (x-y=w639:dbl)
                      n1158 = Divide(x=w640, y=w641) -> (x/y=w629:dbl)
                      "Y Rate" <- w629
                      n1159 = Divide(x=w639, y=w641) -> (x/y=w630:dbl)
                      "X Rate" <- w630
                      n1160 = Bundle(w630, w629) -> (w628:cluster{dbl, dbl})  [unwired: 1 in]
                      n1161 = local read "NewXYRates"() -> (w632:dbl[][])
                      n1162 = Cluster To Array(cluster=w628) -> (array=w627:dbl[])
                      n1163 = Insert Into Array(array=w632, index (row)=w631, new element=w627) -> (w633:dbl[][])  [unwired: 1 in]
                      n1164 = local write "NewXYRates"(w633) -> ()
                    }
                  }
                }
              }
            }
          }
          frame #1 {
            n1165 = local write "Rates"(0) -> ()
          }
        }
      }
    }
    n1166 = local read "Initiate Creation"() -> (w84:dbl)
    n1167 = case shown="1" w84 {
      frame 0, Default {
      }
      frame 1 {
        # "This create the array needed for a sequential\narray."
        n1168 = local read "Number of Planned\nSequence Frames"() -> (w847:dbl)
        n1169 = local read "Max Number \nof Bubbles"() -> (w846:dbl)
        n1170 = for {
          N: w847 -> [_]
          tunnel: w846 -> [w848]
          i -> [w851]
          n1171 = Initialize Array(T15 {"Position"={"x"=nan, "y"=nan, "z"=nan}, "Intensity"=1.0, "Vortex Charge"=1, "Phase"=1.0, "NA Position"={"x"=0.0, "y"=0.0, "r"=1.0}, "Line Trapping"={"Vector"={"x"=0.0, "y"=0.0, "z"=0.0}, "Phase Gradient"=0.0}, "Amplitude Correction"=0.0} ("Cluster"), w848) -> (w849:T33)
          n1172 = local read "Sequence Storer"() -> (w852:T3[][])
          n1173 = Insert Into Array(array=w852, index (row)=w851, new element=w849) -> (w853:T3[][])  [unwired: 1 in]
          n1174 = local write "Sequence Storer"(w853) -> ()
        }
        n1175 = local write "Initiate Creation"(0) -> ()
      }
    }
    n1176 = Greater?(x=1.0, y=2.0) -> (0:w39:bool)
    n1177 = case shown="True" w39 {
      frame False {
      }
      frame True {
        # "Collision Avoidance System"
        n1178 = local read "Position"() -> (w251:cluster{"x":dbl, "y":dbl, "z":dbl})
        n1179 = local read "1spot X"() -> (w255:dbl)
        n1180 = local read "2spot X"() -> (w262:dbl)
        n1181 = local read "2spot Y"() -> (w260:dbl)
        n1182 = local read "1spot Y"() -> (w257:dbl)
        n1183 = local read "ROI x2"() -> (w261:dbl)
        n1184 = local read "ROI y2"() -> (w259:dbl)
        n1185 = local read "ROI x1"() -> (w254:dbl)
        n1186 = local read "Number of Planned\nSequence Frames"() -> (w266:dbl)
        n1187 = local read "ROI y1"() -> (w256:dbl)
        n1188 = local read "Number of Planned\nSequence Frames"() -> (w265:dbl)
        n1189 = Unbundle(w251) -> ("x"=w252:dbl, "y"=w253:dbl)  [unwired: 1 out]
        n1190 = case shown="3" "Spots" {
          tunnel: w252 -> [_ w350 w352 w354]
          tunnel: w253 -> [_ w349 w351 w353]
          frame 0, Default {
          }
          frame 1 {
            "1spot X" <- w350
            "1spot Y" <- w349
          }
          frame 2 {
            "2spot X" <- w352
            "2spot Y" <- w351
          }
          frame 3 {
            "3spot X" <- w354
            "3spot Y" <- w353
          }
        }
        n1191 = Subtract(x=w261, y=w262) -> (x-y=w263:dbl)
        n1192 = Subtract(x=w259, y=w260) -> (x-y=w264:dbl)
        n1193 = Subtract(x=w254, y=w255) -> (x-y=w267:dbl)
        n1194 = Subtract(x=w256, y=w257) -> (x-y=w258:dbl)
        n1195 = Divide(x=w263, y=w265) -> (x/y=w269:dbl)
        "Step Calculation X2" <- w269
        n1196 = Divide(x=w264, y=w265) -> (x/y=w270:dbl)
        "Step Calculation Y2" <- w270
        n1197 = Divide(x=w267, y=w266) -> (x/y=w268:dbl)
        "Step Calculation X1" <- w268
        n1198 = Divide(x=w258, y=w266) -> (x/y=w271:dbl)
        "Step Calculation Y1" <- w271
        n1199 = while {
          tunnel: w258 -> [w324]
          tunnel: w267 -> [w316]
          tunnel: w268 -> [w294]
          tunnel: w271 -> [w314]
          tunnel: w270 -> [w297]
          tunnel: w269 -> [w298]
          tunnel: w263 -> [w301]
          tunnel: w264 -> [w300]
          tunnel: w265 -> [w299]
          i -> [w274]
          stop <- w283 continue-if-true
          # "Distance Formula"
          # "True if distance is less than the distance limit"
          n1200 = Multiply(x=w301, y=-1) -> (x*y=w304:dbl)
          n1201 = Multiply(x=w300, y=-1) -> (x*y=w309:dbl)
          n1202 = Multiply(x=w316, y=-1) -> (x*y=w315:dbl)
          n1203 = Multiply(x=w324, y=-1) -> (x*y=w321:dbl)
          n1204 = Less?(x=w274, y=w299) -> (x < y?=w273:bool)
          n1205 = Less?(x=w304, y=0) -> (x < y?=w307:bool)
          n1206 = Less?(x=w309, y=0) -> (x < y?=w308:bool)
          n1207 = Add(x=1, y=w274) -> (x+y=w296:i32)
          n1208 = Add(x=1, y=w274) -> (x+y=w293:i32)
          n1209 = Multiply(x=w297, y=w296) -> (x*y=w295:dbl)
          n1210 = Multiply(x=w293, y=w294) -> (x*y=w292:dbl)
          n1211 = Multiply(x=w314, y=w293) -> (x*y=w312:dbl)
          n1212 = Multiply(x=w298, y=w296) -> (x*y=w302:dbl)
          n1213 = Less?(x=w315, y=0) -> (x < y?=w319:bool)
          n1214 = Less?(x=w321, y=0) -> (x < y?=w320:bool)
          n1215 = case shown="True" w308 {
            tunnel: w302 -> [w333 w336]
            tunnel: [w331 w334] -> w275
            frame False {
              n1216 = local read "2spot Y"() -> (w332:dbl)
              n1217 = Subtract(x=w332, y=w333) -> (x-y=w331:dbl)
            }
            frame True {
              n1218 = local read "2spot Y"() -> (w335:dbl)
              n1219 = Add(x=w335, y=w336) -> (x+y=w334:dbl)
            }
          }
          n1220 = case shown="False" w307 {
            tunnel: w295 -> [w326 w329]
            tunnel: [w325 w328] -> w290
            frame False {
              n1221 = local read "2spot X"() -> (w327:dbl)
              n1222 = Subtract(x=w327, y=w326) -> (x-y=w325:dbl)
            }
            frame True {
              n1223 = local read "2spot X"() -> (w330:dbl)
              n1224 = Add(x=w329, y=w330) -> (x+y=w328:dbl)
            }
          }
          n1225 = case shown="False" w320 {
            tunnel: w292 -> [w345 w348]
            tunnel: [w343 w346] -> w291
            frame False {
              n1226 = local read "1spot Y"() -> (w344:dbl)
              n1227 = Subtract(x=w344, y=w345) -> (x-y=w343:dbl)
            }
            frame True {
              n1228 = local read "1spot Y"() -> (w347:dbl)
              n1229 = Add(x=w347, y=w348) -> (x+y=w346:dbl)
            }
          }
          n1230 = case shown="False" w319 {
            tunnel: w312 -> [w338 w341]
            tunnel: [w337 w340] -> w289
            frame False {
              n1231 = local read "1spot X"() -> (w339:dbl)
              n1232 = Subtract(x=w339, y=w338) -> (x-y=w337:dbl)
            }
            frame True {
              n1233 = local read "1spot X"() -> (w342:dbl)
              n1234 = Add(x=w341, y=w342) -> (x+y=w340:dbl)
            }
          }
          n1235 = Subtract(x=w275, y=w291) -> (x-y=w287:dbl)
          n1236 = Subtract(x=w290, y=w289) -> (x-y=w288:dbl)
          n1237 = Square(x=w287) -> (x^2=w286:dbl)
          n1238 = Square(x=w288) -> (x^2=w285:dbl)
          n1239 = local read "Bubble Size"() -> (w278:dbl)
          n1240 = local read "Buffer Zone"() -> (w281:dbl)
          n1241 = Add(x=w286, y=w285) -> (x+y=w284:dbl)
          n1242 = Square Root(x=w284) -> (sqrt(x)=w282:dbl)
          n1243 = Multiply(x=w281, y=2) -> (x*y=w279:dbl)
          n1244 = Add(x=w278, y=w279) -> (x+y=w277:dbl)
          n1245 = Greater?(x=w282, y=w277) -> (0:w276:bool)
          n1246 = Not(x=w276) -> (.not. x?=w272:bool)
          n1247 = And(x=w276, y=w273) -> (x .and. y?=w283:bool)
          n1248 = local write "Possible Collision"(w272) -> ()
        }
      }
    }
    n1249 = local read "Sequence Instances"() -> (w137:dbl)
    n1250 = case shown="True" w156 {
      tunnel: w162 -> [_ w896]
      frame False {
      }
      frame True {
        n1251 = global write "red_tweezers_globals_INTERNAL.vi" "Image Overlay (extras from control loop)"(w896) -> ()
      }
    }
    n1252 = local read "Counter"() -> (w136:dbl)
    n1253 = local read "Sequence Storer"() -> (w132:T3[][])
    n1254 = call "sync_with_globals.vi"("Selection/Group"=w160, "Spots"=w161) -> ("Selection/Group 2"=w172:T9[], "Spots 2"=w123:T3[])  [unwired: 4 in]
    n1255 = local read "Sequence On?"() -> (w135:bool)
    n1256 = local read "Sequence On?"() -> (w150:bool)
    n1257 = call "red_tweezers_UNDO.vi"("Force Save"=w158, "This change is inconsequential (don't save it)"=w159, "Selection/Group"=w160, "Spots"=w161) -> ()  [unwired: 6 in, 2 out]
    n1258 = call "SequenceControl.vi"("Sequence On? 2"=w135, "Counter 2"=w136, "Sequence Instances 2"=w137, "Sequence Storer"=w132) -> ("Time per Frame (ms) 2"=w130:dbl, "Sequence Order 2"=w133:dbl, "Reset 2"=w134:bool, "Sequence Storer 2"=w145:T3[][], "Clearance Button 2"=w144:bool, "Manual Edit 2"=w143:bool, "Save State 2"=w142:bool, "Play Sequence 2"=w139:bool, "Bubble ID to Empty 2"=w138:dbl, "Manual Sequence 2"=w140:bool, "Edit Sequence Mode 2"=w141:bool)  [unwired: 1 in]
    n1259 = local write "Play Sequence"(w139) -> ()
    n1260 = local write "Bubble ID to Empty"(w138) -> ()
    n1261 = local write "Manual Sequence"(w140) -> ()
    n1262 = local write "Reset"(w134) -> ()
    n1263 = local write "Edit Sequence Mode"(w141) -> ()
    n1264 = local write "Clearance Button"(w144) -> ()
    n1265 = local write "Save State"(w142) -> ()
    n1266 = local write "Sequence Storer"(w145) -> ()
    n1267 = local write "Manual Edit"(w143) -> ()
    n1268 = Or(x=w150, y="Manual Sequence") -> (x .or. y?=w149:bool)
    n1269 = case shown="True" "Play Sequence" {
      frame False {
        n1270 = local write "Sequence On?"(FALSE) -> ()
      }
      frame True {
        "Sequence On?" <- TRUE
      }
    }
    n1271 = local write "Time per Frame (ms)"(w130) -> ()
    n1272 = case shown="True" "Clearance Button" {
      frame False {
      }
      frame True {
        # "This is the Bubble ID to Empty tool- this \"deletes\" the bubble in a sequence."
        n1273 = local read "Sequence Order"() -> (w857:dbl)
        n1274 = local read "Sequence Storer"() -> (w858:T3[][])
        n1275 = Replace Array Subset(array=w858, new element=T15 {"Position"={"x"=nan, "y"=nan, "z"=nan}, "Intensity"=1.0, "Vortex Charge"=1, "Phase"=1.0, "NA Position"={"x"=0.0, "y"=0.0, "r"=1.0}, "Line Trapping"={"Vector"={"x"=0.0, "y"=0.0, "z"=0.0}, "Phase Gradient"=0.0}, "Amplitude Correction"=0.0} ("Cluster"), index (row)=w857, index (col)="Bubble ID to Empty") -> (w854:T3[][])
        n1276 = local write "Sequence Storer"(w854) -> ()
      }
    }
    n1277 = feedback #10() -> (w177:T35)  [unwired: 1 out]
    n1278 = call "Smoothed Frame Rate.vi"("Feedback In"=w177) -> ("Feedback Out"=w176:T35, "Frame Rate"=→"Interface Frame Rate":dbl)  [unwired: 1 in, 4 out]
    n1279 = feedback-in #10(w176) -> ()
    n1280 = local write "Sequence Order"(w133) -> ()
    n1281 = Not(x=w126) -> (.not. x?=w127:bool)
    n1282 = Not(x="Output to SLM") -> (.not. x?=w128:bool)
    n1283 = case shown="True" w149 {
      tunnel: [w866 w871] -> w153
      tunnel: w123 -> [w865 _]
      frame False {
        n1284 = Or(x="Manual Edit", y="Edit Sequence Mode") -> (x .or. y?=w864:bool)
        n1285 = case shown="False" w864 {
          tunnel: w865 -> [w867 _]
          tunnel: [w867 w868] -> w866
          frame False {
          }
          frame True {
            n1286 = local read "Sequence Order"() -> (w869:dbl)
            n1287 = local read "Sequence Storer"() -> (w870:T3[][])
            n1288 = Index Array(array=w870, index (row)=w869) -> (element=w868:T3[])  [unwired: 1 in]
          }
        }
      }
      frame True {
        n1289 = stacked-sequence {
          tunnel: [w873 _] -> w871
          frame #0 {
            n1290 = local read "Counter"() -> (w874:dbl)
            n1291 = local read "Sequence Storer"() -> (w875:T3[][])
            n1292 = Index Array(array=w875, index (row)=w874) -> (element=w873:T3[])  [unwired: 1 in]
            n1293 = Wait (ms)(milliseconds to wait="Time per Frame (ms)") -> ()  [unwired: 1 out]
          }
          frame #1 {
            n1294 = local read "Sequence Instances"() -> (w877:dbl)
            n1295 = local read "Counter"() -> (w880:dbl)
            n1296 = Subtract(x=w877, y=1) -> (x-y=w878:dbl)
            n1297 = Equal?(x=w880, y=w878) -> (x = y?=w879:bool)
            n1298 = case shown="False" w879 {
              frame False {
                n1299 = local read "Counter"() -> (w883:dbl)
                n1300 = Add(x=w883, y=1) -> (x+y=→"Counter":dbl)
              }
              frame True {
                w884 = FALSE
                n1301 = local write "Counter"(0) -> ()
                n1302 = local write "Play Sequence"(w884) -> ()
                n1303 = local write "Sequence On?"(w884) -> ()
              }
            }
          }
        }
      }
    }
    n1304 = case shown="True" "Save State" {
      tunnel: w123 -> [_ w887]
      frame False {
      }
      frame True {
        n1305 = local write "Save State"(FALSE) -> ()
        n1306 = stacked-sequence {
          tunnel: w887 -> [w888 _]
          frame #0 {
            "Spot Storage" <- w888
          }
          frame #1 {
            n1307 = local read "Spot Storage"() -> (w894:T3[])
            n1308 = Replace Array Subset(array="Sequence Storer", new element=w894, index (row)="Sequence Order") -> (w892:T3[][])  [unwired: 1 in]
            n1309 = Array Size(array=w892) -> (size(s)=w891:i32[])
            n1310 = local write "Sequence Storer"(w892) -> ()
            n1311 = Index Array(array=w891, index=0) -> (element=→"Sequence Instances":i32)
          }
        }
      }
    }
    n1312 = case shown="True" "Save" {
      frame False {
      }
      frame True {
        n1313 = local read "Sequence Storer"() -> (w823:T3[][])
        n1314 = call "SequenceSaver.vi"("Sequence Storer"=w823) -> ()  [unwired: 10 in, 1 out]
      }
    }
    n1315 = And(x=w128, y=w127) -> (x .and. y?=w131:bool)
    n1316 = case shown="True" "Load" {
      frame False {
      }
      frame True {
        n1317 = call "SequenceSaver.vi"() -> ("Sequence Storer 2"=w822:T3[][])  [unwired: 11 in]
        n1318 = local write "Sequence Storer"(w822) -> ()
      }
    }
    n1319 = case shown="True" w131 {
      tunnel: w123 -> [w2294 _]
      frame False {
        n1320 = call "UDP Sender generic_2.vi"("Spots"=w2294) -> ()  [unwired: 2 in, 1 out]
      }
      frame True {
      }
    }
    n1321 = case shown="True" "Reset" {
      frame False {
      }
      frame True {
        n1322 = local write "Counter"(0) -> ()
      }
    }
    n1323 = local read "Current Spot #"() -> (w106:dbl)
    n1324 = local read "Selection/Group"() -> (w107:T9[])
    n1325 = Not Equal?(x=w106, y=-1) -> (x != y?=w108:bool)
    n1326 = local read "spots selected 2"() -> (w96:i32)
    n1327 = Index Array(array=w107, index=w106) -> (element=w105:T9)
    n1328 = Unbundle By Name(w105) -> ("Selected"=w104:bool)
    n1329 = local read "spots selected"() -> (w97:i32)
    n1330 = Not(x=w104) -> (.not. x?=w103:bool)
    n1331 = And(x=w103, y=w108) -> (x .and. y?=w98:bool)
    n1332 = Less?(x=w97, y=w96) -> (x < y?=w94:bool)
    n1333 = local read "# of Spots"() -> (w122:dbl)
    n1334 = And(x=w94, y=w98) -> (x .and. y?=w99:bool)
    n1335 = case shown="True" w99 {
      frame False {
      }
      frame True {
        n1336 = local read "# of Spots"() -> (w757:dbl)
        n1337 = for {
          N: w757 -> [_]
          i -> [w759]
          stop <- w758 stop-if-true
          n1338 = local read "Selection/Group"() -> (w761:T9[])
          n1339 = Index Array(array=w761, index=w759) -> (element=w760:T9)
          n1340 = Unbundle By Name(w760) -> ("Selected"=w758:bool)
          n1341 = case shown="True" w758 {
            tunnel: w759 -> [_ w763]
            frame False {
            }
            frame True {
              n1342 = local write "Current Spot #"(w763) -> ()
              "Induce check" <- TRUE
            }
          }
        }
      }
    }
    n1343 = case shown="True" "Insert" {
      tunnel: w123 -> [_ w486]
      tunnel: w122 -> [_ w485]
      frame False {
      }
      frame True {
        n1344 = for {
          N: w485 -> [_]
          tunnel: w486 -> [w488]
          i -> [w487]
          n1345 = stacked-sequence {
            tunnel: w488 -> [w490 w495 _]
            tunnel: w487 -> [_ w491 _]
            frame #0 {
              n1346 = local read "Start at Which Frame?"() -> (→"Num":dbl)
              "Spot Storage 2" <- w490
            }
            frame #1 {
              n1347 = local read "Selection/Group"() -> (w494:T9[])
              n1348 = Index Array(array=w494, index=w491) -> (element=w493:T9)
              n1349 = Unbundle By Name(w493) -> ("Selected"=w492:bool)
              n1350 = case shown="True" w492 {
                tunnel: w495 -> [_ _]
                frame False {
                }
                frame True {
                  n1351 = stacked-sequence {
                    frame #0 {
                      n1352 = case shown="\"Arc\"" "Tab Control" {
                        frame "Arc" {
                          n1353 = local read "How Many Frames?"() -> (w497:dbl)
                          n1354 = for {
                            N: w497 -> [_]
                            tunnel: w497 -> [w498]
                            i -> [w500]
                            # "What is this ^\n\nFor # of sequence\nframes, don't worry\nabout it"
                            # "How to make position x and y?\nIt's called a cluster, inser the new position to Position.x and Position.y"
                            n1355 = Equal?(x=w498, y=w500) -> (x = y?=w499:bool)
                            n1356 = case shown="False" w499 {
                              tunnel: [w525 w534] -> w502
                              tunnel: [w524 w533] -> w501
                              tunnel: w500 -> [w521 _]
                              frame False {
                                # "calculating new position"
                                n1357 = local read "Degree Rate"() -> (w520:dbl)
                                n1358 = local read "Original Theta"() -> (w529:dbl)
                                n1359 = Multiply(x=w520, y=w521) -> (x*y=w519:dbl)
                                n1360 = Add(x=w529, y=w519) -> (x+y=w528:dbl)
                                n1361 = Cosine(x=w528) -> (cos(x)=w531:dbl)
                                n1362 = Sine(x=w528) -> (sin(x)=w532:dbl)
                                n1363 = local read "Original Radius"() -> (w530:dbl)
                                n1364 = Multiply(x=w530, y=w532) -> (x*y=w526:dbl)
                                n1365 = Multiply(x=w531, y=w530) -> (x*y=w527:dbl)
                                n1366 = local read "Center X"() -> (w523:dbl)
                                n1367 = local read "Center Y"() -> (w522:dbl)
                                n1368 = Subtract(x=w523, y=w527) -> (x-y=w525:dbl)
                                n1369 = Subtract(x=w522, y=w526) -> (x-y=w524:dbl)
                              }
                              frame True {
                                n1370 = global read "red_tweezers_globals.vi" "Spots"() -> (w537:T3[])
                                n1371 = local read "Numeric"() -> (w536:dbl)
                                n1372 = Index Array(array=w537, index=w536) -> (element=w535:T3)
                                n1373 = Unbundle By Name(w535) -> ("Position.x"=w534:dbl, "Position.y"=w533:dbl)
                              }
                            }
                            n1374 = local read "Spot Storage 2"() -> (w518:T3[])
                            n1375 = local read "Numeric"() -> (w517:dbl)
                            n1376 = Index Array(array=w518, index=w517) -> (element=w504:T3)
                            n1377 = local read "Start at Which Frame?"() -> (w506:dbl)
                            n1378 = Bundle By Name(cluster=w504, "Position.x"=w502, "Position.y"=w501) -> (w503:T3)
                            n1379 = local read "How Many Frames?"() -> (w505:dbl)
                            n1380 = Subtract(x=w506, y=w500) -> (x-y=w515:dbl)
                            n1381 = local read "Sequence Storer"() -> (w516:T3[][])
                            n1382 = local read "Numeric"() -> (w511:dbl)
                            n1383 = Add(x=w515, y=w505) -> (x+y=w514:dbl)
                            n1384 = Subtract(x=w514, y=1) -> (x-y=w512:dbl)
                            n1385 = Replace Array Subset(array=w516, new element=w503, index (row)=w512, index (col)=w511) -> (w510:T3[][])
                            n1386 = Array Size(array=w510) -> (size(s)=w509:i32[])
                            n1387 = local write "Sequence Storer"(w510) -> ()
                            n1388 = Index Array(array=w509, index=0) -> (element=w507:i32)
                            n1389 = local write "Sequence Instances"(w507) -> ()
                          }
                        }
                        frame "Line" {
                          # "This is the automatic sequence generator which allows for the creation of the sequence. This calculates the LAST coordinates of each bubble first\nbefore going for the first few coordinates of the sequence."
                          n1390 = local read "How Many Frames?"() -> (w538:dbl)
                          n1391 = for {
                            N: w538 -> [_]
                            i -> [w546]
                            # "For why do we multiply?"
                            n1392 = local read "Spot Storage 2"() -> (w556:T3[])
                            n1393 = local read "Numeric"() -> (w543:dbl)
                            n1394 = local read "NewXYRates"() -> (w544:dbl[][])
                            n1395 = Index Array(array=w544, index (row)=w543, index (col)=1) -> (element=w539:dbl)
                            n1396 = Index Array(array=w544, index (row)=w543, index (col)=0) -> (element=w540:dbl)
                            n1397 = Index Array(array=w556, index=w543) -> (element=w554:T3)
                            n1398 = Unbundle By Name(w554) -> ("Position.x"=w561:dbl, "Position.y"=w559:dbl)
                            n1399 = Multiply(x=w540, y=w546) -> (x*y=w560:dbl)
                            n1400 = Multiply(x=w539, y=w546) -> (x*y=w555:dbl)
                            "probe" <- w555
                            n1401 = Subtract(x=w561, y=w560) -> (x-y=w558:dbl)
                            n1402 = Subtract(x=w559, y=w555) -> (x-y=w557:dbl)
                            n1403 = Bundle By Name(cluster=w554, "Position.x"=w558, "Position.y"=w557) -> (w549:T3)
                            n1404 = local read "Sequence Storer"() -> (w562:T3[][])
                            n1405 = local read "Numeric"() -> (w548:dbl)
                            n1406 = Add(x="Start at Which Frame?", y=w546) -> (x+y=w545:dbl)
                            n1407 = Replace Array Subset(array=w562, new element=w549, index (row)=w545, index (col)=w548) -> (w553:T3[][])
                            n1408 = Array Size(array=w553) -> (size(s)=w552:i32[])
                            n1409 = local write "Sequence Storer"(w553) -> ()
                            n1410 = Index Array(array=w552, index=0) -> (element=w550:i32)
                            n1411 = local write "Sequence Instances"(w550) -> ()
                          }
                        }
                      }
                    }
                    frame #1 {
                      w564 = FALSE
                      n1412 = Tick Count (ms)() -> (millisecond timer value=→"Stop":u32)
                      n1413 = local write "Play Pressed"(w564) -> ()
                      "Insert End" <- w564
                    }
                  }
                }
              }
              "Numeric" <- w491
            }
            frame #2 {
              n1414 = local write "Insert"(FALSE) -> ()
            }
          }
        }
      }
    }
    n1415 = local read "spots selected"() -> (w109:i32)
    n1416 = local read "spots selected 2"() -> (w110:i32)
    n1417 = local read "Prev Current Spot"() -> (w118:dbl)
    n1418 = local read "Current Spot #"() -> (w119:dbl)
    n1419 = Not Equal?(x=w119, y=w118) -> (x != y?=w117:bool)
    n1420 = Greater?(x=w110, y=w109) -> (0:w111:bool)
    n1421 = local read "Induce check"() -> (w100:bool)
    n1422 = Or(x=w117, y=w111) -> (x .or. y?=w102:bool)
    n1423 = Or(x=w102, y=w100) -> (x .or. y?=w101:bool)
    n1424 = local read "Buffer Zone"() -> (w115:dbl)
    n1425 = case shown="True" w101 {
      frame False {
      }
      frame True {
        n1426 = stacked-sequence {
          frame #0 {
            # "A small 100 ms delay is given to provide enough time for the data to be processed properly."
            n1427 = local read "Null array"() -> (w769:dbl[])
            n1428 = local write "What to Check"(w769) -> ()
            n1429 = local write "ID"(w769) -> ()
            n1430 = local read "Current Spot #"() -> (w771:dbl)
            n1431 = local write "Potential Collisions"(0) -> ()
            n1432 = local read "Spot Checker"() -> (w770:T3[])
            n1433 = Index Array(array=w770, index=w771) -> (element=w772:T3)
            n1434 = Wait (ms)(milliseconds to wait=10) -> ()  [unwired: 1 out]
            n1435 = Unbundle By Name(w772) -> ("Position.x"=w766:dbl, "Position.y"=w767:dbl)
            n1436 = local write "Orig Y SC"(w767) -> ()
            n1437 = local write "Orig X SC"(w766) -> ()
            n1438 = local write "Induce check"(FALSE) -> ()
          }
          frame #1 {
            n1439 = local read "# of Spots"() -> (w773:dbl)
            n1440 = for {
              N: w773 -> [_]
              tunnel: w773 -> [w778]
              i -> [w774]
              n1441 = local read "Selection/Group"() -> (w777:T9[])
              n1442 = Index Array(array=w777, index=w774) -> (element=w776:T9)
              n1443 = Unbundle By Name(w776) -> ("Selected"=w775:bool)
              n1444 = case shown="True" w775 {
                tunnel: w778 -> [_ w780]
                tunnel: w774 -> [_ w779]
                frame False {
                }
                frame True {
                  n1445 = for {
                    N: w780 -> [_]
                    tunnel: w779 -> [w781]
                    i -> [w782]
                    # "If the bubble is not selected, find difference of bubble to bubble\nbeing checked"
                    n1446 = local read "Selection/Group"() -> (w786:T9[])
                    n1447 = Index Array(array=w786, index=w782) -> (element=w785:T9)
                    n1448 = Unbundle By Name(w785) -> ("Selected"=w783:bool)
                    n1449 = Not(x=w783) -> (.not. x?=w784:bool)
                    n1450 = case shown="True" w784 {
                      tunnel: w782 -> [_ w790]
                      tunnel: w781 -> [_ w789]
                      tunnel: w781 -> [_ w788]
                      frame False {
                      }
                      frame True {
                        n1451 = local read "Spot Checker"() -> (w807:T3[])
                        n1452 = Index Array(array=w807, index=w790) -> (element=w808:T3)
                        n1453 = Index Array(array=w807, index=w789) -> (element=w806:T3)
                        n1454 = Unbundle By Name(w806) -> ("Position.x"=w803:dbl, "Position.y"=w799:dbl)
                        n1455 = Unbundle By Name(w808) -> ("Position.x"=w800:dbl, "Position.y"=w796:dbl)
                        n1456 = local read "Area+ Buffer"() -> (w787:dbl)
                        n1457 = Subtract(x=w803, y=w787) -> (x-y=w804:dbl)
                        n1458 = Greater Or Equal?(x=w800, y=w804) -> (x >= y?=w805:bool)
                        n1459 = Add(x=w799, y=w787) -> (x+y=w798:dbl)
                        n1460 = Subtract(x=w799, y=w787) -> (x-y=w797:dbl)
                        n1461 = Add(x=w803, y=w787) -> (x+y=w801:dbl)
                        n1462 = Less Or Equal?(x=w796, y=w798) -> (x <= y?=w795:bool)
                        n1463 = Greater Or Equal?(x=w796, y=w797) -> (x >= y?=w794:bool)
                        n1464 = Less Or Equal?(x=w800, y=w801) -> (x <= y?=w802:bool)
                        n1465 = And(x=w805, y=w802) -> (x .and. y?=w792:bool)
                        n1466 = And(x=w795, y=w794) -> (x .and. y?=w793:bool)
                        n1467 = And(x=w792, y=w793) -> (x .and. y?=w791:bool)
                        n1468 = case shown="True" w791 {
                          tunnel: w790 -> [_ _]
                          tunnel: w790 -> [_ w810]
                          tunnel: w788 -> [_ w809]
                          frame False {
                          }
                          frame True {
                            n1469 = stacked-sequence {
                              tunnel: w810 -> [w811 _]
                              tunnel: w809 -> [w812 _]
                              frame #0 {
                                n1470 = local read "Potential Collisions"() -> (w815:dbl)
                                n1471 = local read "What to Check"() -> (w816:dbl[])
                                n1472 = Insert Into Array(array=w816, index=w815, new element=w811) -> (w817:dbl[])
                                n1473 = local read "ID"() -> (w814:dbl[])
                                n1474 = local write "What to Check"(w817) -> ()
                                n1475 = Insert Into Array(array=w814, index=w815, new element=w812) -> (w813:dbl[])
                                n1476 = local write "ID"(w813) -> ()
                              }
                              frame #1 {
                                n1477 = local read "Potential Collisions"() -> (w820:dbl)
                                n1478 = Add(x=w820, y=1) -> (x+y=w818:dbl)
                                n1479 = local write "Potential Collisions"(w818) -> ()
                              }
                            }
                          }
                        }
                      }
                    }
                  }
                }
              }
            }
          }
          frame #2 {
            n1480 = local read "Current Spot #"() -> (w821:dbl)
            n1481 = local write "Prev Current Spot"(w821) -> ()
          }
        }
      }
    }
    n1482 = Multiply(x=w115, y=2) -> (x*y=w116:dbl)
    n1483 = Add(x="Area to check", y=w116) -> (x+y=→"Area+ Buffer":dbl)
    n1484 = feedback #11() -> (w88:dbl)  [unwired: 1 in]
    n1485 = Equal?(x=w88, y=10000) -> (x = y?=w89:bool)
    n1486 = call "Elapsed Time"("Reset"=w89) -> ("Elapsed Time (s)"=w87:dbl, "Time has Elapsed"=w92:bool)  [unwired: 11 in, 6 out]
    "Elapsed Time" <- w87
    n1487 = feedback-in #11(w87) -> ()
    n1488 = And(x="On", y=w92) -> (x .and. y?=w93:bool)
    n1489 = case shown="True" w93 {
      frame False {
      }
      frame True {
        n1490 = local read "Position"() -> (w756:cluster{"x":dbl, "y":dbl, "z":dbl})
        n1491 = Unbundle By Name(w756) -> ("x"=→"X Pos every 10 sec":dbl)
      }
    }
    n1492 = case shown="True" "OK Button" {
      frame False {
      }
      frame True {
        n1493 = script code="clear all;\nclc;\n\ng = gigecam('169.254.154.83');\n\ng.PixelFormat= 'BayerGR8'\n\nimg = snapshot(g);\n\nimshow(img);"() -> ()  [unwired: 1 in, 1 out]
      }
    }
    n1494 = case shown="True" "O Button" {
      frame False {
      }
      frame True {
        n1495 = script code="%\n    rslt = Hough1_data(img);\n\n    % Frame translation\n    %- omit this as of now \n    \n    % Control method\n    increment = 10; %assuming the diamiter of the agent around 20 pic \n    \n    %- NewLoc = [x,y] whose unit is px\n    %- update new location based on current location obtained by the camera\n    NewLoc(1)= rslt(1);\n    NewLoc(2)= rslt(2);\n    \n    \n    % Update microrobot location with NewLoc\n    % the single robot would move to oblique downword\n    \n    % wait seconds"() -> ("NewLoc"=w752:dbl[])  [unwired: 1 in, 1 out]
        n1496 = Index Array(array=w752, index=1) -> (element=→"Y":dbl)
        n1497 = Index Array(array=w752, index=0) -> (element=→"X":dbl)
      }
    }
  }
  n1498 = flat-sequence {
    tunnel: w6 -> [w2297]
    tunnel: w5 -> [w2296]
    tunnel: [w2295] -> w3
    frame #0 {
      n1499 = disable-structure shown="\"IMAQdx with ROI tool buttons (default)\"" {
        disable-tunnel: w2297 -> [_ _ _ _ _ _]
        disable-tunnel: w2296 -> [_ _ w2355 _ _ _]
        disable-tunnel: [_ _ w2354 _ _ _] -> w2295
        frame condition #0 {
          w2299 = u32 10 ("Number of buffers")
          (unwired) FALSE ("background subtraction")
          # "This subdiagram uses the IMAQ drivers, with a pre-allocated ringbuffer for images.  This is the code I use with my Mikrotron MC1362-CL"
          n1500 = call <vilib>:"IMAQ Init.vi"("Interface Name"="img0") -> ("IMAQ Session Out"=w2306:refnum<k11>)  [unwired: 9 in, 1 out]
          n1501 = call <vilib>:"IMAQ Configure List.vi"("Region of interest"="Global ROI (requires restart)", "Number of buffers"=w2299, "Continuous?"=enum16{"One-Shot", "Continuous"}."Continuous", "IMAQ Session In"=w2306) -> ("error out"=w2300:errorcluster, "IMAQ Session Out"=w2302:refnum<k11>)  [unwired: 6 in]
          n1502 = for {
            N: w2299 -> [_]
            tunnel: 0 ("Channel") -> [w2319]
            shift-right: [w2322] -> w2304
            shift-left: w2300 -> [w2318]
            shift-right: [w2321] -> w2303
            shift-left: w2302 -> [w2320]
            i -> [w2317]
            n1503 = Format Into String(format string="mikrotronbuffer%04d", w2317) -> (resulting string=w2315:string)  [unwired: 2 in, 1 out]
            n1504 = call "IMAQ Create"("Image Name"=w2315) -> ("New Image"=w2314:T11)  [unwired: 4 in, 1 out]
            n1505 = call <vilib>:"IMAQ Configure Buffer.vi"("Channel"=w2319, "error in (no error)"=w2318, "Buffer Number"=w2317, "Image In"=w2314, "IMAQ Session In"=w2320) -> ("error out"=w2322:errorcluster, "IMAQ Session Out"=w2321:refnum<k11>)  [unwired: 5 in]
          }
          n1506 = call <vilib>:"IMAQ Start.vi"("error in (no error)"=w2304, "IMAQ Session In"=w2303) -> ("error out"=w2310:errorcluster, "IMAQ Session Out"=w2311:refnum<k11>)  [unwired: 8 in]
          n1507 = call "IMAQ Create"("Image Name"="Red Tweezers live image") -> ("New Image"=w2312:T11)  [unwired: 3 in, 2 out]
          n1508 = while {
            tunnel: w2311 -> [w2330]
            tunnel: w2310 -> [w2329]
            tunnel: w2312 -> [_]
            tunnel: [w2331] -> w2308
            tunnel: [w2324] -> w2309
            i -> [w2326]
            stop <- w2332 stop-if-true
            n1509 = local read "stop"() -> (w2332:bool)
            n1510 = call <vilib>:"IMAQ Extract Buffer.vi"("error in (no error)"=w2329, "Buffer to extract"=w2326, "IMAQ Session In"=w2330) -> ("error out"=w2324:errorcluster, "Image Out"=w2323:T11, "IMAQ Session Out"=w2331:refnum<k11>)  [unwired: 3 in, 3 out]
            n1511 = call "imageQ_camera_hook.vi"("Image"=w2323) -> ()  [unwired: 11 in]
            n1512 = feedback #12() -> (w2327:T35)  [unwired: 1 in]
            n1513 = call "Smoothed Frame Rate.vi"("Feedback In"=w2327) -> ("Feedback Out"=w2328:T35, "Frame Rate"=w2325:dbl)  [unwired: 1 in, 4 out]
            n1514 = feedback-in #12(w2328) -> ()
            n1515 = global write "red_tweezers_globals_INTERNAL_VOLATILE.vi" "Video Frame Rate"(w2325) -> ()
          }
          n1516 = call <vilib>:"IMAQ Close.vi"("error in (no error)"=w2309, "IMAQ Session In"=w2308) -> ()  [unwired: 9 in, 1 out]
        }
        frame condition #1 {
          (unwired) FALSE ("background subtraction")
          # "This subdiagram acquires using the IMAQdx drivers.  This covers most FireWire and GigE cameras (at least the ones supporting the IIDC or GenICam standards)."
          n1517 = call <vilib>:"IMAQdx Open Camera.vi"("Session In"=T8 "dalsaGenie") -> ("error out"=w2335:errorcluster, "Session Out"=w2334:T8)  [unwired: 9 in]
          n1518 = call <vilib>:"IMAQdx Configure Grab.vi"("error in"=w2335, "Session In"=w2334) -> ("error out"=w2336:errorcluster, "Session Out"=w2337:T8)  [unwired: 8 in]
          n1519 = call "IMAQ Create"("Image Name"="Red Tweezers live image") -> ("New Image"=w2340:T11)  [unwired: 3 in, 2 out]
          n1520 = while {
            tunnel: w2337 -> [w2349]
            tunnel: w2336 -> [w2348]
            tunnel: w2340 -> [w2342]
            tunnel: [w2350] -> w2338
            tunnel: [w2344] -> w2339
            stop <- w2351 stop-if-true
            n1521 = local read "stop"() -> (w2351:bool)
            n1522 = call <vilib>:"IMAQdx Grab.vi"("error in"=w2348, "Image In"=w2342, "Session In"=w2349) -> ("error out"=w2344:errorcluster, "Image Out"=w2343:T11, "Session Out"=w2350:T8)  [unwired: 5 in, 1 out]
            n1523 = call "imageQ_camera_hook.vi"("Image"=w2343) -> ()  [unwired: 11 in]
            n1524 = feedback #13() -> (w2346:T35)  [unwired: 1 in]
            n1525 = call "Smoothed Frame Rate.vi"("Feedback In"=w2346) -> ("Feedback Out"=w2347:T35, "Frame Rate"=w2345:dbl)  [unwired: 1 in, 4 out]
            n1526 = feedback-in #13(w2347) -> ()
            n1527 = global write "red_tweezers_globals_INTERNAL_VOLATILE.vi" "Video Frame Rate"(w2345) -> ()
          }
          n1528 = call <vilib>:"IMAQdx Close Camera.vi"("error in"=w2339, "Session In"=w2338) -> ()  [unwired: 9 in, 1 out]
        }
        frame condition #2 {
          # "This subdiagram acquires using the IMAQdx drivers.  This covers most FireWire and GigE cameras (at least the ones supporting the IIDC or GenICam standards)."
          n1529 = call <vilib>:"IMAQdx Open Camera.vi"("Session In"="Camera") -> ("error out"=w2363:errorcluster, "Session Out"=w2362:T8)  [unwired: 9 in]
          n1530 = call <vilib>:"IMAQdx Configure Grab.vi"("error in"=w2363, "Session In"=w2362) -> ("error out"=w2359:errorcluster, "Session Out"=w2360:T8)  [unwired: 8 in]
          n1531 = call "IMAQ Create"("Image Name"="Red Tweezers live image") -> ("New Image"=w2357:T11)  [unwired: 3 in, 2 out]
          n1532 = call "IMAQdx_get_ROI.vi"("Session In"=w2360) -> ("ROI"=w2356:u32[], "Session Out"=w2358:T8)  [unwired: 8 in]
          n1533 = while {
            shift-right: [w2372] -> w2352
            shift-left: w2359 -> [w2373]
            shift-right: [w2369] -> w2353
            shift-left: w2358 -> [w2370]
            tunnel: w2357 -> [w2368]
            tunnel: w2356 -> [w2367]
            tunnel: w2355 -> [w2366]
            tunnel: [w2365] -> w2354
            stop <- w2379 stop-if-true
            n1534 = event shown="[0] Timeout" {
              selector: _ -> [_ _ _]
              dyn-events: _ -> [_ _ _]
              timeout: 0 -> [_ _ _]
              tunnel: w2373 -> [w2386 w2393 w2408]
              tunnel: [w2385 w2393 w2408] -> w2372
              tunnel: w2370 -> [w2384 w2394 w2409]
              tunnel: [w2383 w2394 w2409] -> w2369
              tunnel: w2368 -> [w2382 _ _]
              tunnel: w2367 -> [w2381 _ _]
              tunnel: w2366 -> [_ w2392 w2407]
              event Timeout {
                w2380 = 0  # timeout in ms
                # "Use a timeout of a few hundred ms if you want to acquire just fast enough to update the image- or a timeout of zero to run the camera at full speed."
                # "This VI sends the image to the loop above for display.\nIt's better to do this than to display here, because it separates the camera loop from the front panel a bit, and increases speed without sacrificing responsiveness of the UI.  Of course, using the event structure removes some of those benefits- but it is possible to write a high-performance camera loop with fast particle tracking, and still use this mechanism to display images without slowing down acquisition."
                # "If we're not dealing with other events, acquire from the camera."
                n1535 = event-data() -> ("Time"=w2391:u32)  [unwired: 1 in]
                n1536 = call <vilib>:"IMAQdx Grab.vi"("error in"=w2386, "Image In"=w2382, "Session In"=w2384) -> ("error out"=w2385:errorcluster, "Image Out"=w2388:T11, "Session Out"=w2383:T8)  [unwired: 5 in, 1 out]
                n1537 = call "IMAQ Clear Overlay"("Image"=w2388) -> ("Image Out"=w2387:T11)  [unwired: 9 in, 1 out]
                n1538 = Multiply(x=w2391, y=u32 1000) -> (x*y=w2389:u32)
                n1539 = call "imageQ_camera_hook.vi"("timeout in ms (0=don't wait if there are no requests)"=w2380, "Timestamp/us"=w2389, "ROI"=w2381, "Image"=w2387) -> ()  [unwired: 8 in]
              }
              event "Draw ROI", "Zoom": Value Change {
                # "This changes the current mouse mode on the image, allowing zooming/drawing of ROI (which can be useful if you want to window down a camera for particle tracking)."
                n1540 = event-data() -> ("CtlRef"=w2399:refnum<vi>)  [unwired: 1 in]
                n1541 = control-ref of="Draw ROI"() -> (w2400:refnum<vi>)
                n1542 = Equal?(x=w2400, y=w2399) -> (x = y?=w2398:bool)
                n1543 = case shown="True" w2398 {
                  tunnel: [w2403 w2406] -> w2397
                  tunnel: [TRUE ("stop") FALSE ("stop")] -> w2395
                  tunnel: [FALSE ("Update Indicators?") TRUE ("Update Indicators?")] -> w2396
                  frame False {
                    w2403 = u32 8 items=["Zoom Tool"=8, "Selection Tool"=0, "Pan Tool"=9, "Point Tool"=1, "Line Tool"=2, "Rectangle Tool"=3, "Rotated Rectangle Tool"=12, "Polyline Tool"=10, "Polygon Tool"=5, "Freehand Tool"=11, "Closed Freehand Tool"=6, "Ellipse Tool"=4, "Annulus Tool"=7] ("Current ROI Tool")
                  }
                  frame True {
                    w2406 = u32 3 items=["Zoom Tool"=8, "Selection Tool"=0, "Pan Tool"=9, "Point Tool"=1, "Line Tool"=2, "Rectangle Tool"=3, "Rotated Rectangle Tool"=12, "Polyline Tool"=10, "Polygon Tool"=5, "Freehand Tool"=11, "Closed Freehand Tool"=6, "Ellipse Tool"=4, "Annulus Tool"=7] ("Current ROI Tool")
                  }
                }
                n1544 = local write "Draw ROI"(w2396) -> ()
                n1545 = local write "Zoom"(w2395) -> ()
                n1546 = property on="Property Node" class="ImageControl"(reference=w2392, "Current ROI Tool"=w2397) -> ()  [unwired: 1 in, 2 out]
              }
              event "Zoom to Fit": Value Change {
                # "The various ROI tools are hidden, so the image control resizes nicely as the Red Tweezers window is resized.  The zoom to fit button/mouse mode buttons return some of this functionality."
                n1547 = event-data() -> ("NewVal"=w2410:bool)  [unwired: 1 in]
                n1548 = property on="Property Node" class="ImageControl"(reference=w2407, "Zoom to Fit Mode"=w2410) -> ()  [unwired: 1 in, 2 out]
              }
            }
            n1549 = feedback #14() -> (w2378:T35)  [unwired: 1 in]
            n1550 = call "Smoothed Frame Rate.vi"("Feedback In"=w2378, "Alpha"=0.05) -> ("Feedback Out"=w2377:T35, "Frame Rate"=w2374:dbl)  [unwired: 4 out]
            n1551 = feedback-in #14(w2377) -> ()
            n1552 = global write "red_tweezers_globals_INTERNAL_VOLATILE.vi" "Video Frame Rate"(w2374) -> ()
            n1553 = local read "stop"() -> (w2375:bool)
            n1554 = Unbundle By Name(w2372) -> ("status"=w2365:bool)
            n1555 = Or(x=w2365, y=w2375) -> (x .or. y?=w2379:bool)
          }
          n1556 = call <vilib>:"IMAQdx Close Camera.vi"("error in"=w2352, "Session In"=w2353) -> ()  [unwired: 9 in, 1 out]
        }
        frame condition #3 (active) {
          w2412 = 0 ("element")
          w2414 = 1920 ("dimension size")
          w2413 = 1080 ("dimension size")
          w2415 = T19 0 items=["Grayscale (U8)", "Grayscale (I16)", "Grayscale (SGL)", "Complex (CSG)", "RGB (U32)", "HSL (U32)", "RGB (U64)", "Grayscale (U16)"] ("Image Type")
          (unwired) FALSE ("background subtraction")
          # "This subdiagram generates a blank white image- useful if you don't have a camera"
          n1557 = Build Array(w2412, w2412, w2414, w2413) -> (w2411:i32[])
          n1558 = Initialize Array(u8 255 ("element"), w2413, w2414) -> (w2416:u8[][])
          n1559 = global write "red_tweezers_globals_INTERNAL.vi" "Global ROI"(w2411) -> ()
          n1560 = call "IMAQ Create"("Image Name"="red tweezers camera stub", "Image Type"=w2415) -> ("New Image"=w2417:T11)  [unwired: 2 in, 2 out]
          n1561 = call "IMAQ ArrayToImage"("Image Pixels (U8)"=w2416, "Image"=w2417) -> ("Image Out"=w2420:T11)  [unwired: 8 in, 1 out]
          n1562 = call "IMAQ Create"("Image Name"="Red Tweezers live image") -> ("New Image"=w2421:T11)  [unwired: 3 in, 2 out]
          n1563 = while {
            tunnel: w2420 -> [w2424]
            tunnel: w2421 -> [_]
            stop <- w2428 stop-if-true
            n1564 = local read "stop"() -> (w2428:bool)
            n1565 = Wait Until Next ms Multiple(millisecond multiple=u32 20) -> ()  [unwired: 1 out]
            n1566 = call "imageQ_camera_hook.vi"("Image"=w2424) -> ()  [unwired: 11 in]
            n1567 = feedback #15() -> (w2426:T35)  [unwired: 1 in]
            n1568 = call "Smoothed Frame Rate.vi"("Feedback In"=w2426) -> ("Feedback Out"=w2427:T35, "Frame Rate"=w2425:dbl)  [unwired: 1 in, 4 out]
            n1569 = feedback-in #15(w2427) -> ()
            n1570 = global write "red_tweezers_globals_INTERNAL_VOLATILE.vi" "Video Frame Rate"(w2425) -> ()
          }
        }
        frame condition #4 {
          # "Use this subdiagram if you have an external camera VI which writes to the image queue (using imageQ_camera_hook.vi)"
        }
        frame condition #5 {
          w2429 = path "C:/Users/Tweezer Cube/Desktop/red_tweezers_1_4_rc0/camera_for_rt136.llb/Particle Tracking.vi"  # Path to camera VI
          # "Use this subdiagram if you have an external camera VI which writes to the image queue (using imageQ_camera_hook.vi).  This is the slightly more sophisticated version, which checks that said external VI is running, and runs it if not."
          n1571 = Open VI Reference(vi path=w2429) -> (vi reference=w2430:refnum<vi>, error out=w2432:errorcluster)  [unwired: 5 in]
          n1572 = property class="VI"(reference=w2430) -> ("Path"=w2431:path)  [unwired: 1 in, 2 out]
          n1573 = global write "red_tweezers_globals_INTERNAL_VOLATILE.vi" "Current Camera VI"(w2431) -> ()
          n1574 = property class="VI"(reference=w2430, error in=w2432) -> (reference out=w2437:refnum<vi>, error out=w2436:errorcluster, "Exec.State"=w2434:T36)
          n1575 = Equal?(x=w2434, y=T36."Idle") -> (x = y?=w2438:bool)
          n1576 = case shown="True" w2438 {
            tunnel: w2437 -> [w2442 w2451]
            tunnel: w2436 -> [w2441 w2448]
            tunnel: [w2440 w2447] -> w2433
            tunnel: w2434 -> [w2444 _]
            frame False {
              n1577 = Close Reference(reference=w2442, error in (no error)=w2441) -> (error out=w2440:errorcluster)
              n1578 = Equal?(x=w2444, y=T36."Bad") -> (x = y?=w2443:bool)
              n1579 = case shown="False" w2443 {
                frame False {
                }
                frame True {
                  n1580 = One Button Dialog(message="The external camera VI is not running and cannot be started- it's probably broken or missing.  Check the static/dynamically loaded VI reference in the bottom loop on the block diagram.") -> ()  [unwired: 1 in, 1 out]
                }
              }
            }
            frame True {
              n1581 = invoke class="VI" method="Run VI"(reference=w2451, error in=w2448, "Wait until done"=FALSE ("Wait Until Done"), "Auto Dispose Ref"=TRUE ("Auto Dispose Reference")) -> (error out=w2447:errorcluster)  [unwired: 1 in, 4 out]
            }
          }
          n1582 = call <vilib>:"Simple Error Handler.vi"("error source (\" \")"="External camera VI (see the bottom loop in the block diagram)" ("error source (\" \")"), "error in (no error)"=w2433) -> ()  [unwired: 3 in, 5 out]
        }
      }
    }
  }
  n1583 = while {
    tunnel: w9 -> [w2469]
    shift-right: [w2468] -> w8
    shift-left: w10 -> [w2470]
    shift-right: [w2465] -> _
    shift-left: _ -> [w2458]
    shift-right: [w2464] -> _
    shift-left: _ -> [w2462]
    shift-right: [w2463] -> _
    shift-left: FALSE ("Saving") -> [w2459]
    stop <- w2467 stop-if-true
    w2456 = u32 50 ("millisecond multiple")
    # "Start/stop saving data, if necessary"
    n1584 = Divide(x=u32 1000, y=w2456) -> (x/y=w2454:dbl)
    n1585 = Wait Until Next ms Multiple(millisecond multiple=w2456) -> ()  [unwired: 1 out]
    n1586 = call "imageQ_dequeue.vi"("timeout in ms (-1)"=2000, "Return queue"=w2470, "Image Dst"=w2469) -> ("Timestamp/us"=w2460:u64, "Return queue out"=w2468:refnum<queue>, "Image Dst Out"=w2471:T11, "timed out?"=w2474:bool, "ROI"=w2453:u64[])  [unwired: 4 in]
    n1587 = Not(x=w2474) -> (.not. x?=w2472:bool)
    n1588 = case shown="True" w2472 {
      tunnel: w2471 -> [_ w2508]
      tunnel: w2462 -> [w2501 w2511]
      tunnel: w2459 -> [_ w2505]
      tunnel: [w2501 w2506] -> w2461
      tunnel: w2460 -> [_ w2509]
      tunnel: w2458 -> [w2502 w2510]
      tunnel: [w2502 w2507] -> w2457
      tunnel: w2453 -> [_ w2504]
      frame False {
      }
      frame True {
        n1589 = global read "red_tweezers_globals_INTERNAL.vi" "Image Overlay (extras from control loop)"() -> (w2519:T21[])
        n1590 = case shown="True" w2505 {
          tunnel: w2511 -> [w2520 w2522]
          tunnel: w2510 -> [w2521 w2528]
          tunnel: w2509 -> [_ w2527]
          tunnel: w2508 -> [_ w2526]
          tunnel: [w2521 w2525] -> w2507
          tunnel: [w2520 w2524] -> w2506
          frame False {
          }
          frame True {
            n1591 = call "save_data_save.vi"("Image"=w2526, "Timestamp"=w2527, "Avi Refnum"=w2522, "Data refnum"=w2528) -> ("error out"=w2523:errorcluster, "Avi Refnum (duplicate)"=w2524:T37, "Data refnum (duplicate)"=w2525:refnum<file>)  [unwired: 5 in]
            n1592 = case shown="Error" w2523 {
              selector: w2523 -> [_ w2530]
              frame No Error {
              }
              frame Error {
                n1593 = call <vilib>:"Clear Errors.vi"("error in (no error)"=w2530) -> ()  [unwired: 5 in, 2 out]
                n1594 = local write "Save Video"(FALSE ("Save")) -> ()
              }
            }
          }
        }
        n1595 = global write "red_tweezers_globals_INTERNAL.vi" "Global ROI"(w2504) -> ()
        n1596 = global read "red_tweezers_globals_INTERNAL_VOLATILE.vi" "Tracked Spot Positions (3D)"() -> (w2512:cluster{"x":dbl, "y":dbl, "Z":dbl}[])
        n1597 = global read "red_tweezers_globals.vi" "Selection/Group"() -> (w2518:T9[])
        n1598 = global read "red_tweezers_globals.vi" "Spots"() -> (w2517:T3[])
        n1599 = call "overlay_positions.vi"("Positions"=w2512, "Image"=w2508) -> ("Image 2"=w2514:T11)  [unwired: 9 in]
        n1600 = call "render_overlay_elements.vi"("Image Overlay (extras from control loop)"=w2519, "Image"=w2514) -> ("Image Out"=w2516:T11)  [unwired: 5 in]
        n1601 = call "grid_and_guides.vi"("Operation"=T16."Render on image", "Image"=w2516) -> ("Image Out"=w2503:T11)  [unwired: 9 in]
        n1602 = call "overlay_spots_on_image.vi"("Selection and Groups"=w2518, "Spots"=w2517, "image"=w2503) -> ("Image"=→"Image":T11)  [unwired: 3 in, 1 out]
      }
    }
    n1603 = global read "red_tweezers_globals_INTERNAL_VOLATILE.vi" "Video Frame Rate"() -> (→"Video Frame Rate":dbl)
    n1604 = case shown="False" "Save Video" {
      tunnel: [w2477 w2492] -> w2465
      tunnel: [w2476 w2486] -> w2464
      tunnel: [FALSE ("Saving") w2491] -> w2463
      tunnel: w2459 -> [w2480 w2490]
      tunnel: w2461 -> [w2478 w2489]
      tunnel: w2457 -> [w2479 w2488]
      tunnel: w2454 -> [_ w2487]
      frame False {
        n1605 = case shown="True" w2480 {
          tunnel: w2479 -> [w2482 w2485]
          tunnel: w2478 -> [w2481 w2484]
          tunnel: [w2482 _] -> w2477
          tunnel: [w2481 _] -> w2476
          frame False {
          }
          frame True {
            n1606 = local write "Save Video"(FALSE ("Save")) -> ()
            n1607 = call "save_data_stop.vi"("Avi Refnum"=w2484, "Data refnum"=w2485) -> ()  [unwired: 10 in]
          }
        }
      }
      frame True {
        n1608 = case shown="False" w2490 {
          selector: w2490 -> [_ w2500]
          tunnel: [w2497 w2498] -> w2492
          tunnel: [w2496 w2499] -> w2486
          tunnel: [w2493 w2500] -> w2491
          tunnel: w2489 -> [_ w2499]
          tunnel: w2488 -> [_ w2498]
          tunnel: w2487 -> [w2495 _]
          frame False {
            n1609 = call "save_data_start.vi"("Save Video"=TRUE, "Frames Per Second"=w2495) -> ("Saving"=w2493:bool, "Avi Refnum"=w2496:T37, "Data Refnum"=w2497:refnum<file>)  [unwired: 3 in]
            n1610 = local write "Save Video"(w2493) -> ()
          }
          frame True {
          }
        }
      }
    }
    n1611 = local read "stop"() -> (w2467:bool)
  }
  n1612 = case shown="True" w3 {
    frame False {
    }
    frame True {
      n1613 = One Button Dialog(message="Warning: there was a camera error.  You may need to restart Red Tweezers.") -> ()  [unwired: 1 in, 1 out]
    }
  }
  n1614 = Release Queue(queue=w8) -> ()  [unwired: 2 in, 3 out]
  n1615 = flat-sequence {
    tunnel: w18 -> [w2536]
    tunnel: w17 -> [_]
    frame #0 {
      # "This autosaves when we stop.  The sequence structures are necessary so that:\n1. loading settings doesn't stop the VI\n2. plugins are still open (and hence saved) when we save settings"
      n1616 = local read "Plugins"() -> (w2539:T5)
      n1617 = global read "red_tweezers_globals_INTERNAL_VOLATILE.vi" "Current Settings File"() -> (w2533:path)
      n1618 = global read "red_tweezers_globals_INTERNAL_VOLATILE.vi" "Save Settings On Exit"() -> (w2532:bool)
      n1619 = flat-sequence {
        tunnel: w2536 -> [w2542]
        tunnel: [w2542] -> w2535
        frame #0 {
          n1620 = local write "stop"(FALSE ("STOP")) -> ()
        }
      }
      n1621 = case shown="True" w2532 {
        tunnel: w2533 -> [_ w2547]
        tunnel: w2535 -> [w2544 w2545]
        tunnel: [w2544 w2545] -> w2534
        frame False {
        }
        frame True {
          n1622 = Path To String(path=w2547) -> (string=w2546:string)
          n1623 = call "settings_save_to_file.vi"("XML File Path"=w2547) -> ()  [unwired: 11 in]
          n1624 = call "settings_filename_to_registry.vi"("Last Used Settings File"=w2546) -> ()  [unwired: 11 in]
        }
      }
      n1625 = flat-sequence {
        tunnel: w2534 -> [w2540]
        tunnel: [w2540] -> _
        frame #0 {
          n1626 = local write "stop"(TRUE ("STOP")) -> ()
        }
      }
      n1627 = control-ref of="Plugin Pnl"() -> (w2537:refnum<vi>)
      n1628 = control-ref of="Plugin:"() -> (w2538:refnum<vi>)
      n1629 = call "plugins_unload.vi"("error in (no error)"=w2534, "Plugins"=w2539, "Sub Panel"=w2537, "Plugin Chooser"=w2538) -> ()  [unwired: 2 in, 2 out]
    }
  }
